vi "Cascade front panel.vi"() -> ()   [LabVIEW 2016]
uses:
  sdi_12/SDI-12/Sonde Vertical Graph.ctl
  controls/Vertical Chart.ctl
  sdi_12/Groundwater header.ctl
  controls/MCC DAQ Setup.ctl
  controls/Aux Sensor.ctl
  KPRO_2016 subvis/Control 2.ctl
  KPRO_2016 subvis/Graph Controls 2.ctl
  KPRO_2016 subvis/Ik control.ctl
  controls/MCC DAQ Readings.ctl
  controls/Kpro pressure measurement cluster.ctl
  controls/Kpro hydraulic measurement cluster.ctl
  activeXtest/activeXtest 2015 Folder/sonde cluster from excel.ctl
  sdi_12/Sonde Value Percent Tol.ctl
  activeXtest/activeXtest 2015 Folder/sample data row cluster.ctl
  activeXtest/activeXtest 2015 Folder/sonde cluster.ctl
  KPRO_2016 subvis/Sensor Physical Measurements.ctl
  KPRO_2016 subvis/SS Control 7.ctl
  controls/Action Control 1.ctl
  <extravilib>/ChannelInstances/One Element Stream-t'Action Control 1.ctl'/Instantiate.vi
  <extravilib>/ChannelInstances/One Element Stream-t'Action Control 1.ctl'/Endpoint.vi
  KPRO_lv2015/Kpro Globals.vi
  <vilib>/Utility/file.llb/Write Delimited Spreadsheet (string).vi
  C/Program Files (x86)/National Instruments/LabVIEW 2016/user.lib/_OpenG.lib/file/file.llb/Strip Path - Traditional__ogtk.vi
  C/Program Files (x86)/National Instruments/LabVIEW 2016/user.lib/_OpenG.lib/file/file.llb/Build Path - Traditional__ogtk.vi
  <vilib>/Utility/file.llb/Write Delimited Spreadsheet (DBL).vi
  C/Program Files (x86)/National Instruments/LabVIEW 2016/user.lib/_OpenG.lib/file/file.llb/Strip Path Extension - Path__ogtk.vi
  C/Program Files (x86)/National Instruments/LabVIEW 2016/user.lib/_OpenG.lib/file/file.llb/Convert File Extension (String)__ogtk.vi
  <vilib>/ULx/Create Channel.llb/ULx Create Channel (AI-Voltage-Basic).vi
  KPRO_lv2015/ad interface/Global_SIM_switch.vi
  C:/Program Files (x86)/National Instruments/LabVIEW 2016/vi.lib/ULx/ULx_LV.dll
  <vilib>/Utility/NIReport.llb/NI_report.lvclass
  <vilib>/Utility/config.llb/NI_LVConfig.lvlib
  <extravilib>/ChannelInstances/One Element Stream-t'Action Control 1.ctl'.lvlib
panel:
  out "output cluster":T1 caption="Cluster" {"Salinity" format="%_3g"; "Temp" format="%_2g"; "ORP" format="%_4g"; "pH" format="%_4g"; "Dissolved\nOxygen" format="%_3g"; "Specific\nConductance" format="%_4g"; "Cumulative\nVolume" format="%#_4g"}
  out "Serial Number/MISC":string
  in  "Depth mode":bool caption="Use \nIncrement"
  in  "Sample Sheet Data Row Cluster 2":T2={"Head\nPressure"=0.0, "Depth"=0.0, "comment string"="", "Sonde Data Cluster"={"Cumulative\nVolume"=100.0, "Specific\nConductance"=2.0, "Dissolved\nOxygen"=3.0, "pH"=4.0, "ORP"=5.0, "Temp"=26.0, "Salinity"=7.0}} {"Sonde Data Cluster"."Salinity" format="%_3g"; "Sonde Data Cluster"."Temp" format="%_2g"; "Sonde Data Cluster"."ORP" format="%_4g"; "Sonde Data Cluster"."pH" format="%_4g"; "Sonde Data Cluster"."Dissolved\nOxygen" format="%_4g"; "Sonde Data Cluster"."Specific\nConductance" format="%_4g"; "Sonde Data Cluster"."Cumulative\nVolume" format="%#_4g"; "Depth" format="%#.3g"; "Head\nPressure" format="%#.4g"}
  out "subarray":string[][](array[string])
  out "Initialization":i32
  in  "Increment Depth":bool
  in  "Finish Tests":bool
  in  "Start KPRO":bool
  in  "Record Continuous Samples":bool
  out "Current Time (s)":dbl
  in  "stop":bool
  in  "Write Data to Spreadsheet":bool
  in  "Sample Not Collected":bool
  in  "Record Single Sample":bool
  in  "Tab Control":T3(tab)
  out "KPRO Output File Path":path=path "C:/KPRO_2010/Output_files/Static Ik.txt"
  out "Output File Path":path=path "C:/KPRO_2010/Output_files/Static Ik.txt"
  in  "Slopes File Path":path=path "D:/Cascade/Data/Output Files/slopes.csv"
  out "12V Voltage Monitor":dbl format="%_3f"
  out "Found Quanta Sonde Com Port":refnum<visa-resource-name>
  in  "Temporary Data Files Directory":path=path "D:/Cascade/Data/Output Files"
  in  "Data File Directory":path=path "D:/Cascade/Data/Excel Reports"
  out "Quanta Sonde found?":bool
  in  "template file path":path=path "D:/Cascade/templates/Groundwater Profiling Log_empty_labview_template.xlsx"
  in  "Config File Path":path=path "D:/Cascade/Data/config files/DAQ Setup Config.ini"
  in  "Read Configuration File?":bool
  out "H-4191 Adapter found":bool
  in  "Save Configuration File?":bool
  out "Sonde Communication Error Out":errorcluster
  in  "Search for Comm Ports?":bool=TRUE
  in  "USB Serial Port Manual Entry":refnum<visa-resource-name>="COM13"
  in  "Static IK path":path=path "D:/Cascade/Data/Output Files/Static Ik.csv"
  out "Down hole Pressure Transducer CSV data  path 2":path
  out "appended path":path
  in  "Sonde Parameters \nTolerance Limits":T4 {"Salinity %" format="%_2f%%"; "Temp %" format="%_2f%%"; "ORP %" format="%_2f%%"; "pH %" format="%_2f%%"; "DO %" format="%_2f%%"; "SC %" format="%_2f%%"}
  in  "Sonde Parameters \nInitial Values":T5 {"Salinity Initial" format="%_2f"; "Temp Initial" format="%_2f"; "ORP  Initial" format="%_2f"; "pH Initial" format="%_2f"; "DO Initial" format="%_2f"; "SC Initial" format="%_2f"}
  in  "Header path":path=path "D:/Cascade/templates/Fields for Excel sheets.xlsx"
  out "Sensor  Real \nMeasurements":T6 {"9V Monitor" format="%#.3g"; "Aux 3" format="%#.3g"; "Aux 2" format="%#.3g"; "Aux 1" format="%#.3g"; "String Pot" format="%#.3g"; "Top String Pot" format="%#_4g"; "Downhole Pressure" format="%#_4g"; "Flow" format="%#_4g"; "Uphole Pressure" format="%#_4g"}
  in  "MCC USB-DAQ Setup":T7={"Device Name in InstaCal"="Dev0", "Omega Pressure Sensor"={"DAQ Channel"=2.0, "Output Voltage Range"=1, "Enabled"=TRUE, "Description"="Uphole Pressure"}, "McMillian 102 Flowmeter"={"DAQ Channel"=11.0, "Output Voltage Range"=0, "Enabled"=TRUE, "Description"="Flow"}, "DHT Pressure Sensor"={"DAQ Channel"=3.0, "Output Voltage Range"=1, "Enabled"=TRUE, "Description"="Downhole Pressure"}, "Top String Pot"={"DAQ Channel"=0.0, "Output Voltage Range"=0, "Enabled"=TRUE, "Description"="Top String Pot"}, "String Pot Signal"={"DAQ Channel"=1.0, "Output Voltage Range"=0, "Enabled"=TRUE, "Description"="String Pot"}, "Aux Sensor 1"={"DAQ Channel"=5.0, "Output Voltage Range"=1, "Enabled"=TRUE, "Description"="Aux 1"}, "Aux Sensor 2"={"DAQ Channel"=6.0, "Output Voltage Range"=1, "Enabled"=TRUE, "Description"="Aux 2"}, "Aux Sensor 3"={"DAQ Channel"=7.0, "Output Voltage Range"=1, "Enabled"=TRUE, "Description"="Aux 3"}, "Voltage Monitor"={"DAQ Channel"=8.0, "Output Voltage Range"=0, "Enabled"=TRUE, "Description"="9V Monitor"}} {"Voltage Monitor"."Output Voltage Range" items=["+/-10 V Range", "+/-5 V Range", "+/-2.5V Range", "+/-1.25 V Range", "+/-0.625 V Range", "+/-0.3125 V Range", "+/-0.1562V Range", "+/-0.078125 V Range"]; "Aux Sensor 3"."Output Voltage Range" items=["+/-10 V Range", "+/-5 V Range", "+/-2.5V Range", "+/-1.25 V Range", "+/-0.625 V Range", "+/-0.3125 V Range", "+/-0.1562V Range", "+/-0.078125 V Range"]; "Aux Sensor 2"."Output Voltage Range" items=["+/-10 V Range", "+/-5 V Range", "+/-2.5V Range", "+/-1.25 V Range", "+/-0.625 V Range", "+/-0.3125 V Range", "+/-0.1562V Range", "+/-0.078125 V Range"]; "Aux Sensor 1"."Output Voltage Range" items=["+/-10 V Range", "+/-5 V Range", "+/-2.5V Range", "+/-1.25 V Range", "+/-0.625 V Range", "+/-0.3125 V Range", "+/-0.1562V Range", "+/-0.078125 V Range"]; "String Pot Signal"."Output Voltage Range" items=["+/-10 V Range", "+/-5 V Range", "+/-2.5V Range", "+/-1.25 V Range", "+/-0.625 V Range", "+/-0.3125 V Range", "+/-0.1562V Range", "+/-0.078125 V Range"]; "Top String Pot"."Output Voltage Range" items=["+/-10 V Range", "+/-5 V Range", "+/-2.5V Range", "+/-1.25 V Range", "+/-0.625 V Range", "+/-0.3125 V Range", "+/-0.1562V Range", "+/-0.078125 V Range"]; "DHT Pressure Sensor"."Output Voltage Range" items=["+/-10 V Range", "+/-5 V Range", "+/-2.5V Range", "+/-1.25 V Range", "+/-0.625 V Range", "+/-0.3125 V Range", "+/-0.1562V Range", "+/-0.078125 V Range"]; "McMillian 102 Flowmeter"."Output Voltage Range" items=["+/-10 V Range", "+/-5 V Range", "+/-2.5V Range", "+/-1.25 V Range", "+/-0.625 V Range", "+/-0.3125 V Range", "+/-0.1562V Range", "+/-0.078125 V Range"]; "Omega Pressure Sensor"."Output Voltage Range" items=["+/-10 V Range", "+/-5 V Range", "+/-2.5V Range", "+/-1.25 V Range", "+/-0.625 V Range", "+/-0.3125 V Range", "+/-0.1562V Range", "+/-0.078125 V Range"]}
  out "Rate":dbl=1000.0 caption="Sample Rate (Hz)"
  out "Number \nof Channels":u16
  in  "Channel \nData Rate S/s":dbl=3720.0 format="%#_13g"
  out "Descriptions":string[](array[string])
  out "Raw Voltages":dbl[](array[numeric])
  out "9V Voltage Monitor":dbl format="%#_3g"
  in  "Record DAQ Raw Voltages":bool
  out "Sensor Voltage Cluster":T9 {"9V Monitor" format="%#.3g"; "Aux 3" format="%#_3g"; "Aux 2" format="%#.3g"; "Aux 1" format="%#.3g"; "String Pot" format="%#.3g"; "Top String Pot" format="%#_3g"; "Downhole Pressure" format="%#.3g"; "Flow" format="%#_3g"; "Uphole Pressure" format="%-#1.3g"}
  in  "Clear Groundwater Header Values":bool
  in  "Groundwater Header":T10
  out "Worksheet Names":string[](array[string])
  in  "Current Sheet":i32=1
  out "row max value":i32
  out "last occupied cell's name":string
  out "Current Sample Sheet":string="Sample 1"
  in  "Excel report file path":path=path "D:/Cascade/Data/Excel Reports/Groundwater Profiling Log_ara1.xlsx"
  out "Data Setup Indicator":string
  in  "Start Initialization":bool
  in  "Input Variables and Slopes":T11={"Total Volume"=0.0, "String Pot Slope"=1.6619999408721924, "Flow Slope"=39.040000915527344, "Up Hole Pressure Slope"=48.27000045776367, "Depth to Water Table"=-0.0, "Atmospheric Pressure"=32.22022530555725, "Reservoir Pressure"=-0.004827000045779073, "Height of Sample Box"=0.0, "DH Pressure Trans Slope"=42.0, "DH Pressure Offset"=0.0, "Up Hole  Pressure Offset"=0.0, "Aux 1 Slope"=1.0, "Aux 2 Slope"=1.0, "Aux 3 Slope"=1.0} {"Aux 3 Slope" format="%.2f"; "Aux 2 Slope" format="%.2f"; "Aux 1 Slope" format="%.2f"; "Up Hole  Pressure Offset" format="%.2f"; "DH Pressure Offset" format="%.2f"; "DH Pressure Trans Slope" format="%.2f"; "Height of Sample Box" format="%.2f"; "Reservoir Pressure" format="%.2f"; "Atmospheric Pressure" format="%.2f"; "Depth to Water Table" format="%.2f"; "Up Hole Pressure Slope" format="%.2f"; "Flow Slope" format="%.2f"; "String Pot Slope" format="%.2f"; "Total Volume" format="%.2f"}
  out "Pressure Offset":dbl
  in  "Update Sonde":bool
  out "Sonde Data Array":T12[](array[typedef]) {"Salinity"."%" format="%_2f%%"; "Salinity"."Value" format="%_4g"; "Temperature"."%" format="%_2f%%"; "Temperature"."Value" format="%_4g"; "ORP"."%" format="%_2f%%"; "ORP"."Value" format="%_4g"; "pH"."%" format="%_2f%%"; "pH"."Value" format="%_4g"; "Dissolved Oxygen"."%" format="%_2f%%"; "Dissolved Oxygen"."Value" format="%_4g"; "Sp. Conductance"."%" format="%_2f%%"; "Sp. Conductance"."Value" format="%_4g"; "Cumulative\nVolume" format="%#_4g"}
  out "Table Label":string="Data from Sample Sheet %d from Excel File"
  out "Sonde Data Display":T14
  out "Temperature":cluster{"Y":dbl[], "Y":dbl[]}[](graph)
  in  "Record Reason":bool
  in  "Select Reasons to Record Data":u16(ring) items=["Per Client Request", "Timed Out", "Sample stopped flowing", "Equipment Issue"]
  out "Sonde Recording Failure Path":path
  out "Sonde IK Behavior Path":path
  out "Recording Reason Sonde array":string[][](array[string])
  out "IK Reason array":string[][](array[string])
  out "SC  Reference\nCalibrate Response":bool
  out "DO  Reference\nCalibrate Response":bool
  in  "Salinity \nReference":dbl
  out "Salinity  Reference\nCalibrate Response":bool
  out "ORP  Reference\nCalibrate Response":bool
  in  "SC \nReference":dbl
  in  "DO \nReference":dbl
  in  "ORP Reference":dbl
  in  "pH Reference":dbl
  in  "pH Zero":dbl
  in  "Record  SC Calibration":bool
  in  "Record DO Calibration":bool
  in  "Record Salinity Calibration":bool
  in  "Record ORP Calibration":bool
  in  "Record pH Calibration Reference":bool
  in  "Record pH Calibration Zero":bool
  out "pH Zero \nCalibrate Response":bool
  out "pH  Reference\nCalibrate Response":bool
  out "KPRO Finish\nIndicator":bool
  in  "Input Depths \nand Parameters Cluster":T16={"Flow"=0.21081600494384767, "Zeroed \nPressure"=74.74207969932556, "Ik"=0.003788962123473114, "Current Depth"=-100.6, "Feet of Stainless"=40, "Start Depth"=0.0, "Abs Start Depth"=0.0} {"Abs Start Depth" format="%.2f"; "Start Depth" format="%.2f"; "Current Depth" format="%.2f"; "Ik" format="%.2f"; "Zeroed \nPressure" format="%.2f"; "Flow" format="%.2f"}
  out "Zero Pressure\nIndicator":bool
  in  "Zero\nPressure":bool caption="Zero Pressure"
  in  "enable_IKMGS_file":bool
  in  "enable_slug_file":bool
  in  "enable_kpro_file":bool=TRUE
  in  "Simulate AD6B":bool
  out "KPRO Test\nIndicator":bool
  in  "Record DTW File":bool
  in  "Zero In-Line Pressure\n(F = leave as is)":bool=TRUE
  out "Current Session":sgl[][](array[numeric]) format="%.2f"
  in  "KPRO test report header":string[](array[string])=["Time(msecs)", "Uncorrected Depth", "Corrected Depth", "Drive_Rate", "Flow", "Feet_of Stainless", "Up Hole Pressure", "IK", "Corrected Pressure", "Atm Pressure", "Depth to water", "Height of box", "Res_Pressure", "Secs_since_1_JAN_1904", "Depth jumps more than 1_foot", "Down hole Pressure"]
  in  "Depth Cluster":T17
  out "Cumulative_data_from_file":sgl[][](array[numeric]) format="%.2f"
  in  "KPRO test report header 2":string[](array[string])=["Time(msecs)", "Uncorrected Depth", "Corrected Depth", "Drive_Rate", "Flow", "Feet_of Stainless", "Up Hole Pressure", "IK", "Corrected Pressure", "Atm Pressure", "Depth to water", "Height of box", "Res_Pressure", "Secs_since_1_JAN_1904", "Depth jumps more than 1_foot", "Down hole Pressure"]
  out "Cumulative_data_ready":bool
  out "Depth Rate\nft/min":dbl format="%#.2g"
  out "Ik":dbl=0.003788962123473114 caption="Real Time - Depth vs. lk" format="%.2f"
  out "Uphole Pressure":dbl format="%.2f"
  in  "New Depth":dbl
  in  "Update Depth":bool
  in  "Select Entry for IK Log File":u16(ring) items=["IK Increase", "IK stayed the Same", "IK decreased"]
  out "Large Depth IK Graph Cluster":T18={[0.003788962123473114, 0.0037174584307500765, 0.0037174584307500765, 0.0037174584307500765, 0.0037174584307500765, 0.003788962123473114], [-100.1, -100.2, -100.3, -100.4, -100.5, -100.6]}
  in  "Culmulative Graph Cluster":T19={"Cumulative - Depth vs. Ik"={[], []}, "Real Time - Depth vs. lk "={[0.003788962123473114, 0.0037174584307500765, 0.0037174584307500765, 0.0037174584307500765, 0.0037174584307500765, 0.003788962123473114], [-100.1, -100.2, -100.3, -100.4, -100.5, -100.6]}, "Cumulative - Depth vs. Drive Rate"={[], []}, "Real Time - Depth vs. Drive Rate"={[0.02036245163917736, 0.125, 0.16666666666666674, 0.16666666666666663, 0.16666666666666663, 0.16666666666666663], [-100.1, -100.2, -100.3, -100.4, -100.5, -100.6]}}
  out "Down hole Pressure":dbl format="%.2f"
  in  "Record IK Reason":bool
  in  "Corrected Pressure Cluster":T20
  out "Flow":dbl format="%#.2g"
  out "Current Depth":sgl=-100.6 format="%.2f"
  out "Current \nDepth (m)":sgl=-30.661383 format="%.2f"
  in  "Read String Pot":bool
  out "Large Depth IK Graph":dbl(graph)
  out "DAQ Error":errorcluster
  out "Initialization Finished":bool=TRUE
  out "Stop":bool
  out "error out":errorcluster
  in  "error in (no error)":errorcluster
  out "producer loop":i32
  out "consumer loop":i32
  out "Active Channel Array":string[](array[string])
  out "delimited string":string
  out "Voltage Range":dbl[](array[numeric])
  out "Stop 2":bool
  # "ft. water"
  # "mL/min."
  # "ft. water"
  # "ft."
  # "ft."
  # "Instructions for Sonde Calibration:\n1.  Use the Record Single Point to Record the Data prior to start of\ncalibration procedure to record the initial points to the excel worksheet.\n2.  pH Calibration is a 2 step process:  A pH standard between 6.8 and 7.2 is treated as the “zero”\nand all other values are treated as the “slope”. First calibrate “zero”, then  add a second to calibrate “slope”. \n3.  Specific Conductance:  Wait for the specific conductance readings to stabilize in the calibration solution, which may\nrequire one or two minutes."
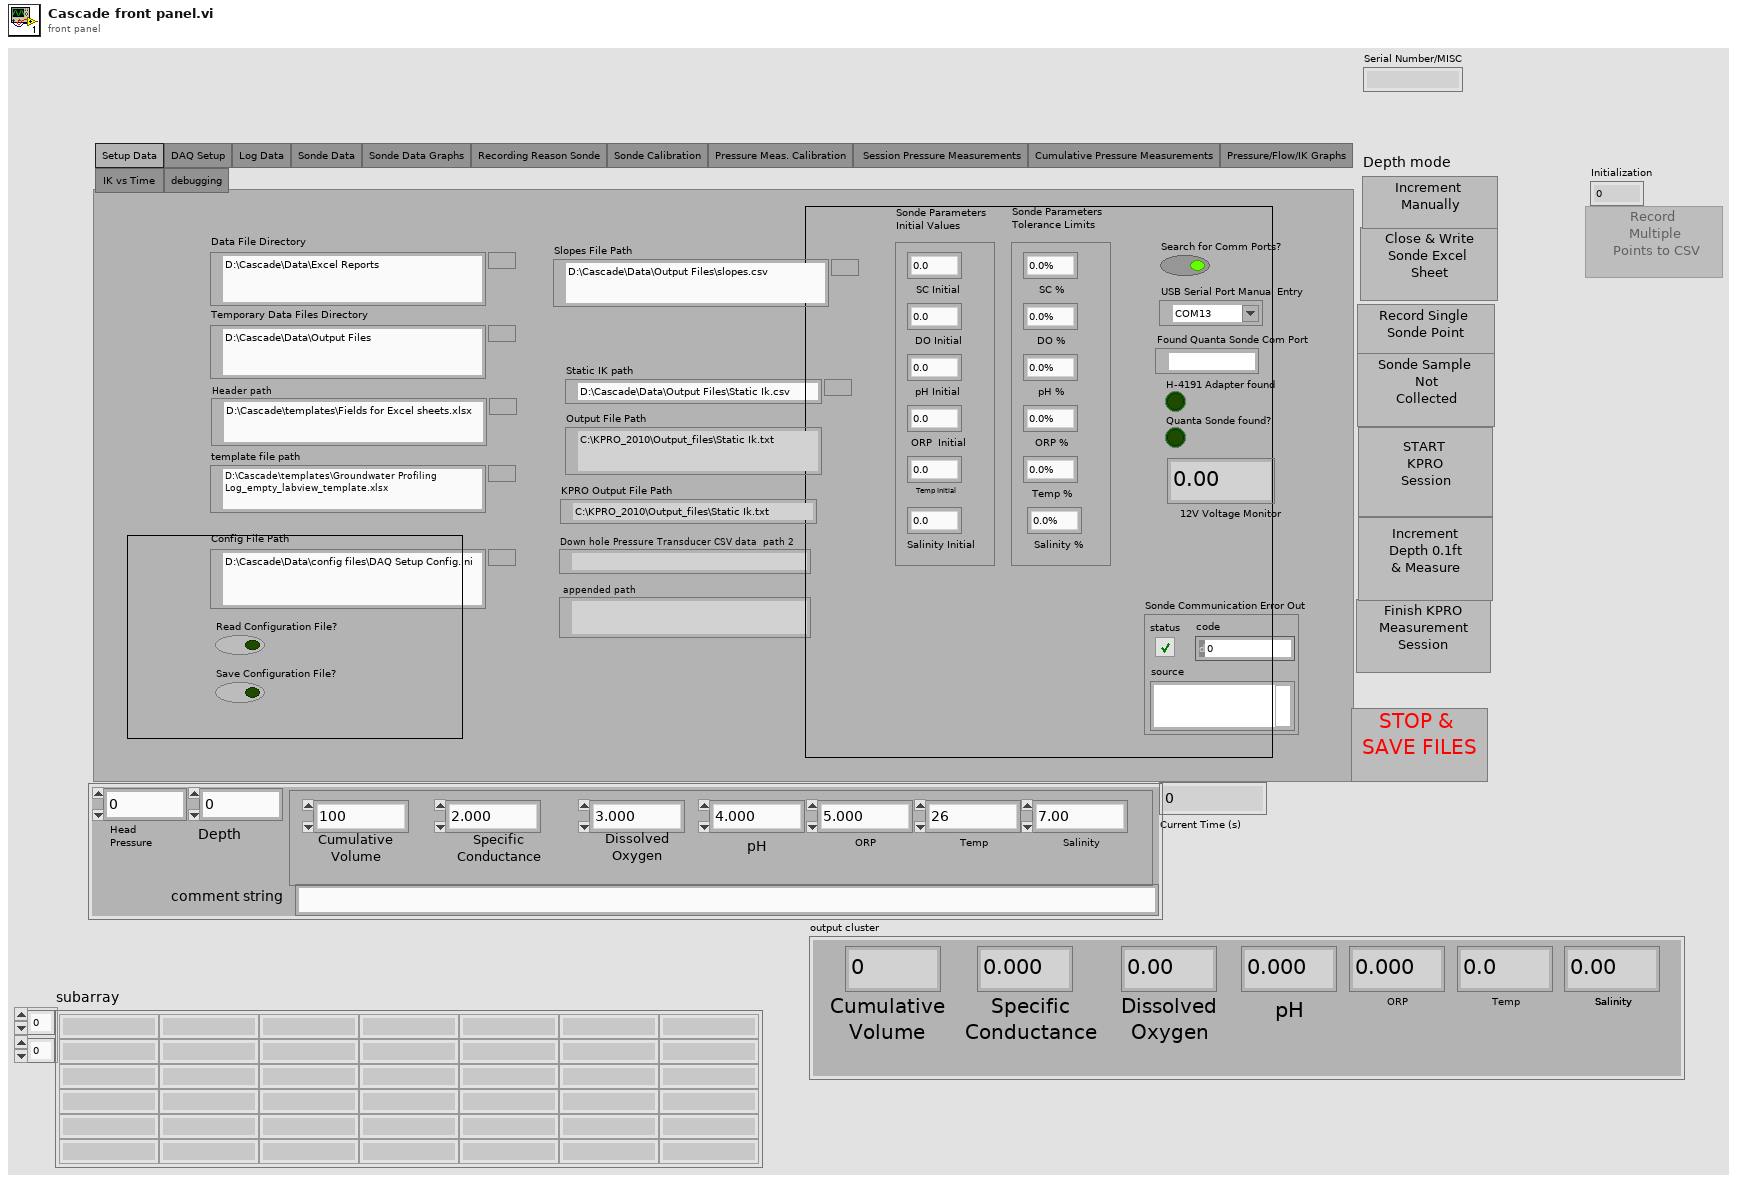
[diagram p1: front panel]
types:
  T1 = typedef "sonde cluster.ctl" = cluster{"Cumulative\nVolume":dbl, "Specific\nConductance":dbl, "Dissolved\nOxygen":dbl, "pH":dbl, "ORP":dbl, "Temp":dbl, "Salinity":dbl}
  T2 = typedef "sample data row cluster.ctl" = cluster{"Head\nPressure":dbl, "Depth":dbl, "comment string":string, "Sonde Data Cluster":T1}
  T3 = enum32{"Setup Data", "DAQ Setup", "Log Data", "Sonde Data", "Sonde Data Graphs", "Recording Reason Sonde", "Sonde Calibration", "Pressure Meas. Calibration", " Session Pressure Measurements", "Cumulative Pressure Measurements", "Pressure/Flow/IK Graphs", "IK vs Time ", "debugging"}
  T4 = cluster{"SC %":dbl, "DO %":dbl, "pH % ":dbl, "ORP % ":dbl, "Temp % ":dbl, "Salinity %":dbl}
  T5 = cluster{"SC Initial ":dbl, "DO Initial ":dbl, "pH Initial  ":dbl, "ORP  Initial":dbl, "Temp Initial":dbl, "Salinity Initial ":dbl}
  T6 = typedef "Sensor Physical Measurements.ctl" = cluster{"Uphole Pressure":dbl, "Flow":dbl, "Downhole Pressure":dbl, "Top String Pot":dbl, "String Pot":dbl, "Aux 1":dbl, "Aux 2":dbl, "Aux 3":dbl, "9V Monitor":dbl}
  T7 = typedef "MCC DAQ Setup.ctl" = cluster{"Device Name in InstaCal":string, "Omega Pressure Sensor":T8, "McMillian 102 Flowmeter":T8, "DHT Pressure Sensor":T8, "Top String Pot":T8, "String Pot Signal":T8, "Aux Sensor 1":T8, "Aux Sensor 2":T8, "Aux Sensor 3":T8, "Voltage Monitor":T8}
  T8 = typedef "Aux Sensor.ctl" = cluster{"DAQ Channel":dbl, "Output Voltage Range":u16, "Enabled":bool, "Description":string}
  T9 = typedef "MCC DAQ Readings.ctl" = cluster{"Uphole Pressure":dbl, "Flow":dbl, "Downhole Pressure":dbl, "Top String Pot":dbl, "String Pot":dbl, "Aux 1":dbl, "Aux 2":dbl, "Aux 3":dbl, "9V Monitor":dbl}
  T10 = typedef "Groundwater header.ctl" = cluster{"Location":string, "Date Finished":string, "CTS":string, "sampler":string, "Kpro box Serial ":string, "Sonde Serial":string, "Drilling Contractor":string, "Ave Depth to Water":string, "Gas/Peri Pump":string, "Atmospheric Pressure":string, "KPRO N2 Pressure":string, "Gas Drive N2 Pressure":string, "Profile ID":string}
  T11 = typedef "Control 2.ctl" = cluster{"Total Volume":dbl, "String Pot Slope":dbl, "Flow Slope":dbl, "Up Hole Pressure Slope":dbl, "Depth to Water Table":dbl, "Atmospheric Pressure":dbl, "Reservoir Pressure":dbl, "Height of Sample Box":dbl, "DH Pressure Trans Slope":dbl, "DH Pressure Offset":dbl, "Up Hole  Pressure Offset":dbl, "Aux 1 Slope":dbl, "Aux 2 Slope":dbl, "Aux 3 Slope":dbl}
  T12 = typedef "sonde cluster from excel.ctl" = cluster{"Head":dbl, "Depth":dbl, "Time":string, "Cumulative\nVolume":dbl, "Sp. Conductance":T13, "Dissolved Oxygen":T13, "pH":T13, "ORP":T13, "Temperature":T13, "Salinity":T13, "Final Tol.":bool, "Final":bool}
  T13 = typedef "Sonde Value Percent Tol.ctl" = cluster{"Value":dbl, "%":dbl, "Tol.":bool}
  T14 = typedef "Sonde Vertical Graph.ctl" = cluster{"pH":T15, "Conductance":T15, "Salinity":T15, "DO % Saturation":T15, "DO mg/L":T15, "ORP":T15}
  T15 = typedef "Vertical Chart.ctl" = cluster{"Y":dbl[], "Y":dbl[]}[]
  T16 = typedef "SS Control 7.ctl" = cluster{"Flow":dbl, "Zeroed \nPressure":dbl, "Ik":dbl, "Current Depth":sgl, "Feet of Stainless":i32, "Start Depth":sgl, "Abs Start Depth":sgl}
  T17 = typedef "Kpro hydraulic measurement cluster.ctl" = cluster{"Absolute Depth In":dbl, "Current Absolute Depth":dbl, "First Absolute Depth":dbl, "Previous Relative Depth":dbl, "Current Relative Depth":dbl, "First Relative Depth":dbl, "Last Filed Depth":dbl, "Total Volume In":dbl, "Total Volume Out":dbl, "Current Measurement Time":dbl, "Previous Measurement Time":dbl}
  T18 = typedef "Ik control.ctl" = cluster{dbl[], dbl[]}
  T19 = typedef "Graph Controls 2.ctl" = cluster{"Cumulative - Depth vs. Ik":cluster{dbl[], dbl[]}, "Real Time - Depth vs. lk ":cluster{dbl[], dbl[]}, "Cumulative - Depth vs. Drive Rate":cluster{dbl[], dbl[]}, "Real Time - Depth vs. Drive Rate":cluster{dbl[], dbl[]}}
  T20 = typedef "Kpro pressure measurement cluster.ctl" = cluster{"Up hole Corrected Pressure":dbl, "Down hole Corrected Pressure":dbl}
  T21 = enum16{"maximized", "minimized", "normal", "no change"}
  T22 = typedef "NI_LVConfig.lvlib/Config Data RefNum.ctl" = refnum<k1>
  T23 = enum8{"Enabled", "Disabled", "Disabled and Grayed Out"}
  T24 = typedef "Action Control 1.ctl" = enum16{"TimeOut", "Continuous  Sonde Data", "Init", "Exit", "Acq. Single Sonde Point", "Write Sonde Sample Sheet", "Acq. DAQ data", "Sample Not Collected", "Record Reason", "pH Calibration Zero", "pH Calibration Standard", "ORP Calibration Standard", "Salinity Calibration Standard", "DO Calibration Standard", "SC Calibration Standard", "Increment Depth Manually", "Start KPRO Measurements", "Finish KPRO Measurements", "Update Depth", "IK vs Time", "Record IK Reason"}
  T25 = typedef "One Element Stream-t'Action Control 1.ctl'.lvlib/)Channel.ctl" = refnum<queue>
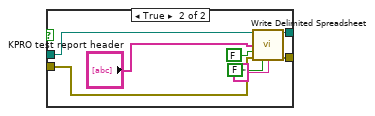
[diagram p11: hidden frame]
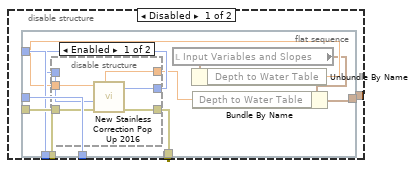
[diagram p18: hidden frame]
diagram:
  # "For calibrate command (XC) on SDI-12 address ‘a’, P is pH, C is specific conductance, S is\nsalinity or TDS, % is DO %Saturation, O is DO mg/L, R is ORP, D is depth, B is\nbarometric pressure, and t is TDS scale factor."
  n1 = flat-sequence {
    tunnel: [w20] -> w5
    tunnel: [w52] -> w7
    tunnel: w5 -> [w52]
    tunnel: [w48] -> w3
    tunnel: [w58] -> w14
    tunnel: w7 -> [w67]
    tunnel: [w67] -> w6
    tunnel: w14 -> [w93]
    tunnel: [w98] -> w12
    tunnel: [w100] -> w11
    tunnel: [w102] -> w8
    tunnel: [w95] -> w9
    tunnel: [w101] -> w10
    tunnel: [w99] -> _
    tunnel: [w94] -> w13
    tunnel: [w96] -> w2
    tunnel: [w97] -> w1
    frame #0 {
      n2 = invoke on="error out" class="Clust (strict)" method="Reinit To Default"(error in="error in (no error)") -> (error out=w18:errorcluster)  [unwired: 2 in, 2 out]
      n3 = flat-sequence {
        tunnel: [w24] -> w20
        tunnel: w18 -> [w23]
        frame #0 {
          n4 = case shown="True" "Read Configuration File?" {
            selector: "Read Configuration File?" -> [_ w31]
            tunnel: [w25 w36] -> w24
            tunnel: w23 -> [w25 w33]
            tunnel: "Config File Path" -> [_ w32]
            frame False {
            }
            frame True {
              n5 = call <vilib>:"Check if File or Folder Exists.vi"("error in (no error)"=w33, "path"=w32) -> ("error out"=w28:errorcluster, "file or folder exists?"=w29:bool, "dup path"=w27:path)  [unwired: 7 in]
              n6 = And(x=w31, y=w29) -> (x .and. y?=w30:bool)
              n7 = control-ref of="This VI"() -> (w34:refnum<vi>)
              n8 = case shown="True" w30 {
                selector: w30 -> [w37 _]
                tunnel: w27 -> [_ w42]
                tunnel: w28 -> [w38 w46]
                tunnel: [w38 w39] -> w35
                tunnel: w34 -> [_ w47]
                frame False {
                  n9 = local write "Read Configuration File?"(w37) -> ()
                }
                frame True {
                  n10 = call <vilib>:"Open Config Data.vi"("error in (no error)"=w46, "create file if necessary (T)"=FALSE, "configuration file path"=w42) -> ("error out"=w44:errorcluster, "refnum"=w45:T22)  [unwired: 6 in, 1 out]
                  n11 = call "Read Panel from INI__ogtk.vi"("error in (no error)"=w44, "VI ref"=w47, "refnum"=w45) -> ("error out"=w40:errorcluster, "refnum out"=w41:T22)  [unwired: 7 in]
                  n12 = call <vilib>:"Close Config Data.vi"("error in (no error)"=w40, "refnum"=w41) -> ("error out"=w39:errorcluster)  [unwired: 8 in, 1 out]
                }
              }
              n13 = call <vilib>:"Clear Errors.vi"("error in (no error)"=w35) -> ("error out"=w26:errorcluster)  [unwired: 5 in, 1 out]
              n14 = Merge Errors(w26) -> (w36:errorcluster)
            }
          }
        }
      }
    }
    frame #1 {
      n15 = local write "Current Sheet"(1 ("Current Sheet")) -> ()
      n16 = Get Date/Time In Seconds() -> (seconds since 1Jan1904=w48:timestamp)
      n17 = Get Date/Time In Seconds() -> (seconds since 1Jan1904=w49:timestamp)
      n18 = Subtract(x=w48, y=w49) -> (x-y=w50:dbl)
      n19 = To Double Precision Float(number=w50) -> (double precision float=→"Current Time (s)":dbl)
    }
    frame #2 {
      w54 = T23."Enabled" ("Disabled")
      w78 = T23."Disabled and Grayed Out" ("Disabled")
      n20 = local write "Initialization Finished"(FALSE ("Initialization Finished")) -> ()
      n21 = invoke on="Current Sheet" class="DigNum (strict)" method="Reinit To Default"() -> (error out=w71:errorcluster)  [unwired: 3 in, 2 out]
      n22 = invoke on="Sample Not Collected" class="Bool" method="Reinit To Default"(error in=w71) -> (error out=w75:errorcluster)  [unwired: 2 in, 2 out]
      n23 = invoke on="Record Continuous Samples" class="Bool" method="Reinit To Default"(error in=w75) -> (error out=w74:errorcluster)  [unwired: 2 in, 2 out]
      n24 = property on="Record Continuous Samples" class="Bool"("DisabledEnum"=w78) -> (error out=w79:errorcluster)  [unwired: 2 in, 1 out]
      n25 = invoke on="Write Data to Spreadsheet" class="Bool" method="Reinit To Default"(error in=w74) -> (error out=w73:errorcluster)  [unwired: 2 in, 2 out]
      n26 = call "search for Quanta Sonde devices.vi"("VISA resource name"="USB Serial Port Manual Entry", "Search for Comm Ports?"="Search for Comm Ports?", "error in (no error)"=w67) -> ("12V monitor"=→"12V Voltage Monitor":dbl, "Com Port with Quanta Sonde devices"=w84:refnum<visa-resource-name>[], "Number of Quanta Sonde devices"=w83:i32, "Serial Number/MISC"=w56:string, "Number of Quanta Sonde devices > 0?"=→"Quanta Sonde found?":bool, "H-4191 Adapter found"=→"H-4191 Adapter found":bool, "Error Out"=w64:errorcluster)  [unwired: 4 in, 2 out]
      "Sonde Communication Error Out" <- w64
      "Serial Number/MISC" <- w56
      n27 = local read "Groundwater Header"() -> (w55:T10)
      n28 = invoke on="Record Single Sample" class="Bool" method="Reinit To Default"(error in=w73) -> (error out=w72:errorcluster)  [unwired: 2 in, 2 out]
      n29 = case shown="1" w83 {
        tunnel: w84 -> [_ w91]
        tunnel: [refnum<visa-resource-name> refnum ("RS232 Port Out") w89] -> w82
        frame 0, Default {
        }
        frame 1 {
          n30 = Index Array(array=w91, index=0) -> (element=w89:refnum<visa-resource-name>)
        }
      }
      "Found Quanta Sonde Com Port" <- w82
      n31 = property on="Record Single Sample" class="Bool"(error in=w79, "DisabledEnum"=w78) -> (error out=w80:errorcluster)  [unwired: 1 in, 1 out]
      n32 = invoke on="stop" class="Bool" method="Reinit To Default"(error in=w72) -> (error out=w77:errorcluster)  [unwired: 2 in, 2 out]
      n33 = Bundle By Name(cluster=w55, "Sonde Serial"=w56) -> (w57:T10)
      n34 = invoke on="Stop" class="Bool (strict)" method="Reinit To Default"() -> (error out=w66:errorcluster)  [unwired: 3 in, 2 out]
      n35 = local write "Groundwater Header"(w57) -> ()
      n36 = property on="Write Data to Spreadsheet" class="Bool"(error in=w77, "DisabledEnum"=w78) -> (error out=w69:errorcluster)  [unwired: 1 in, 1 out]
      n37 = property on="Sample Not Collected" class="Bool"(error in=w80, "DisabledEnum"=w78) -> (error out=w76:errorcluster)  [unwired: 1 in, 1 out]
      n38 = invoke on="Stop 2" class="Bool (strict)" method="Reinit To Default"(error in=w66) -> (error out=w65:errorcluster)  [unwired: 2 in, 2 out]
      n39 = call <vilib>:"Clear Errors.vi"("error in (no error)"=w64) -> ("error out"=w63:errorcluster)  [unwired: 5 in, 1 out]
      n40 = Merge Errors(w63, w65, w69, w76) -> (w60:errorcluster)
      n41 = flat-sequence {
        tunnel: [w87] -> w59
        tunnel: w60 -> [w87]
        frame #0 {
          n42 = local write "Tab Control"(T3."Log Data" ("Tab Control")) -> ()
        }
      }
      n43 = invoke on="Current Session" class="Arr (strict)" method="Reinit To Default"() -> ()  [unwired: 3 in, 3 out]
      n44 = control-ref of="Sonde Data Display"() -> ()  [unwired: 1 out]
      n45 = property on="Clear Groundwater Header Values" class="Bool"("DisabledEnum"=w54) -> ()  [unwired: 2 in, 2 out]
      n46 = property on="Start Initialization" class="Bool"("DisabledEnum"=w54) -> ()  [unwired: 2 in, 2 out]
      n47 = invoke on="Data Setup Indicator" class="Str" method="Reinit To Default"(error in=w59) -> (error out=w58:errorcluster)  [unwired: 2 in, 2 out]
    }
    frame #3 {
      n48 = while {
        tunnel: w93 -> [w108]
        tunnel: [w105] -> w92
        tunnel: [w107] -> _
        i -> [w107]
        stop <- w110 stop-if-true
        n49 = event shown="[1] \"Start Initialization\": Value Change" {
          selector: _ -> [_ _ _]
          dyn-events: _ -> [_ _ _]
          timeout: 100 -> [_ _ _]
          tunnel: [FALSE w118 _] -> w110
          event Timeout {
            n50 = event-data() -> ()  [unwired: 1 in, 3 out]
          }
          event "Start Initialization": Value Change {
            n51 = event-data() -> ()  [unwired: 1 in, 3 out]
            n52 = case shown="True" "Start Initialization" {
              tunnel: [FALSE ("Stop") TRUE ("Stop")] -> w118
              frame False {
              }
              frame True {
                n53 = invoke on="Data Setup Indicator" class="Str" method="Reinit To Default"() -> ()  [unwired: 3 in, 3 out]
                n54 = invoke on="Start Initialization" class="Bool" method="Reinit To Default"() -> ()  [unwired: 3 in, 3 out]
              }
            }
          }
          event "Clear Groundwater Header Values": Value Change {
            n55 = event-data() -> ()  [unwired: 1 in, 6 out]
            n56 = case shown="True" "Clear Groundwater Header Values" {
              frame False {
              }
              frame True {
                n57 = invoke on="Groundwater Header" class="Clust (strict)" method="Reinit To Default"() -> (error out=w122:errorcluster)  [unwired: 3 in, 2 out]
                n58 = flat-sequence {
                  tunnel: w122 -> [_]
                  frame #0 {
                    n59 = local read "Groundwater Header"() -> (w123:T10)
                    n60 = local read "Serial Number/MISC"() -> (w124:string)
                    n61 = Bundle By Name(cluster=w123, "Sonde Serial"=w124) -> (w125:T10)
                    n62 = local write "Groundwater Header"(w125) -> ()
                  }
                }
              }
            }
          }
        }
        n63 = call "Wait (ms)__ogtk.vi"("error in (no error)"=w108, "milliseconds to wait"=u32 100) -> ("error out"=w105:errorcluster)  [unwired: 8 in, 1 out]
        n64 = Quotient & Remainder(x=w107, y=100) -> (floor(x/y)=w103:i32)  [unwired: 1 out]
        n65 = case shown="0" w103 {
          tunnel: w105 -> [w113 w115]
          frame 1, Default {
            n66 = property on="Data Setup Indicator" class="Str"(error in=w113, "Text.TextColor"=u32 0) -> ()  [unwired: 1 in, 2 out]
          }
          frame 0 {
            n67 = property on="Data Setup Indicator" class="Str"(error in=w115, "Text.TextColor"=u32 16716800) -> ()  [unwired: 1 in, 2 out]
          }
        }
        "Data Setup Indicator" <- "Hit the Start Key after Data Entry of Log Parameters and File Names." ("Data Setup Indicator")
      }
      n68 = invoke on="Sonde Data Array" class="Arr (strict)" method="Reinit To Default"() -> ()  [unwired: 3 in, 3 out]
      n69 = flat-sequence {
        tunnel: w92 -> [w146]
        tunnel: [w139] -> w102
        tunnel: [w138] -> w101
        tunnel: [w136] -> w100
        tunnel: [w135] -> w99
        tunnel: [w134] -> w98
        tunnel: [w133] -> w94
        tunnel: [w128] -> w95
        frame #0 {
          w126 = T23."Disabled and Grayed Out" ("Disabled")
          n70 = property on="Clear Groundwater Header Values" class="Bool"("DisabledEnum"=w126) -> ()  [unwired: 2 in, 2 out]
          n71 = property on="Start Initialization" class="Bool"("DisabledEnum"=w126) -> ()  [unwired: 2 in, 2 out]
          n72 = call "get sample header columns.vi"("report file path"="Header path", "error in (no error)"=w146) -> ("Column of Volume"=w128:i32, "Columns"=w138:i32[], "data"=w145:string[][], "error out"=w147:errorcluster)  [unwired: 4 in, 6 out]
          "row max value" <- w128
          n73 = call "format into Sonde Data Array.vi"("data"=w145) -> ()  [unwired: 10 in, 1 out]
          n74 = call "close excel file if open.vi"("error in (no error)"=w147, "report file path in"="Excel report file path") -> ("error out"=w140:errorcluster, "report file path out"=w132:path)  [unwired: 8 in]
          n75 = call "copy excel template.vi"("error in (no error)"=w140, "report file path in"=w132, "template file path in"="template file path") -> ("error out"=w141:errorcluster, "report file path out"=w143:path)  [unwired: 6 in, 1 out]
          n76 = call "open excel get worksheet names.vi"("window state (normal)"=T21."normal", "error in (no error)"=w141, "milliseconds to wait"=u32 5, "report file path"=w143) -> ("error out"=w129:errorcluster, "Number of Sample Sheets"=w139:i32, "NI_report out"=w130:refnum<class "NI_report.lvclass">, "Worksheet Names"=w136:string[])  [unwired: 2 in, 2 out]
          "Worksheet Names" <- w136
          n77 = flat-sequence {
            tunnel: w136 -> [w165]
            tunnel: [w163] -> w135
            tunnel: [w161] -> w134
            tunnel: [w159] -> w133
            tunnel: w130 -> [w158]
            tunnel: w129 -> [w157]
            frame #0 {
              w164 = "Sample 1" ("Worksheet Name in")
              n78 = local read "Current Sample Sheet"() -> (w150:string)
              n79 = call "find and open select worksheet.vi"("Worksheet Names"=w165, "error in (no error)"=w157, "milliseconds to wait"=u32 100, "Worksheet Name in"=w164, "NI_report in"=w158) -> ("error out"=w160:errorcluster, "Select Worksheet Index"=w163:i32, "NI_report out"=w162:refnum<class "NI_report.lvclass">)  [unwired: 4 in]
              n80 = local write "Current Sample Sheet"(w164) -> ()
              n81 = call "get sample sheet data cells.vi"("error in (no error)"=w160, "NI_report in"=w162) -> ("error out"=w153:errorcluster, "data"=w154:string[][], "NI_report out"=w161:refnum<class "NI_report.lvclass">, "left edge output cluster"=w152:cluster{"row":i32, "column":i32})  [unwired: 5 in, 1 out]
              n82 = call "find last occupied cell.vi"("data"=w154, "Active Sheet"=w150, "Header Rows to remove"=3, "sub array start"=w152, "error in (no error)"=w153) -> ("row max value"=w151:i32, "start of last occupied row"=w149:string, "error out"=w159:errorcluster)  [unwired: 4 in, 4 out]
              n83 = Array Subset(array=w154, index (col)=2 ("index")) -> (→"subarray":string[][])  [unwired: 3 in]
              n84 = local write "row max value"(w151) -> ()
              n85 = local write "last occupied cell's name"(w149) -> ()
            }
          }
        }
      }
      n86 = flat-sequence {
        tunnel: w94 -> [_]
        frame #0 {
          n87 = local write "KPRO Finish\nIndicator"(FALSE ("KPRO Finish\nIndicator")) -> ()
        }
      }
      n88 = flat-sequence {
        tunnel: [w169] -> w97
        tunnel: [w169] -> w96
        tunnel: [w174] -> _
        tunnel: w94 -> [w173]
        frame #0 {
          n89 = Unbundle By Name("Input Variables and Slopes") -> ("Depth to Water Table"=w179:dbl)
          n90 = Bundle By Name(cluster="Input Variables and Slopes", "Depth to Water Table"=w179) -> (w176:T11)
          n91 = call <vilib>:"Check if File or Folder Exists.vi"("error in (no error)"=w173, "path"="Slopes File Path") -> ("error out"=w172:errorcluster, "dup path"=w177:path)  [unwired: 7 in, 1 out]
          n92 = case shown="True" TRUE {
            tunnel: w177 -> [_ w190]
            tunnel: w176 -> [w183 w189]
            tunnel: [w183 w188] -> w175
            tunnel: w172 -> [w182 w184]
            tunnel: [w182 w184] -> w174
            frame False {
              n93 = local write "Data Setup Indicator"("Slope file not found." ("Data Setup Indicator")) -> ()
            }
            frame True {
              n94 = call "Get_SLOPE_data_from_file 2016.vi"("Slopes File Path"=w190) -> ("Last_Pressure_Slope"=w185:dbl, "Last_Flow_Slope"=w186:dbl, "Last_String_Pot_Slope"=w187:dbl)  [unwired: 7 in, 1 out]
              n95 = Bundle By Name(cluster=w189, "String Pot Slope"=w187, "Flow Slope"=w186, "Up Hole Pressure Slope"=w185) -> (w188:T11)
            }
          }
          n96 = local read "Input Depths \nand Parameters Cluster"() -> (w171:T16)
          n97 = Unbundle By Name(w171) -> ("Feet of Stainless"=w169:i32)
          n98 = Bundle By Name(cluster=w171, "Feet of Stainless"=w169) -> (w170:T16)
          n99 = local write "Input Depths \nand Parameters Cluster"(w170) -> ()
          n100 = local write "Input Variables and Slopes"(w175) -> ()
        }
      }
      n101 = invoke on="Update Sonde" class="Bool (strict)" method="Reinit To Default"() -> ()  [unwired: 3 in, 3 out]
    }
  }
  n102 = flat-sequence {
    tunnel: [w194] -> w17
    tunnel: w13 -> [w193]
    tunnel: [w192] -> w4
    frame #0 {
      w191 = Action_Control_1."Init"  # Event
      n103 = while {
        shift-right: [w202] -> w194
        shift-left: w193 -> [w202]
        shift-right: [w197] -> _
        shift-left: w191 -> [w195]
        tunnel: [w203] -> w192
        i -> [w201]
        stop <- w199 stop-if-true
        # "User Interface Producer Loop"
        n104 = First Call?() -> (First Call?: T/F=w196:bool)
        n105 = case shown="False" w196 {
          tunnel: w202 -> [w208 _]
          tunnel: [w206 FALSE ("Boolean")] -> w199
          tunnel: [w205 w392] -> w197
          tunnel: w195 -> [_ w392]
          frame False {
            w204 = Action_Control_1."TimeOut"  # Event
            n106 = event shown="[16] \"Record IK Reason\": Value Change" {
              selector: _ -> [_ _ _ _ _ _ _ _ _ _ _ _ _ _ _ _ _ _ _]
              dyn-events: _ -> [_ _ _ _ _ _ _ _ _ _ _ _ _ _ _ _ _ _ _]
              timeout: 100 -> [_ _ _ _ _ _ _ _ _ _ _ _ _ _ _ _ _ _ _]
              tunnel: [w209 w215 w221 w234 w246 w258 w270 w282 w294 w306 w319 w330 w340 w348 w356 w363 w372 w380 _] -> w205
              tunnel: [FALSE w214 w222 w235 w247 w259 w271 w283 w295 w307 w318 w329 w341 w349 w357 w364 w373 w381 _] -> w206
              tunnel: w208 -> [_ w212 w224 w237 w249 w261 w273 w285 w297 w309 _ w326 _ _ _ _ _ _ _]
              tunnel: [_ w212 w223 w236 w248 w260 w272 w284 w296 w308 _ _ _ _ _ _ _ _ _] -> _
              tunnel: w204 -> [w209 w211 w220 w233 w245 w257 w269 w281 w293 w305 w317 w324 w338 w346 w355 w362 w371 w379 _]
              event Timeout {
                n107 = event-data() -> ()  [unwired: 1 in, 3 out]
              }
              event "stop": Value Change {
                n108 = event-data() -> ()  [unwired: 1 in, 6 out]
                n109 = case shown="False" "stop" {
                  tunnel: [w216 w218] -> w215
                  tunnel: [FALSE TRUE] -> w214
                  tunnel: w211 -> [w216 _]
                  frame False {
                  }
                  frame True {
                    w218 = Action_Control_1."Exit"  # Event
                  }
                }
              }
              event "Record DAQ Raw Voltages": Value Change {
                n110 = event-data() -> ()  [unwired: 1 in, 6 out]
                n111 = case shown="False" "Record DAQ Raw Voltages" {
                  tunnel: [w226 w229] -> w221
                  tunnel: [FALSE FALSE ("Boolean")] -> w222
                  tunnel: [w227 w230] -> w223
                  tunnel: w224 -> [w227 w230]
                  tunnel: w220 -> [w226 _]
                  frame False {
                  }
                  frame True {
                    w229 = Action_Control_1."Acq. DAQ data"  # Event
                  }
                }
              }
              event "Record pH Calibration Zero": Value Change {
                n112 = event-data() -> ()  [unwired: 1 in, 6 out]
                n113 = case shown="True" "Record pH Calibration Zero" {
                  tunnel: [w238 w241] -> w234
                  tunnel: [FALSE FALSE ("Boolean")] -> w235
                  tunnel: [w239 w242] -> w236
                  tunnel: w237 -> [w239 w242]
                  tunnel: w233 -> [w238 _]
                  frame False {
                  }
                  frame True {
                    w241 = Action_Control_1."pH Calibration Zero"  # Event
                  }
                }
              }
              event "Record pH Calibration Reference": Value Change {
                n114 = event-data() -> ()  [unwired: 1 in, 6 out]
                n115 = case shown="True" "Record pH Calibration Reference" {
                  tunnel: [w250 w253] -> w246
                  tunnel: [FALSE FALSE ("Boolean")] -> w247
                  tunnel: [w251 w254] -> w248
                  tunnel: w249 -> [w251 w254]
                  tunnel: w245 -> [w250 _]
                  frame False {
                  }
                  frame True {
                    w253 = Action_Control_1."pH Calibration Standard"  # Event
                  }
                }
              }
              event "Record ORP Calibration": Value Change {
                n116 = event-data() -> ()  [unwired: 1 in, 6 out]
                n117 = case shown="True" "Record ORP Calibration" {
                  tunnel: [w262 w265] -> w258
                  tunnel: [FALSE FALSE ("Boolean")] -> w259
                  tunnel: [w263 w266] -> w260
                  tunnel: w261 -> [w263 w266]
                  tunnel: w257 -> [w262 _]
                  frame False {
                  }
                  frame True {
                    w265 = Action_Control_1."ORP Calibration Standard"  # Event
                  }
                }
              }
              event "Record Salinity Calibration": Value Change {
                n118 = event-data() -> ()  [unwired: 1 in, 6 out]
                n119 = case shown="True" "Record Salinity Calibration" {
                  tunnel: [w274 w277] -> w270
                  tunnel: [FALSE FALSE ("Boolean")] -> w271
                  tunnel: [w275 w278] -> w272
                  tunnel: w273 -> [w275 w278]
                  tunnel: w269 -> [w274 _]
                  frame False {
                  }
                  frame True {
                    w277 = Action_Control_1."Salinity Calibration Standard"  # Event
                  }
                }
              }
              event "Record DO Calibration": Value Change {
                n120 = event-data() -> ()  [unwired: 1 in, 6 out]
                n121 = case shown="True" "Record DO Calibration" {
                  tunnel: [w286 w289] -> w282
                  tunnel: [FALSE FALSE ("Boolean")] -> w283
                  tunnel: [w287 w290] -> w284
                  tunnel: w285 -> [w287 w290]
                  tunnel: w281 -> [w286 _]
                  frame False {
                  }
                  frame True {
                    w289 = Action_Control_1."DO Calibration Standard"  # Event
                  }
                }
              }
              event "Record  SC Calibration": Value Change {
                n122 = event-data() -> ()  [unwired: 1 in, 6 out]
                n123 = case shown="True" "Record  SC Calibration" {
                  tunnel: [w298 w301] -> w294
                  tunnel: [FALSE FALSE ("Boolean")] -> w295
                  tunnel: [w299 w302] -> w296
                  tunnel: w297 -> [w299 w302]
                  tunnel: w293 -> [w298 _]
                  frame False {
                  }
                  frame True {
                    w301 = Action_Control_1."SC Calibration Standard"  # Event
                  }
                }
              }
              event "Increment Depth": Value Change {
                n124 = event-data() -> ()  [unwired: 1 in, 6 out]
                n125 = case shown="True" "Increment Depth" {
                  tunnel: [w310 w313] -> w306
                  tunnel: [FALSE FALSE ("Boolean")] -> w307
                  tunnel: [w311 w314] -> w308
                  tunnel: w309 -> [w311 w314]
                  tunnel: w305 -> [w310 _]
                  frame False {
                  }
                  frame True {
                    w313 = Action_Control_1."Increment Depth Manually"  # Event
                  }
                }
              }
              event "Record Single Sample": Value Change {
                n126 = event-data() -> ()  [unwired: 1 in, 6 out]
                n127 = case shown="False" "Record Single Sample" {
                  tunnel: [w320 w322] -> w319
                  tunnel: [FALSE FALSE] -> w318
                  tunnel: w317 -> [w320 _]
                  frame False {
                  }
                  frame True {
                    w322 = Action_Control_1."Acq. Single Sonde Point"  # Event
                  }
                }
              }
              event "Write Data to Spreadsheet": Value Change {
                n128 = event-data() -> ("OldVal"=w328:bool, "NewVal"=w331:bool)  [unwired: 1 in, 4 out]
                n129 = Not(x=w328) -> (.not. x?=w327:bool)
                n130 = And(x=w327, y=w331) -> (x .and. y?=w325:bool)
                n131 = case shown="True" w325 {
                  tunnel: [w332 w335] -> w330
                  tunnel: [FALSE FALSE ("Boolean")] -> w329
                  tunnel: [w333 w336] -> _
                  tunnel: w326 -> [w333 w336]
                  tunnel: w324 -> [w332 _]
                  frame False {
                  }
                  frame True {
                    w335 = Action_Control_1."Write Sonde Sample Sheet"  # Event
                  }
                }
              }
              event "Sample Not Collected": Value Change {
                n132 = event-data() -> ("NewVal"=w339:bool)  [unwired: 1 in, 5 out]
                n133 = case shown="True" w339 {
                  tunnel: [FALSE FALSE] -> w341
                  tunnel: [w342 w344] -> w340
                  tunnel: w338 -> [_ w344]
                  frame True {
                    w342 = Action_Control_1."Sample Not Collected"  # Event
                  }
                  frame False {
                  }
                }
              }
              event "Record Reason": Value Change {
                n134 = event-data() -> ("NewVal"=w347:bool)  [unwired: 1 in, 5 out]
                n135 = case shown="True" w347 {
                  tunnel: [FALSE FALSE] -> w349
                  tunnel: [w350 w352] -> w348
                  tunnel: w346 -> [_ w352]
                  frame True {
                    w350 = Action_Control_1."Record Reason"  # Event
                  }
                  frame False {
                  }
                }
              }
              event "Start KPRO": Value Change {
                n136 = event-data() -> ()  [unwired: 1 in, 6 out]
                n137 = case shown="True" "Start KPRO" {
                  tunnel: [FALSE FALSE] -> w357
                  tunnel: [w358 w360] -> w356
                  tunnel: w355 -> [_ w360]
                  frame True {
                    w358 = Action_Control_1."Start KPRO Measurements"  # Event
                  }
                  frame False {
                  }
                }
              }
              event "Update Depth": Value Change {
                n138 = event-data() -> ()  [unwired: 1 in, 6 out]
                n139 = case shown="True" "Update Depth" {
                  tunnel: [FALSE FALSE] -> w364
                  tunnel: [w366 w368] -> w363
                  tunnel: w362 -> [_ w368]
                  frame True {
                    w366 = Action_Control_1."Update Depth"  # Event
                  }
                  frame False {
                  }
                }
              }
              event "Record IK Reason": Value Change {
                n140 = event-data() -> ()  [unwired: 1 in, 6 out]
                n141 = case shown="True" "Record IK Reason" {
                  tunnel: [FALSE FALSE] -> w373
                  tunnel: [w374 w376] -> w372
                  tunnel: w371 -> [_ w376]
                  frame True {
                    w374 = Action_Control_1."Record IK Reason"  # Event
                  }
                  frame False {
                  }
                }
              }
              event "Finish Tests": Value Change {
                n142 = event-data() -> ()  [unwired: 1 in, 6 out]
                n143 = case shown="True" "Finish Tests" {
                  tunnel: [FALSE FALSE] -> w381
                  tunnel: [w383 w385] -> w380
                  tunnel: w379 -> [_ w385]
                  frame True {
                    w383 = Action_Control_1."Finish KPRO Measurements"  # Event
                    "KPRO Finish\nIndicator" <- TRUE ("KPRO Finish\nIndicator")
                  }
                  frame False {
                  }
                }
              }
              event "Depth mode": Value Change {
                n144 = event-data() -> ()  [unwired: 1 in, 6 out]
                n145 = case shown="True" "Depth mode" {
                  tunnel: [FALSE ("Read String Pot") TRUE ("Read String Pot")] -> w387
                  frame False {
                  }
                  frame True {
                  }
                }
                n146 = local write "Read String Pot"(w387) -> ()
              }
            }
          }
          frame True {
          }
        }
        "Stop" <- w199
        n147 = local read "Stop"() -> (w200:bool)
        n148 = Or(x=w200, y=w199) -> ()  [unwired: 1 out]
        n149 = call <extravilib>:"Write With Abort.vi"("abort"=FALSE, "last element? (F)"=w199, "element"=w197) -> ("channel"=w203:T25)  [unwired: 6 in, 2 out]
        "producer loop" <- w201
      }
    }
  }
  n150 = flat-sequence {
    tunnel: [w418] -> w16
    tunnel: w13 -> [w417]
    tunnel: w12 -> [w416]
    tunnel: w11 -> [w414]
    tunnel: w10 -> [w412]
    tunnel: w9 -> [w411]
    tunnel: w8 -> [w409]
    tunnel: w6 -> [w408]
    tunnel: w4 -> [w407]
    tunnel: w3 -> [w405]
    tunnel: w2 -> [w404]
    tunnel: w1 -> [w403]
    frame #0 {
      w393 = dbl[][] []  # Cumulative Data over 1 string pot
      w397 = T5 {"SC Initial "=0.0, "DO Initial "=0.0, "pH Initial  "=0.0, "ORP  Initial"=0.0, "Temp Initial"=0.0, "Salinity Initial "=0.0}  # Sonde Parameters  Initial Values
      w398 = FALSE  # Read String Pot
      w399 = T16 {"Flow"=0.21081600494384767, "Zeroed \nPressure"=74.74207969932556, "Ik"=0.003788962123473114, "Current Depth"=-100.6, "Feet of Stainless"=40, "Start Depth"=0.0, "Abs Start Depth"=0.0}  # Input Depths  and Parameters Cluster
      w400 = T17 {"Absolute Depth In"=0.0, "Current Absolute Depth"=0.0, "First Absolute Depth"=0.0, "Previous Relative Depth"=0.0, "Current Relative Depth"=0.0, "First Relative Depth"=0.0, "Last Filed Depth"=0.0, "Total Volume In"=0.0, "Total Volume Out"=0.0, "Current Measurement Time"=0.0, "Previous Measurement Time"=0.0}  # Depth Cluster
      w401 = dbl[][] []  # Cumulative Data From File
      n151 = Get Date/Time In Seconds() -> (seconds since 1Jan1904=w396:timestamp)
      n152 = To Double Precision Float(number=w396) -> (double precision float=w395:dbl)
      n153 = while {
        tunnel: w417 -> [w472]
        tunnel: [w473] -> w418
        tunnel: w407 -> [w446]
        tunnel: w416 -> [w471]
        shift-right: [w459] -> _
        shift-left: "Current Sheet" -> [w465]
        tunnel: w414 -> [w461]
        tunnel: w412 -> [w469]
        tunnel: w411 -> [w468]
        shift-right: [w460] -> _
        shift-left: 0 ("row index") -> [w467]
        tunnel: [w466] -> _
        shift-right: [w464] -> _
        shift-left: cluster{"row":i32, "column":i32} {"row"=0, "column"=0} ("start of last occupied row") -> [w463]
        tunnel: w409 -> [w458]
        shift-right: [w452] -> _
        shift-left: dbl[] [] ("Time Array") -> [w453]
        shift-right: [w451] -> _
        shift-left: w401 -> [w450]
        tunnel: w395 -> [w449]
        tunnel: [w448] -> _
        tunnel: w408 -> [w433]
        shift-right: [w444] -> _
        shift-left: refnum<k24>[] [] -> [w432]
        tunnel: w405 -> [w442]
        shift-right: [w419] -> _
        shift-left: w404 -> [w428]
        shift-right: [w441] -> _
        shift-left: w403 -> [w441]
        shift-right: [w438] -> _
        shift-left: w398 -> [w437]
        shift-right: [w424] -> _
        shift-left: w400 -> [w436]
        shift-right: [w435] -> _
        shift-left: w399 -> [w434]
        shift-right: [w429] -> _
        shift-left: w397 -> [_]
        shift-right: [w426] -> _
        shift-left: dbl[][] [] ("Cumulative Sonde \nData Out") -> [w425]
        shift-right: [w423] -> _
        shift-left: w393 -> [w422]
        i -> [w430]
        stop <- w447 stop-if-true
        # "Consumer Data Handling Loop"
        n154 = flat-sequence {
          frame #0 {
            n155 = call "boolean debounce 2016.vi"() -> ()  [unwired: 1 in, 1 out]
          }
        }
        n156 = call <extravilib>:"Read With Abort.vi"("abort"=FALSE, "channel"=w446) -> ("last element?"=w445:bool, "element"=w455:T24)  [unwired: 5 in, 3 out]
        n157 = call "Wait (ms)__ogtk.vi"("error in (no error)"=w472, "milliseconds to wait"=u32 50) -> ("error out"=w457:errorcluster)  [unwired: 8 in, 1 out]
        n158 = feedback-in #1(w455) -> ()
        n159 = feedback #1() -> (w454:T24)  [unwired: 1 in]
        n160 = call "open select sample sheet.vi"("Number of Sample Sheets"=w458, "error in (no error)"=w457, "Worksheet Names"=w461, "Active Sample Sheet"=w465, "NI_report in"=w471) -> ("error out"=w440:errorcluster, "Current Sample Sheet"=w443:string, "NI_report out"=w470:refnum<class "NI_report.lvclass">)  [unwired: 3 in, 1 out]
        n161 = flat-sequence {
          tunnel: w443 -> [w494]
          tunnel: w442 -> [w489]
          tunnel: w440 -> [w488]
          tunnel: [w486] -> w439
          frame #0 {
            n162 = Get Date/Time In Seconds() -> (seconds since 1Jan1904=w490:timestamp)
            n163 = Subtract(x=w490, y=w489) -> (x-y=w491:dbl)
            n164 = local write "Current Time (s)"(w491) -> ()
            n165 = Scan From String(format string="Sample %d", input string=w494, error in=w488) -> (error out=w487:errorcluster, output 1=w492:i32)  [unwired: 2 in, 2 out]
            n166 = Format Into String(format string="Data from Sample Sheet %d from Excel File", error in=w487, w492) -> (resulting string=→"Table Label":string, error out=w486:errorcluster)  [unwired: 1 in]
            "Current Sample Sheet" <- w494
          }
        }
        n167 = disable-structure shown="Enabled" {
          disable-tunnel: w433 -> [w477 _]
          disable-tunnel: w432 -> [w476 w485]
          disable-tunnel: [w475 w485] -> w431
          disable-tunnel: w430 -> [w474 _]
          frame Enabled {
            n168 = case shown="1, Default" w474 {
              tunnel: w476 -> [w478 w484]
              tunnel: w477 -> [_ w483]
              tunnel: [w478 w481] -> w475
              frame 0 {
              }
              frame 1, Default {
                n169 = local read "Descriptions"() -> (w482:string[])
                n170 = call "Measure DAQ Voltages.vi"("error in (no error)"=w483, "Descriptions"=w482, "Array in"=w484) -> ("Raw Voltages"=w480:dbl[], "Array out"=w481:refnum<k24>[], "Sensor Cluster"=w479:T9)  [unwired: 6 in]
                n171 = local write "Sensor Voltage Cluster"(w479) -> ()
                n172 = local write "Raw Voltages"(w480) -> ()
              }
            }
          }
          frame Disabled {
          }
        }
        n173 = feedback #2() -> (w420:i32)  [unwired: 1 in]
        n174 = case shown="\"Start KPRO Measurements\"" w455 {
          selector: w455 -> [_ _ _ _ _ _ _ _ _ _ _ _ _ _ _ _ _ w1955 _ _ _]
          tunnel: w439 -> [w509 w661 w733 w755 w778 w926 w1118 w1135 w1174 w1222 w1257 w1335 w1438 w1542 w1646 w1750 w1853 w1961 w2040 w2418 w2435]
          tunnel: [w509 w661 w733 w755 w774 w921 w1118 w1135 w1174 w1221 w1255 w1333 w1436 w1540 w1644 w1748 w1851 w1944 w2040 w2418 w2445] -> w473
          tunnel: w445 -> [_ _ _ _ _ _ _ _ _ _ _ _ _ _ _ _ _ _ _ _ _]
          tunnel: w470 -> [w526 w647 w732 w754 w795 w946 w1117 w1134 w1173 w1216 w1269 w1353 w1456 w1560 w1664 w1768 w1871 w1962 w2047 w2417 w2436]
          tunnel: [w525 w660 w731 w753 w794 w945 w1116 w1133 w1172 w1215 w1253 w1330 w1433 w1537 w1641 w1745 w1848 w1949 w2046 w2416 w2450] -> w460
          tunnel: w469 -> [_ _ _ _ _ _ _ _ _ _ w1264 w1348 w1451 w1555 w1659 w1763 w1866 _ _ _ _]
          tunnel: w468 -> [_ _ _ _ _ _ _ _ _ _ w1263 w1347 w1450 w1554 w1658 w1762 w1865 _ _ _ _]
          tunnel: w467 -> [w525 w660 w731 w753 w794 w945 w1116 w1133 w1172 w1215 w1233 w1331 w1434 w1538 w1642 w1746 w1849 w1938 w2046 w2416 w2450]
          tunnel: [w526 w647 w732 w754 w795 w946 w1117 w1134 w1173 w1216 w1258 w1336 w1439 w1543 w1647 w1751 w1854 w1960 w2047 w2417 w2451] -> w466
          tunnel: w465 -> [w524 w659 w730 w752 w782 w930 w1115 w1132 w1171 w1214 w1231 w1344 w1447 w1551 w1655 w1759 w1862 w1957 w2045 w2415 w2449]
          tunnel: [w524 w659 w730 w752 w782 w930 w1115 w1132 w1171 w1214 w1231 w1344 w1447 w1551 w1655 w1759 w1862 w1956 w2045 w2415 w2449] -> w459
          tunnel: [w523 w658 w729 w751 w793 w944 w1114 w1131 w1170 w1213 w1254 w1332 w1435 w1539 w1643 w1747 w1850 w1952 w2044 w2414 w2448] -> w464
          tunnel: w463 -> [w523 w658 w729 w751 w793 w944 w1114 w1131 w1170 w1213 _ _ _ _ _ _ _ w1953 w2044 w2414 w2448]
          tunnel: w461 -> [_ _ _ _ _ _ _ _ _ _ _ _ _ _ _ _ _ w1959 _ _ _]
          tunnel: w458 -> [_ _ _ _ _ _ _ _ _ _ _ _ _ _ _ _ _ w1958 _ _ _]
          tunnel: w454 -> [_ _ _ _ _ _ _ _ _ _ _ _ _ _ _ _ _ w1954 _ _ _]
          tunnel: w453 -> [w508 w657 w728 w750 w792 w943 w1113 w1130 w1169 w1212 w1252 w1329 w1432 w1536 w1640 w1744 w1847 w1948 w2043 w2413 w2447]
          tunnel: [w507 w657 w728 w750 w792 w943 w1113 w1130 w1169 w1212 w1251 w1328 w1431 w1535 w1639 w1743 w1846 w1948 w2043 w2413 w2447] -> w452
          tunnel: [w502 w648 w727 w749 w780 w928 w1112 w1129 w1168 w1211 w1250 w1327 w1430 w1525 w1638 w1742 w1845 w1947 w2032 w2412 w2446] -> w451
          tunnel: w450 -> [w503 w648 w727 w749 w786 w935 w1112 w1129 w1168 w1211 w1249 w1326 w1429 w1525 w1637 w1741 w1844 w1947 w2033 w2412 w2446]
          tunnel: w449 -> [_ _ _ _ _ _ _ _ _ _ w1229 w1325 w1428 w1534 w1636 w1740 w1843 _ _ _ _]
          tunnel: w431 -> [w517 w656 w726 w748 w789 w940 w1111 w1128 w1167 w1210 w1247 w1323 w1426 w1532 w1634 w1738 w1841 w1946 _ w2410 w2440]
          tunnel: [w522 w655 w725 w747 w768 w920 w1110 w1127 w1166 w1209 w1248 w1324 w1427 w1533 w1635 w1739 w1842 w1945 w2039 _ w2441] -> w448
          tunnel: w433 -> [w522 w655 w725 w747 w769 w920 w1110 w1127 w1166 w1209 w1248 w1324 w1427 w1533 w1635 w1739 w1842 w1945 w2041 w2409 w2444]
          tunnel: [_ _ _ _ _ _ _ _ _ _ _ _ _ _ _ _ _ _ FALSE ("aborted?") FALSE ("aborted?") w2443] -> w447
          tunnel: [w513 w656 w726 w748 w789 w940 w1111 w1128 w1167 w1210 w1247 w1323 w1426 w1532 w1634 w1738 w1841 w1946 w2030 w2408 w2440] -> w444
          tunnel: [w521 w654 w724 w746 w791 w942 w1109 w1126 w1165 w1208 w1245 w1321 w1424 w1530 w1632 w1736 w1839 w1943 "Read String Pot" w2407 w2439] -> w438
          tunnel: w437 -> [w521 w654 w724 w746 w791 w942 w1109 w1126 w1165 w1208 w1245 w1321 w1424 w1530 w1632 w1736 w1839 w1943 _ w2407 w2439]
          tunnel: [w500 w649 w719 w742 w784 w932 w1108 w1125 w1164 w1207 w1244 w1320 w1423 w1529 w1631 w1735 w1838 w1942 w2036 w2406 w2438] -> w424
          tunnel: w436 -> [w501 w650 w720 w742 w760 w933 w1108 w1125 w1164 w1207 w1244 w1320 w1423 w1529 w1631 w1735 w1838 w1942 w2022 w2406 w2438]
          tunnel: [w520 w653 w723 w745 w790 w941 w1107 w1124 w1163 w1206 w1243 w1319 w1422 w1528 w1630 w1734 w1837 w1941 w2035 w2405 w2437] -> w435
          tunnel: w434 -> [w520 w653 w723 w745 w790 w941 w1107 w1124 w1163 w1206 w1243 w1319 w1422 w1528 w1630 w1734 w1837 w1941 _ w2405 w2437]
          tunnel: [w519 w652 w722 w744 w779 w927 w1106 w1123 w1162 w1205 w1227 w1318 w1421 w1527 w1629 w1733 w1836 w1940 w2026 w2404 w2432] -> w429
          tunnel: "Sonde Parameters \nInitial Values" -> [w519 w652 w722 w744 w779 w927 w1106 w1123 w1162 w1205 w1237 w1318 w1421 w1527 w1629 w1733 w1836 w1940 w2026 w2404 w2432]
          tunnel: w428 -> [w518 w651 w721 w743 w777 w925 w1105 w1122 w1161 w1204 w1236 w1317 w1420 w1526 w1628 w1732 w1835 w1939 w2025 w2403 w2431]
          tunnel: [w518 w651 w721 w743 w762 w924 w1105 w1122 w1161 w1204 w1236 w1317 w1420 w1526 w1628 w1732 w1835 w1939 w2025 w2403 w2431] -> w421
          tunnel: [w506 w646 w718 w741 w761 w918 w1104 w1121 w1160 w1203 w1228 w1316 w1419 w1524 w1627 w1731 w1834 w1937 w2023 w2402 w2430] -> w426
          tunnel: w425 -> [w505 w646 w718 w741 w761 w918 w1104 w1121 w1160 w1203 w1228 w1316 w1419 w1523 w1627 w1731 w1834 w1937 w2023 w2402 w2430]
          tunnel: [w498 w645 w717 w740 w757 w917 w1103 w1120 w1159 w1202 w1226 w1315 w1418 w1522 w1626 w1730 w1833 w1936 w2020 w2401 w2429] -> w423
          tunnel: w422 -> [w499 w645 w717 w740 w758 w916 w1103 w1120 w1159 w1202 w1226 w1315 w1418 w1522 w1626 w1730 w1833 w1936 w2020 w2401 w2429]
          tunnel: w420 -> [w497 w643 w716 w739 w756 w915 w1101 w1119 w1158 w1201 w1225 w1314 w1417 w1521 w1625 w1729 w1832 w1935 w2019 w2400 w2428]
          tunnel: [w497 w642 w716 w739 w756 w915 w1101 w1119 w1158 w1201 w1225 w1314 w1417 w1521 w1625 w1729 w1832 w1935 w2019 w2400 w2428] -> w419
          frame "TimeOut", Default {
            n175 = flat-sequence {
              tunnel: [w628] -> _
              tunnel: [w633] -> w510
              tunnel: [w641] -> _
              tunnel: [w640] -> _
              tunnel: w517 -> [w639]
              tunnel: [w638] -> _
              frame #0 {
                n176 = local read "Input Variables and Slopes"() -> (w630:T11)
                n177 = local read "Input Variables and Slopes"() -> (w635:T11)
                n178 = local read "Zero In-Line Pressure\n(F = leave as is)"() -> (w634:bool)
                n179 = Unbundle By Name(w635) -> ("DH Pressure Trans Slope"=w641:dbl, "DH Pressure Offset"=w640:dbl)
                n180 = local read "Sensor Voltage Cluster"() -> (w636:T9)
                n181 = local read "Descriptions"() -> (w637:string[])
                n182 = local read "Sensor  Real \nMeasurements"() -> (w632:T6)
                n183 = global read "Kpro Globals.vi" "Current Depth"() -> (w628:sgl)
                n184 = call "DHT Pressure 2016.vi"("Sensor Cluster"=w636, "DHT Pressure Offset"=w640, "Array in"=w639, "DHT Pressure \nSlope"=w641, "Descriptions"=w637, "Zero Pressure\n(F = leave as is)"=w634) -> ("Array out"=w638:refnum<k24>[], "DHT Pressure"=w633:dbl, "Sensor Cluster 2"=w629:T9)  [unwired: 7 in]
                n185 = local write "Sensor Voltage Cluster"(w629) -> ()
                n186 = call "convert sensor voltage to real measurements.vi"("Input Variables and Slopes"=w630, "Sensor  Real Measurements in"=w632, "Sensor Cluster"=w629) -> ("Sensor  Real Measurements out"=w631:T9)  [unwired: 8 in]
                n187 = local write "Sensor  Real \nMeasurements"(w631) -> ()
                n188 = local write "Down hole Pressure"(w633) -> ()
                n189 = Add(x=w633, y=w628) -> ()  [unwired: 1 out]
              }
            }
            n190 = case shown="True" "Update Sonde" {
              tunnel: w508 -> [w528 w535]
              tunnel: [w528 w534] -> w507
              tunnel: [w527 w533] -> w506
              tunnel: w505 -> [w527 w532]
              frame False {
              }
              frame True {
                n191 = local read "Sonde Communication Error Out"() -> (w531:errorcluster)
                n192 = local read "Current Time (s)"() -> (w529:dbl)
                n193 = flat-sequence {
                  tunnel: w531 -> [w553]
                  tunnel: [w552] -> w530
                  tunnel: w535 -> [w551]
                  tunnel: [w550] -> w534
                  tunnel: [w549] -> w533
                  tunnel: w532 -> [w548]
                  tunnel: [w538] -> _
                  tunnel: [w547] -> _
                  tunnel: w529 -> [w546]
                  frame #0 {
                    n194 = local read "Sample Sheet Data Row Cluster 2"() -> (w539:T2)
                    n195 = control-ref of="Found Quanta Sonde Com Port"() -> (w545:refnum<vi>)
                    n196 = control-ref of="Current Time (s)"() -> (w541:refnum<vi>)
                    n197 = control-ref of="Sonde Data Display"() -> (w544:refnum<vi>)
                    n198 = control-ref of="Sonde Data Display"() -> (w543:refnum<vi>)
                    n199 = control-ref of="Temperature"() -> (w542:refnum<vi>)
                    n200 = Unbundle By Name(w539) -> ("Sonde Data Cluster.Cumulative\nVolume"=w536:dbl)
                    n201 = call "Sonde Single Measurement Subvi.vi"("VISAResourceName in"=w545, "Time Array"=w551, "Cumulative Sonde Data"=w548, "Previous time"=w546, "Sonde Data Display"=w544, "Sonde Graph in"=w543, "Temp Graph 3"=w542, "error in (no error)"=w553, "Row Cluster Input"=w539, "reference 5"=w541) -> ("seconds since 1Jan1904"=w547:timestamp, "Cumulative Sonde \nData Out"=w549:dbl[][], "Sample Sheet Data Row Cluster 2"=w538:T2, "output cluster"=w540:T1, "time array out"=w550:dbl[], "error out"=w552:errorcluster)
                    n202 = Bundle By Name(cluster=w538, "Sonde Data Cluster.Cumulative\nVolume"=w536) -> (w537:T2)
                    n203 = local write "Sample Sheet Data Row Cluster 2"(w537) -> ()
                    n204 = local write "output cluster"(w540) -> ()
                  }
                }
                n205 = local write "Sonde Communication Error Out"(w530) -> ()
              }
            }
            n206 = flat-sequence {
              tunnel: w517 -> [w622]
              tunnel: [w618] -> w516
              tunnel: [w617] -> w515
              frame #0 {
                n207 = local read "Input Variables and Slopes"() -> (w625:T11)
                n208 = Unbundle By Name(w625) -> ("Up Hole Pressure Slope"=w624:dbl, "Up Hole  Pressure Offset"=w621:dbl)
                n209 = local write "Input Variables and Slopes"(w625) -> ()
                n210 = local read "Sensor Voltage Cluster"() -> (w626:T9)
                n211 = local read "Descriptions"() -> (w618:string[])
                n212 = local read "Corrected Pressure Cluster"() -> (w620:T20)
                n213 = call "up hole Pressure 2016.vi"("Sensor Cluster"=w626, "Pressure Offset"=w621, "Array in"=w622, "Pressure \nSlope"=w624, "Descriptions"=w618, "Zero Pressure\n(F = leave as is)"=TRUE) -> ("Array out"=w617:refnum<k24>[], "Uphole Pressure"=w616:dbl, "Sensor Cluster 2"=w623:T9)  [unwired: 7 in]
                n214 = local write "Uphole Pressure"(w616) -> ()
                n215 = Bundle By Name(cluster=w620, "Up hole Corrected Pressure"=w616) -> (w619:T20)
                n216 = local write "Sensor Voltage Cluster"(w623) -> ()
                n217 = local write "Corrected Pressure Cluster"(w619) -> ()
              }
            }
            n218 = flat-sequence {
              tunnel: w516 -> [w609]
              tunnel: w515 -> [w612]
              tunnel: [w608] -> w512
              tunnel: [w609] -> w514
              tunnel: [w605] -> w511
              tunnel: [w607] -> w513
              frame #0 {
                w613 = 0.0  # Offset
                n219 = local read "Input Variables and Slopes"() -> (w611:T11)
                n220 = local read "Input Depths \nand Parameters Cluster"() -> (w604:T16)
                n221 = Unbundle By Name(w611) -> ("Flow Slope"=w610:dbl)
                n222 = local read "Input Depths \nand Parameters Cluster"() -> (w615:T16)
                n223 = Unbundle By Name(w604) -> ("Feet of Stainless"=w603:i32)
                n224 = call "Flow 2016.vi"("Descriptions"=w609, "Array in"=w612, "Flow Slope"=w610, "Offset"=w613) -> ("Sensor Cluster"=w608:T9, "Flow (ml/min)"=w605:dbl, "Array out"=w607:refnum<k24>[])  [unwired: 4 in]
                n225 = local write "Sensor Voltage Cluster"(w608) -> ()
                n226 = call "pressure and IK2 2016.vi"("Ft. of SS"=w603, "flow"=w605) -> ("IK"=→"Large Depth IK Graph":dbl)  [unwired: 1 in, 1 out]
                n227 = Bundle By Name(cluster=w615, "Flow"=w605) -> (w614:T16)
                n228 = local write "Input Depths \nand Parameters Cluster"(w614) -> ()
              }
            }
            n229 = flat-sequence {
              tunnel: w514 -> [w591]
              tunnel: w503 -> [w564]
              tunnel: w512 -> [w590]
              tunnel: w501 -> [w569]
              tunnel: [w589] -> w500
              tunnel: w511 -> [w588]
              tunnel: w513 -> [w579]
              tunnel: [w578] -> _
              tunnel: [w556] -> w502
              tunnel: [w570] -> _
              tunnel: w510 -> [w561]
              tunnel: w509 -> [w558]
              tunnel: w499 -> [w557]
              tunnel: [w554] -> w498
              frame #0 {
                # "Timeout"
                n230 = Unbundle By Name(w569) -> ("Current Relative Depth"=w568:dbl)
                n231 = local read "Input Depths \nand Parameters Cluster"() -> (w583:T16)
                n232 = local read "Culmulative Graph Cluster"() -> (w577:T19)
                n233 = local read "Depth mode"() -> (w566:bool)
                n234 = local read "Input Variables and Slopes"() -> (w587:T11)
                n235 = local read "KPRO Finish\nIndicator"() -> (w563:bool)
                n236 = local read "KPRO Output File Path"() -> (w570:path)
                n237 = Unbundle By Name(w583) -> ("Feet of Stainless"=w585:i32, "Zeroed \nPressure"=w584:dbl)
                n238 = Unbundle By Name(w587) -> ("String Pot Slope"=w586:dbl)
                n239 = call "Kpro Read String Pot 2016.vi"("Read String Pot"=w566, "Feet of\nStainless to be\nUsed (Count) in"=w585, "Session Array in"=w557, "Flow"=w588, "Manual Depth In"=w568, "Finished In"=w563, "Depth Cluster in"=w569, "error in (no error)"=w558, "String Pot \nSlope in"=w586, "Sensor Cluster In in"=w590, "Descriptions"=w591, "Pressure in"=w584, "Array in"=w579, "Downhole Pressure Sensor"=w561) -> ("Sensor Cluster 2"=w580:T9, "IK"=w560:dbl, "Array out"=w578:refnum<k24>[], "Generate Array Calc IK"=w565:bool, "Feet of\nStainless to be\nUsed (Count) out"=w581:i32, "Depth Cluster out"=w589:T17, "Single String Pot Session Array out"=w554:dbl[][])  [unwired: 5 in, 2 out]
                n240 = local write "Ik"(w560) -> ()
                n241 = local write "Sensor Voltage Cluster"(w580) -> ()
                n242 = Unbundle By Name(w589) -> ("Current Absolute Depth"=w567:dbl)
                n243 = And(x=w565, y=w566) -> ()  [unwired: 1 out]
                n244 = Bundle By Name(cluster=w583, "Feet of Stainless"=w581) -> (w582:T16)
                n245 = local write "Input Depths \nand Parameters Cluster"(w582) -> ()
                n246 = flat-sequence {
                  tunnel: w567 -> [w597]
                  frame #0 {
                    n247 = global write "Kpro Globals.vi" "Current Depth"(w597) -> ()
                    n248 = local write "Current Depth"(w597) -> ()
                    n249 = Divide(x=w597, y=3.281) -> (x/y=w598:dbl)
                    n250 = local read "Sample Sheet Data Row Cluster 2"() -> (w601:T2)
                    n251 = local read "Corrected Pressure Cluster"() -> (w599:T20)
                    n252 = Unbundle By Name(w599) -> ("Up hole Corrected Pressure"=w596:dbl)
                    "Uphole Pressure" <- w596
                    n253 = Bundle By Name(cluster=w601, "Depth"=w597, "Head\nPressure"=w596) -> (w600:T2)
                    n254 = local write "Sample Sheet Data Row Cluster 2"(w600) -> ()
                    n255 = local write "Current \nDepth (m)"(w598) -> ()
                  }
                }
                n256 = case shown="True" FALSE {
                  tunnel: w564 -> [w592 w595]
                  tunnel: w554 -> [_ w593]
                  tunnel: [w592 w594] -> w556
                  frame False {
                  }
                  frame True {
                    n257 = Build Array (concatenate)(w595, w593) -> (w594:dbl[][])
                  }
                }
                n258 = call "Array to Plot 2016.vi"("Input Cumulative Array"=w556, "Input Real Time Array"=w554) -> ("Cumulative - Depth vs.Drive Rate"=w573:cluster{dbl[], dbl[]}, "Cumulative - Depth vs. Ik"=w575:cluster{dbl[], dbl[]}, "Real Time - Depth vs. Drive Rate"=w574:cluster{dbl[], dbl[]}, "Real Time - Depth vs. Ik"=w562:cluster{dbl[], dbl[]}, "Depth Rate"=w559:dbl)  [unwired: 2 in, 1 out]
                n259 = Bundle By Name(cluster=w577, "Cumulative - Depth vs. Ik"=w575, "Real Time - Depth vs. lk"=w562, "Cumulative - Depth vs. Drive Rate"=w574, "Real Time - Depth vs. Drive Rate"=w573) -> (w576:T19)
                n260 = local write "Large Depth IK Graph Cluster"(w562) -> ()
                n261 = local write "Culmulative Graph Cluster"(w576) -> ()
                n262 = local write "Depth Rate\nft/min"(w559) -> ()
                n263 = local write "Current Session"(w554) -> ()
                n264 = local read "Input Depths \nand Parameters Cluster"() -> (w572:T16)
                n265 = local write "Cumulative_data_from_file"(w556) -> ()
                n266 = Unbundle By Name(w572) -> ("Flow"=→"Flow":dbl)
              }
            }
          }
          frame "Finish KPRO Measurements" {
            n267 = flat-sequence {
              tunnel: w650 -> [w705]
              tunnel: [w704] -> w644
              tunnel: [w701] -> w649
              tunnel: w648 -> [w699]
              tunnel: w645 -> [w693]
              tunnel: w643 -> [w692]
              tunnel: [w691] -> w642
              frame #0 {
                n268 = local read "Input Depths \nand Parameters Cluster"() -> (w703:T16)
                n269 = Unbundle By Name(w703) -> ()  [unwired: 1 out]
                n270 = Build Array (concatenate)(w699, w693) -> (w694:dbl[][])
                n271 = local read "KPRO Output File Path"() -> (w697:path)
                n272 = case shown="False" TRUE {
                  tunnel: w697 -> [w706 w715]
                  tunnel: errorcluster {"status"=FALSE, "code"=0, "source"=""} ("error constant") -> [w707 w712]
                  tunnel: [w707 w711] -> _
                  tunnel: [w706 w708] -> w696
                  frame False {
                  }
                  frame True {
                    n273 = call-poly <vilib>:"Write Delimited Spreadsheet.vi"("file path (dialog if empty)"=w715, "1D data"="KPRO test report header", "append to file? (new file:F)"=FALSE, "error in (no error)"=w712, "transpose? (no:F)"=FALSE, "delimiter (\\t)"="," ("delimiter (\\t)")) -> ("new file path (Not A Path if cancelled)"=w708:path, "error out"=w711:errorcluster)  [unwired: 8 in]
                  }
                }
                n274 = call "Finished Collection Write File.vi"("Cluster in"=w705, "Corrected Array in"=w694, "Feet of\nStainless to be\nUsed (Count) in"=w692, "Output KPRO"=w696) -> ("Corrected Array out"=w704:dbl[][], "Depth to \nbe Used \n(Feet)"=w700:sgl, "Feet of\nStainless to be\nUsed (Count) out"=w691:i32)  [unwired: 5 in]
                n275 = Bundle By Name(cluster=w705, "Absolute Depth In"=w700) -> (w701:T17)
                n276 = Bundle By Name(cluster=w703, "Feet of Stainless"=w691) -> (w702:T16)
                n277 = local write "Input Depths \nand Parameters Cluster"(w702) -> ()
              }
            }
            n278 = flat-sequence {
              tunnel: w644 -> [w689]
              frame #0 {
                n279 = control-ref of="KPRO Output File Path"() -> (w687:refnum<vi>)
                n280 = call "write KPRO file.vi"("Corrected Array in"=w689, "Generate Array Calc IK"=TRUE, "Path in"=w687) -> ("paths ok"=w686:bool, "appended path"=w685:path)  [unwired: 7 in]
                n281 = case shown="True" w686 {
                  tunnel: w685 -> [_ w690]
                  frame False {
                  }
                  frame True {
                    n282 = local write "KPRO Output File Path"(w690) -> ()
                  }
                }
              }
            }
            n283 = disable-structure shown="Disabled" {
              disable-tunnel: w647 -> [w665 _]
              disable-tunnel: w644 -> [_ _]
              frame Disabled {
                n284 = disable-structure shown="Disabled" {
                  disable-tunnel: w665 -> [w670 _]
                  disable-tunnel: [w669 _] -> w664
                  disable-tunnel: [w668 _] -> w663
                  disable-tunnel: [w667 _] -> w662
                  frame Disabled {
                    n285 = call "open select sample sheet.vi"("Active Sample Sheet"=0, "NI_report in"=w670) -> ("error out"=w669:errorcluster, "Current Sample Sheet"=w668:string, "NI_report out"=w667:refnum<class "NI_report.lvclass">)  [unwired: 6 in, 1 out]
                  }
                  frame Enabled {
                  }
                }
                n286 = flat-sequence {
                  tunnel: [w683] -> _
                  tunnel: [w682] -> _
                  tunnel: w664 -> [w681]
                  tunnel: [w671] -> _
                  tunnel: [w674] -> _
                  tunnel: w663 -> [w672]
                  tunnel: w662 -> [w671]
                  frame #0 {
                    n287 = call "get sample sheet data cells.vi"("error in (no error)"=w681, "NI_report in"=w671) -> ("error out"=w684:errorcluster, "data"=w679:string[][], "NI_report out"=w683:refnum<class "NI_report.lvclass">, "left edge output cluster"=w677:cluster{"row":i32, "column":i32})  [unwired: 5 in, 1 out]
                    n288 = Array Subset(array=w679, index (col)=2 ("index")) -> ()  [unwired: 3 in, 1 out]
                    n289 = call "find last occupied cell.vi"("Active Sheet"=w672, "Header Rows to remove"=3, "sub array start"=w677, "error in (no error)"=w684) -> ("row max value"=w676:i32, 13:"start of last occupied row"=w682:cluster{"row":i32, "column":i32}, 14:"start of last occupied row"=w675:string, "error out"=w674:errorcluster)  [unwired: 5 in, 3 out]
                    n290 = local write "row max value"(w676) -> ()
                    n291 = local write "last occupied cell's name"(w675) -> ()
                    n292 = local write "Sonde Data Array"(T12[] [{"Head"=0.0, "Depth"=0.0, "Time"="19:00", "Cumulative\nVolume"=0.0, "Sp. Conductance"={"Value"=0.506, "%"=0.0, "Tol."=TRUE}, "Dissolved Oxygen"={"Value"=35.14, "%"=0.0, "Tol."=TRUE}, "pH"={"Value"=4.81, "%"=0.0, "Tol."=TRUE}, "ORP"={"Value"=390.0, "%"=0.0, "Tol."=TRUE}, "Temperature"={"Value"=23.86, "%"=0.0, "Tol."=TRUE}, "Salinity"={"Value"=0.24, "%"=0.0, "Tol."=TRUE}, "Final Tol."=TRUE, "Final"=FALSE}, {"Head"=0.0, "Depth"=0.0, "Time"="19:00", "Cumulative\nVolume"=0.0, "Sp. Conductance"={"Value"=0.506, "%"=0.0, "Tol."=TRUE}, "Dissolved Oxygen"={"Value"=35.12, "%"=0.0, "Tol."=TRUE}, "pH"={"Value"=4.81, "%"=0.0, "Tol."=TRUE}, "ORP"={"Value"=390.0, "%"=0.0, "Tol."=TRUE}, "Temperature"={"Value"=23.89, "%"=0.0, "Tol."=TRUE}, "Salinity"={"Value"=0.24, "%"=0.0, "Tol."=TRUE}, "Final Tol."=TRUE, "Final"=FALSE}, {"Head"=0.0, "Depth"=0.0, "Time"="19:00", "Cumulative\nVolume"=0.0, "Sp. Conductance"={"Value"=0.506, "%"=0.0, "Tol."=TRUE}, "Dissolved Oxygen"={"Value"=35.14, "%"=0.0, "Tol."=TRUE}, "pH"={"Value"=4.81, "%"=0.0, "Tol."=TRUE}, "ORP"={"Value"=390.0, "%"=0.0, "Tol."=TRUE}, "Temperature"={"Value"=23.86, "%"=0.0, "Tol."=TRUE}, "Salinity"={"Value"=0.24, "%"=0.0, "Tol."=TRUE}, "Final Tol."=TRUE, "Final"=FALSE}, {"Head"=0.0, "Depth"=0.0, "Time"="", "Cumulative\nVolume"=0.0, "Sp. Conductance"={"Value"=0.0, "%"=0.0, "Tol."=FALSE}, "Dissolved Oxygen"={"Value"=0.0, "%"=0.0, "Tol."=FALSE}, "pH"={"Value"=0.0, "%"=0.0, "Tol."=FALSE}, "ORP"={"Value"=0.0, "%"=0.0, "Tol."=FALSE}, "Temperature"={"Value"=0.0, "%"=0.0, "Tol."=FALSE}, "Salinity"={"Value"=0.0, "%"=0.0, "Tol."=FALSE}, "Final Tol."=FALSE, "Final"=FALSE}, {"Head"=0.0, "Depth"=0.0, "Time"="", "Cumulative\nVolume"=0.0, "Sp. Conductance"={"Value"=0.0, "%"=0.0, "Tol."=FALSE}, "Dissolved Oxygen"={"Value"=0.0, "%"=0.0, "Tol."=FALSE}, "pH"={"Value"=0.0, "%"=0.0, "Tol."=FALSE}, "ORP"={"Value"=0.0, "%"=0.0, "Tol."=FALSE}, "Temperature"={"Value"=0.0, "%"=0.0, "Tol."=FALSE}, "Salinity"={"Value"=0.0, "%"=0.0, "Tol."=FALSE}, "Final Tol."=FALSE, "Final"=FALSE}, {"Head"=0.0, "Depth"=0.0, "Time"="", "Cumulative\nVolume"=0.0, "Sp. Conductance"={"Value"=0.0, "%"=0.0, "Tol."=FALSE}, "Dissolved Oxygen"={"Value"=0.0, "%"=0.0, "Tol."=FALSE}, "pH"={"Value"=0.0, "%"=0.0, "Tol."=FALSE}, "ORP"={"Value"=0.0, "%"=0.0, "Tol."=FALSE}, "Temperature"={"Value"=0.0, "%"=0.0, "Tol."=FALSE}, "Salinity"={"Value"=0.0, "%"=0.0, "Tol."=FALSE}, "Final Tol."=FALSE, "Final"=FALSE}, {"Head"=0.0, "Depth"=0.0, "Time"="", "Cumulative\nVolume"=0.0, "Sp. Conductance"={"Value"=0.0, "%"=0.0, "Tol."=FALSE}, "Dissolved Oxygen"={"Value"=0.0, "%"=0.0, "Tol."=FALSE}, "pH"={"Value"=0.0, "%"=0.0, "Tol."=FALSE}, "ORP"={"Value"=0.0, "%"=0.0, "Tol."=FALSE}, "Temperature"={"Value"=0.0, "%"=0.0, "Tol."=FALSE}, "Salinity"={"Value"=0.0, "%"=0.0, "Tol."=FALSE}, "Final Tol."=FALSE, "Final"=FALSE}, {"Head"=0.0, "Depth"=0.0, "Time"="", "Cumulative\nVolume"=0.0, "Sp. Conductance"={"Value"=0.0, "%"=0.0, "Tol."=FALSE}, "Dissolved Oxygen"={"Value"=0.0, "%"=0.0, "Tol."=FALSE}, "pH"={"Value"=0.0, "%"=0.0, "Tol."=FALSE}, "ORP"={"Value"=0.0, "%"=0.0, "Tol."=FALSE}, "Temperature"={"Value"=0.0, "%"=0.0, "Tol."=FALSE}, "Salinity"={"Value"=0.0, "%"=0.0, "Tol."=FALSE}, "Final Tol."=FALSE, "Final"=FALSE}, {"Head"=0.0, "Depth"=0.0, "Time"="", "Cumulative\nVolume"=0.0, "Sp. Conductance"={"Value"=0.0, "%"=0.0, "Tol."=FALSE}, "Dissolved Oxygen"={"Value"=0.0, "%"=0.0, "Tol."=FALSE}, "pH"={"Value"=0.0, "%"=0.0, "Tol."=FALSE}, "ORP"={"Value"=0.0, "%"=0.0, "Tol."=FALSE}, "Temperature"={"Value"=0.0, "%"=0.0, "Tol."=FALSE}, "Salinity"={"Value"=0.0, "%"=0.0, "Tol."=FALSE}, "Final Tol."=FALSE, "Final"=FALSE}] ("Sonde Data Array")) -> ()
                  }
                }
              }
              frame Enabled {
              }
            }
          }
          frame "Update Depth" {
            n293 = flat-sequence {
              tunnel: w720 -> [w738]
              tunnel: [w737] -> w719
              frame #0 {
                n294 = local read "Sensor  Real \nMeasurements"() -> (w736:T6)
                n295 = Unbundle By Name(w736) -> ("String Pot"=w735:dbl)
                n296 = Bundle By Name(cluster=w738, "Absolute Depth In"="New Depth", "Current Absolute Depth"="New Depth", "Previous Relative Depth"=w735, "Current Relative Depth"=w735) -> (w737:T17)
                n297 = local write "Current Depth"("New Depth") -> ()
              }
            }
          }
          frame "IK vs Time" {
          }
          frame "Start KPRO Measurements" {
            n298 = flat-sequence {
              tunnel: w778 -> [w805]
              tunnel: w777 -> [w804]
              tunnel: [w803] -> w776
              tunnel: [w802] -> w775
              tunnel: [w799] -> w762
              frame #0 {
                n299 = local read "Input Variables and Slopes"() -> (w797:T11)
                n300 = Unbundle By Name(w797) -> ("Depth to Water Table"=w798:dbl)
                n301 = local read "Input Depths \nand Parameters Cluster"() -> (w801:T16)
                n302 = disable-structure shown="Enabled" {
                  disable-tunnel: w798 -> [w812 w813]
                  disable-tunnel: [w811 w813] -> w796
                  disable-tunnel: w805 -> [w810 w815]
                  disable-tunnel: [w809 w815] -> w802
                  disable-tunnel: w804 -> [w808 w814]
                  disable-tunnel: [w807 w814] -> w799
                  frame Enabled {
                    n303 = call <vilib>:"Clear Errors.vi"("error in (no error)"=w810) -> ("error out"=w806:errorcluster)  [unwired: 5 in, 1 out]
                    n304 = call "New Stainless Correction Pop Up 2016.vi"("error in (no error)"=w806, "New Feet\n of Stainless\n(Count)"=w808, "Depth to \nWater Table\nInput"=w812) -> ("error in (no error) 2"=w809:errorcluster, "Feet of\nStainless to be\nUsed (Count)"=w807:i32, "Depth to \nWater Table\nOutput"=w811:dbl)  [unwired: 6 in]
                  }
                  frame Disabled {
                  }
                }
                n305 = Bundle By Name(cluster=w797, "Depth to Water Table"=w796) -> (w803:T11)
                n306 = Bundle By Name(cluster=w801, "Feet of Stainless"=w799) -> (w800:T16)
                n307 = local write "Input Depths \nand Parameters Cluster"(w800) -> ()
              }
            }
            n308 = flat-sequence {
              tunnel: w789 -> [w843]
              tunnel: [w842] -> w788
              tunnel: w776 -> [w841]
              tunnel: w775 -> [w840]
              tunnel: [w839] -> w774
              tunnel: [w829] -> w773
              frame #0 {
                n309 = control-ref of="Input Variables and Slopes"() -> (w835:refnum<vi>)
                n310 = control-ref of="Sensor Voltage Cluster"() -> (w833:refnum<vi>)
                n311 = control-ref of="Zero In-Line Pressure\n(F = leave as is)"() -> (w832:refnum<vi>)
                n312 = control-ref of="Output File Path"() -> (w836:refnum<vi>)
                n313 = control-ref of="Descriptions"() -> (w834:refnum<vi>)
                n314 = call "measure down hole pressure and save to csv file.vi"("Path in"=w836, "reference 3"=w834, "reference in"=w835, "reference 4"=w833, "reference 5"=w832, "Record DTW File"="Record DTW File", "error in (no error)"=w840, "Array in"=w843, "Input Variables and Slopes"=w841) -> ("DTW path 2"=→"Down hole Pressure Transducer CSV data  path 2":path, "Array out"=w842:refnum<k24>[], "In-Line Pressure"=w829:dbl, "error out"=w839:errorcluster)  [unwired: 3 in]
                "Down hole Pressure" <- w829
                n315 = local read "Corrected Pressure Cluster"() -> (w831:T20)
                n316 = Bundle By Name(cluster=w831, "Down hole Corrected Pressure"=w829) -> (w830:T20)
                n317 = invoke on="Update Sonde" class="Bool (strict)" method="Reinit To Default"() -> ()  [unwired: 3 in, 3 out]
                n318 = local write "Corrected Pressure Cluster"(w830) -> ()
                n319 = property on="Large Depth IK Graph" class="WFChart (strict)"("History Data"=dbl[] []) -> ()  [unwired: 2 in, 2 out]
              }
            }
            n320 = flat-sequence {
              tunnel: w788 -> [w909]
              tunnel: [w905] -> w772
              tunnel: [w904] -> w771
              frame #0 {
                n321 = local read "Input Variables and Slopes"() -> (w912:T11)
                n322 = Unbundle By Name(w912) -> ("Up Hole Pressure Slope"=w911:dbl, "Up Hole  Pressure Offset"=w908:dbl)
                n323 = local write "Input Variables and Slopes"(w912) -> ()
                n324 = local read "Sensor Voltage Cluster"() -> (w913:T9)
                n325 = local read "Descriptions"() -> (w905:string[])
                n326 = local read "Corrected Pressure Cluster"() -> (w907:T20)
                n327 = call "up hole Pressure 2016.vi"("Sensor Cluster"=w913, "Pressure Offset"=w908, "Array in"=w909, "Pressure \nSlope"=w911, "Descriptions"=w905, "Zero Pressure\n(F = leave as is)"=TRUE) -> ("Array out"=w904:refnum<k24>[], "Uphole Pressure"=w903:dbl, "Sensor Cluster 2"=w910:T9)  [unwired: 7 in]
                n328 = Bundle By Name(cluster=w907, "Up hole Corrected Pressure"=w903) -> (w906:T20)
                n329 = local write "Sensor Voltage Cluster"(w910) -> ()
                n330 = local write "Corrected Pressure Cluster"(w906) -> ()
                n331 = local write "Uphole Pressure"(w903) -> ()
              }
            }
            n332 = local read "Input Variables and Slopes"() -> (w767:T11)
            n333 = Unbundle By Name(w767) -> ("String Pot Slope"=w766:dbl)
            n334 = call "depth read from string pot 2016.vi"("Descriptions"=w772, "error in (no error)"=w769, "String Pot \nSlope"=w766, "Array in"=w771) -> ("Array out"=w770:refnum<k24>[], "Depth"=w764:dbl, "error out"=w768:errorcluster)  [unwired: 12 in, 1 out]
            n335 = flat-sequence {
              tunnel: w764 -> [w817]
              tunnel: [w816] -> w763
              frame #0 {
                w818 = 15  # Filter Size
                # "Functional Global in \nBoxcar Integrator\nInitialize filter array to \ncurrent string pot value"
                n336 = call "Boxcar filter2016.vi"("Initialize"=TRUE, "Filter Size"=w818, "Filter Input"=w817) -> ("Filter Output"=w816:dbl)
              }
            }
            n337 = flat-sequence {
              tunnel: [w820] -> w765
              frame #0 {
                n338 = Tick Count (ms)() -> (millisecond timer value=w822:u32)
                n339 = Divide(x=w822, y=u32 1000) -> (x/y=w820:dbl)
              }
            }
            n340 = flat-sequence {
              tunnel: [w826] -> w759
              tunnel: w763 -> [w827]
              tunnel: w765 -> [w825]
              tunnel: w760 -> [w824]
              frame #0 {
                n341 = local read "Current Depth"() -> (w823:sgl)
                n342 = Bundle By Name(cluster=w824, "Previous Relative Depth"=w827, "Current Relative Depth"=w827, "First Relative Depth"=w827, "Current Measurement Time"=w825, "Previous Measurement Time"=w825, "Absolute Depth In"=w823, "Current Absolute Depth"=w823, "First Absolute Depth"=w823) -> (w826:T17)
              }
            }
            n343 = flat-sequence {
              tunnel: w772 -> [w896]
              tunnel: w770 -> [w899]
              tunnel: [w894] -> w785
              tunnel: [w896] -> w787
              tunnel: [w895] -> w783
              tunnel: [w893] -> w781
              frame #0 {
                w900 = 0.0  # Offset
                n344 = local read "Input Variables and Slopes"() -> (w898:T11)
                n345 = Unbundle By Name(w898) -> ("Flow Slope"=w897:dbl)
                n346 = local read "Input Depths \nand Parameters Cluster"() -> (w902:T16)
                n347 = call "Flow 2016.vi"("Descriptions"=w896, "Array in"=w899, "Flow Slope"=w897, "Offset"=w900) -> ("Sensor Cluster"=w894:T9, "Flow (ml/min)"=w895:dbl, "Array out"=w893:refnum<k24>[])  [unwired: 4 in]
                n348 = local write "Sensor Voltage Cluster"(w894) -> ()
                n349 = Bundle By Name(cluster=w902, "Flow"=w895) -> (w901:T16)
                n350 = local write "Input Depths \nand Parameters Cluster"(w901) -> ()
              }
            }
            n351 = flat-sequence {
              tunnel: w787 -> [w880]
              tunnel: w786 -> [w853]
              tunnel: w785 -> [w879]
              tunnel: w759 -> [w878]
              tunnel: [w877] -> w784
              tunnel: w783 -> [w876]
              tunnel: w781 -> [w868]
              tunnel: [w867] -> _
              tunnel: [w844] -> w780
              tunnel: w773 -> [w859]
              tunnel: w758 -> [w848]
              tunnel: [w845] -> w757
              frame #0 {
                n352 = local read "Culmulative Graph Cluster"() -> (w866:T19)
                n353 = local read "Input Depths \nand Parameters Cluster"() -> (w872:T16)
                n354 = local read "Input Variables and Slopes"() -> (w875:T11)
                n355 = local read "KPRO Finish\nIndicator"() -> (w860:bool)
                n356 = local read "Depth mode"() -> (w854:bool)
                n357 = Unbundle By Name(w872) -> ("Feet of Stainless"=w861:i32, "Zeroed \nPressure"=w873:dbl)
                n358 = Unbundle By Name(w875) -> ("String Pot Slope"=w874:dbl)
                n359 = call "Kpro Read String Pot 2016.vi"("Read String Pot"=w854, "Feet of\nStainless to be\nUsed (Count) in"=w861, "Session Array in"=dbl[][] [], "Flow"=w876, "Finished In"=w860, "Depth Cluster in"=w878, "String Pot \nSlope in"=w874, "Sensor Cluster In in"=w879, "Descriptions"=w880, "Pressure in"=w873, "Array in"=w868, "Downhole Pressure Sensor"=w859) -> ("Sensor Cluster 2"=w869:T9, "Array out"=w867:refnum<k24>[], "Generate Array Calc IK"=w846:bool, "Feet of\nStainless to be\nUsed (Count) out"=w870:i32, "Depth Cluster out"=w877:T17, "Single String Pot Session Array out"=w845:dbl[][])  [unwired: 7 in, 3 out]
                n360 = local write "Current Session"(w845) -> ()
                n361 = Build Array (concatenate)(w853, w848) -> (w849:dbl[][])
                n362 = local write "Sensor Voltage Cluster"(w869) -> ()
                n363 = Unbundle By Name(w877) -> ("Current Absolute Depth"=w852:dbl)
                n364 = Bundle By Name(cluster=w872, "Feet of Stainless"=w870) -> (w871:T16)
                n365 = local write "Input Depths \nand Parameters Cluster"(w871) -> ()
                n366 = flat-sequence {
                  tunnel: w852 -> [w886]
                  frame #0 {
                    n367 = global write "Kpro Globals.vi" "Current Depth"(w886) -> ()
                    n368 = local write "Current Depth"(w886) -> ()
                    n369 = Divide(x=w886, y=3.281) -> (x/y=w887:dbl)
                    n370 = local read "Sample Sheet Data Row Cluster 2"() -> (w891:T2)
                    n371 = local read "Corrected Pressure Cluster"() -> (w889:T20)
                    n372 = Unbundle By Name(w889) -> ("Up hole Corrected Pressure"=w888:dbl)
                    n373 = Bundle By Name(cluster=w891, "Depth"=w886, "Head\nPressure"=w888) -> (w890:T2)
                    n374 = local write "Sample Sheet Data Row Cluster 2"(w890) -> ()
                    n375 = local write "Current \nDepth (m)"(w887) -> ()
                  }
                }
                n376 = case shown="True" FALSE {
                  tunnel: w845 -> [_ w885]
                  tunnel: [w882 w884] -> w844
                  tunnel: w849 -> [w882 w883]
                  frame False {
                  }
                  frame True {
                    n377 = Build Array (concatenate)(w883, w885) -> (w884:dbl[][])
                  }
                }
                n378 = call "Array to Plot 2016.vi"("Input Cumulative Array"=w844, "Input Real Time Array"=w845) -> ("Cumulative - Depth vs.Drive Rate"=w862:cluster{dbl[], dbl[]}, "Cumulative - Depth vs. Ik"=w864:cluster{dbl[], dbl[]}, "Real Time - Depth vs. Drive Rate"=w863:cluster{dbl[], dbl[]}, "Real Time - Depth vs. Ik"=w855:cluster{dbl[], dbl[]}, "Depth Rate"=w851:dbl)  [unwired: 2 in, 1 out]
                n379 = Bundle By Name(cluster=w866, "Cumulative - Depth vs. Ik"=w864, "Real Time - Depth vs. lk"=w855, "Cumulative - Depth vs. Drive Rate"=w863, "Real Time - Depth vs. Drive Rate"=w862) -> (w865:T19)
                n380 = local write "Culmulative Graph Cluster"(w865) -> ()
                n381 = local write "Large Depth IK Graph Cluster"(w855) -> ()
                n382 = local write "Depth Rate\nft/min"(w851) -> ()
                n383 = local write "Cumulative_data_from_file"(w844) -> ()
                n384 = control-ref of="KPRO Output File Path"() -> (w858:refnum<vi>)
                n385 = call "write KPRO file.vi"("Corrected Array in"=w844, "Generate Array Calc IK"=w846, "Path in"=w858) -> ("paths ok"=w856:bool, "appended path"=w857:path)  [unwired: 7 in]
                n386 = case shown="True" w856 {
                  tunnel: w857 -> [_ w881]
                  frame False {
                  }
                  frame True {
                    "appended path" <- w881
                  }
                }
              }
            }
          }
          frame "Increment Depth Manually" {
            n387 = disable-structure shown="Enabled" {
              disable-tunnel: w926 -> [w951 w969]
              disable-tunnel: w925 -> [w950 _]
              disable-tunnel: [w949 _] -> w924
              disable-tunnel: [w948 w970] -> w923
              disable-tunnel: [w947 w969] -> w922
              frame Disabled {
                n388 = flat-sequence {
                  tunnel: w951 -> [w959]
                  tunnel: [w958] -> w947
                  tunnel: w950 -> [w957]
                  tunnel: [w956] -> w949
                  tunnel: [w952] -> w948
                  frame #0 {
                    n389 = local read "Input Variables and Slopes"() -> (w954:T11)
                    n390 = Unbundle By Name(w954) -> ("Depth to Water Table"=w955:dbl)
                    n391 = disable-structure shown="Enabled" {
                      disable-tunnel: w955 -> [w965 w966]
                      disable-tunnel: [w964 w966] -> w953
                      disable-tunnel: w959 -> [w963 w968]
                      disable-tunnel: [w962 w968] -> w958
                      disable-tunnel: w957 -> [w961 w967]
                      disable-tunnel: [w960 w967] -> w956
                      frame Enabled {
                        n392 = call "New Stainless Correction Pop Up 2016.vi"("error in (no error)"=w963, "New Feet\n of Stainless\n(Count)"=w961, "Depth to \nWater Table\nInput"=w965) -> ("error in (no error) 2"=w962:errorcluster, "Feet of\nStainless to be\nUsed (Count)"=w960:i32, "Depth to \nWater Table\nOutput"=w964:dbl)  [unwired: 6 in]
                      }
                      frame Disabled {
                      }
                    }
                    n393 = Bundle By Name(cluster=w954, "Depth to Water Table"=w953) -> (w952:T11)
                  }
                }
              }
              frame Enabled {
                n394 = local read "Input Variables and Slopes"() -> (w970:T11)
              }
            }
            n395 = flat-sequence {
              tunnel: w940 -> [w1065]
              tunnel: [w1064] -> w939
              tunnel: w923 -> [w1063]
              tunnel: w922 -> [w1062]
              tunnel: [w1061] -> w921
              tunnel: [w1057] -> w919
              frame #0 {
                n396 = flat-sequence {
                  tunnel: [w1082] -> w1070
                  tunnel: [w1071] -> w1069
                  tunnel: [w1081] -> w1068
                  tunnel: [w1080] -> w1067
                  tunnel: [w1079] -> w1066
                  tunnel: w1065 -> [w1078]
                  tunnel: [w1077] -> w1064
                  tunnel: w1063 -> [w1073]
                  tunnel: [w1071] -> w1057
                  frame #0 {
                    n397 = local read "Zero In-Line Pressure\n(F = leave as is)"() -> (w1072:bool)
                    n398 = Unbundle By Name(w1073) -> ("DH Pressure Trans Slope"=w1080:dbl, "DH Pressure Offset"=w1079:dbl)
                    n399 = local read "Sensor Voltage Cluster"() -> (w1075:T9)
                    n400 = local write "Input Variables and Slopes"(w1073) -> ()
                    n401 = local read "Descriptions"() -> (w1076:string[])
                    n402 = global read "Kpro Globals.vi" "Current Depth"() -> (w1082:sgl)
                    n403 = call "DHT Pressure 2016.vi"("Sensor Cluster"=w1075, "DHT Pressure Offset"=w1079, "Array in"=w1078, "DHT Pressure \nSlope"=w1080, "Descriptions"=w1076, "Zero Pressure\n(F = leave as is)"=w1072) -> ("Array out"=w1077:refnum<k24>[], "DHT Pressure"=w1081:dbl, "Sensor Cluster 2"=w1074:T9)  [unwired: 7 in]
                    n404 = local write "Sensor Voltage Cluster"(w1074) -> ()
                    n405 = Add(x=w1081, y=w1082) -> (x+y=w1071:dbl)
                    n406 = local write "Down hole Pressure"(w1071) -> ()
                  }
                }
                n407 = local read "Record DTW File"() -> (w1060:bool)
                n408 = case shown="True" w1060 {
                  selector: w1060 -> [w1084 _]
                  tunnel: [w1084 FALSE ("Boolean")] -> _
                  tunnel: w1069 -> [_ w1096]
                  tunnel: w1070 -> [_ w1097]
                  tunnel: w1066 -> [_ w1094]
                  tunnel: w1068 -> [_ w1095]
                  tunnel: w1067 -> [_ w1093]
                  tunnel: w1062 -> [w1083 w1088]
                  tunnel: [w1083 w1087] -> w1061
                  frame False {
                  }
                  frame True {
                    n409 = Build Array(w1097, w1096, w1095, w1094, w1093) -> (w1100:dbl[])
                    n410 = local read "Output File Path"() -> (w1092:path)
                    n411 = call-poly "Strip Path__ogtk.vi"("path"=w1092) -> ("stripped path"=w1091:path)  [unwired: 1 out]
                    n412 = call-poly "Strip Path__ogtk.vi"("path"=path "DTW.csv") -> ("name"=w1089:string)  [unwired: 1 out]
                    n413 = call-poly "Build Path__ogtk.vi"("name or relative path"=w1089, "base path"=w1091) -> ("appended path"=w1085:path)
                    n414 = local write "Down hole Pressure Transducer CSV data  path 2"(w1085) -> ()
                    n415 = call-poly <vilib>:"Write Delimited Spreadsheet.vi"("file path (dialog if empty)"=w1085, "1D data"=w1100, "append to file? (new file:F)"=TRUE, "error in (no error)"=w1088, "delimiter (\\t)"="," ("delimiter (\\t)")) -> ("error out"=w1087:errorcluster)  [unwired: 9 in, 1 out]
                  }
                }
                n416 = local read "Corrected Pressure Cluster"() -> (w1058:T20)
                n417 = Bundle By Name(cluster=w1058, "Down hole Corrected Pressure"=w1057) -> (w1059:T20)
                n418 = local write "Corrected Pressure Cluster"(w1059) -> ()
              }
            }
            n419 = flat-sequence {
              tunnel: w939 -> [w1051]
              tunnel: [w1047] -> w938
              tunnel: [w1046] -> w937
              frame #0 {
                n420 = local read "Input Variables and Slopes"() -> (w1054:T11)
                n421 = Unbundle By Name(w1054) -> ("Up Hole Pressure Slope"=w1053:dbl, "Up Hole  Pressure Offset"=w1050:dbl)
                n422 = local write "Input Variables and Slopes"(w1054) -> ()
                n423 = local read "Sensor Voltage Cluster"() -> (w1055:T9)
                n424 = local read "Descriptions"() -> (w1047:string[])
                n425 = local read "Corrected Pressure Cluster"() -> (w1049:T20)
                n426 = call "up hole Pressure 2016.vi"("Sensor Cluster"=w1055, "Pressure Offset"=w1050, "Array in"=w1051, "Pressure \nSlope"=w1053, "Descriptions"=w1047, "Zero Pressure\n(F = leave as is)"=TRUE) -> ("Array out"=w1046:refnum<k24>[], "Uphole Pressure"=w1045:dbl, "Sensor Cluster 2"=w1052:T9)  [unwired: 7 in]
                n427 = Bundle By Name(cluster=w1049, "Up hole Corrected Pressure"=w1045) -> (w1048:T20)
                n428 = local write "Sensor Voltage Cluster"(w1052) -> ()
                n429 = local write "Corrected Pressure Cluster"(w1048) -> ()
                n430 = local write "Uphole Pressure"(w1045) -> ()
              }
            }
            n431 = flat-sequence {
              tunnel: w938 -> [w1038]
              tunnel: w937 -> [w1041]
              tunnel: [w1036] -> w934
              tunnel: [w1038] -> w936
              tunnel: [w1037] -> w931
              tunnel: [w1035] -> w929
              frame #0 {
                w1042 = 0.0  # Offset
                n432 = local read "Input Variables and Slopes"() -> (w1040:T11)
                n433 = Unbundle By Name(w1040) -> ("Flow Slope"=w1039:dbl)
                n434 = local read "Input Depths \nand Parameters Cluster"() -> (w1044:T16)
                n435 = call "Flow 2016.vi"("Descriptions"=w1038, "Array in"=w1041, "Flow Slope"=w1039, "Offset"=w1042) -> ("Sensor Cluster"=w1036:T9, "Flow (ml/min)"=w1037:dbl, "Array out"=w1035:refnum<k24>[])  [unwired: 4 in]
                n436 = local write "Sensor Voltage Cluster"(w1036) -> ()
                n437 = Bundle By Name(cluster=w1044, "Flow"=w1037) -> (w1043:T16)
                n438 = local write "Input Depths \nand Parameters Cluster"(w1043) -> ()
              }
            }
            n439 = flat-sequence {
              tunnel: w936 -> [w1018]
              tunnel: w935 -> [w982]
              tunnel: w934 -> [w1017]
              tunnel: w933 -> [w995]
              tunnel: [w1016] -> w932
              tunnel: w931 -> [w1015]
              tunnel: w929 -> [w1006]
              tunnel: [w1005] -> _
              tunnel: [w972] -> w928
              tunnel: w920 -> [w999]
              tunnel: w919 -> [w991]
              tunnel: [w971] -> w917
              tunnel: w916 -> [w980]
              frame #0 {
                n440 = Unbundle By Name(w995) -> ("Current Relative Depth"=w992:dbl)
                n441 = local read "Input Depths \nand Parameters Cluster"() -> (w994:T16)
                n442 = Unbundle By Name(w994) -> ("Start Depth"=w993:sgl)
                n443 = global read "Kpro Globals.vi" "increment_amount"() -> (w997:dbl)
                n444 = local read "Culmulative Graph Cluster"() -> (w1004:T19)
                n445 = local read "Input Depths \nand Parameters Cluster"() -> (w1010:T16)
                n446 = Equal?(x=w992, y=w993) -> (x = y?=w988:bool)
                n447 = And(x=w988, y=TRUE) -> (x .and. y?=w989:bool)
                n448 = First Call?() -> ()  [unwired: 1 out]
                n449 = local read "Input Variables and Slopes"() -> (w1014:T11)
                n450 = local read "KPRO Finish\nIndicator"() -> (w996:bool)
                n451 = local read "Depth mode"() -> (w979:bool)
                n452 = case shown="False" w989 {
                  tunnel: w992 -> [w1022 w1023]
                  tunnel: [w1021 w1023] -> w998
                  tunnel: w997 -> [w1020 _]
                  frame False {
                    n453 = Add(x=w1020, y=w1022) -> (x+y=w1021:dbl)
                  }
                  frame True {
                  }
                }
                n454 = Unbundle By Name(w1010) -> ("Feet of Stainless"=w1012:i32, "Zeroed \nPressure"=w1011:dbl)
                n455 = Unbundle By Name(w1014) -> ("String Pot Slope"=w1013:dbl)
                n456 = call "Kpro Read String Pot 2016.vi"("Read String Pot"=w979, "Feet of\nStainless to be\nUsed (Count) in"=w1012, "Session Array in"=w980, "Flow"=w1015, "Manual Depth In"=w998, "Finished In"=w996, "Depth Cluster in"=w995, "error in (no error)"=w999, "String Pot \nSlope in"=w1013, "Sensor Cluster In in"=w1017, "Descriptions"=w1018, "Pressure in"=w1011, "Array in"=w1006, "Downhole Pressure Sensor"=w991) -> ("Sensor Cluster 2"=w1007:T9, "IK"=w981:dbl, "Array out"=w1005:refnum<k24>[], "Generate Array Calc IK"=w978:bool, "Depth Rate"=→"Depth Rate\nft/min":dbl, "Feet of\nStainless to be\nUsed (Count) out"=w1008:i32, "Depth Cluster out"=w1016:T17, "Single String Pot Session Array out"=w971:dbl[][])  [unwired: 5 in, 1 out]
                "Ik" <- w981
                n457 = And(x=w979, y=w978) -> ()  [unwired: 1 out]
                n458 = local write "Sensor Voltage Cluster"(w1007) -> ()
                n459 = Unbundle By Name(w1016) -> ("Current Absolute Depth"=w984:dbl)
                n460 = Bundle By Name(cluster=w1010, "Feet of Stainless"=w1008) -> (w1009:T16)
                n461 = local write "Ik"(w981) -> ()
                n462 = local write "Input Depths \nand Parameters Cluster"(w1009) -> ()
                n463 = flat-sequence {
                  tunnel: w984 -> [w1028]
                  frame #0 {
                    n464 = local read "Corrected Pressure Cluster"() -> (w1031:T20)
                    n465 = global write "Kpro Globals.vi" "Current Depth"(w1028) -> ()
                    n466 = local write "Current Depth"(w1028) -> ()
                    n467 = Divide(x=w1028, y=3.281) -> (x/y=w1029:dbl)
                    n468 = local read "Sample Sheet Data Row Cluster 2"() -> (w1033:T2)
                    n469 = local write "Current \nDepth (m)"(w1029) -> ()
                    n470 = Unbundle By Name(w1031) -> ("Up hole Corrected Pressure"=w1030:dbl)
                    n471 = Bundle By Name(cluster=w1033, "Depth"=w1028, "Head\nPressure"=w1030) -> (w1032:T2)
                    n472 = local write "Sample Sheet Data Row Cluster 2"(w1032) -> ()
                  }
                }
                n473 = case shown="True" FALSE {
                  tunnel: w971 -> [_ w1025]
                  tunnel: [w1024 w1026] -> w972
                  tunnel: w982 -> [w1024 w1027]
                  frame False {
                  }
                  frame True {
                    n474 = Build Array (concatenate)(w1027, w1025) -> (w1026:dbl[][])
                  }
                }
                n475 = call "Array to Plot 2016.vi"("Input Cumulative Array"=w972, "Input Real Time Array"=w971) -> ("Cumulative - Depth vs.Drive Rate"=w1000:cluster{dbl[], dbl[]}, "Cumulative - Depth vs. Ik"=w1002:cluster{dbl[], dbl[]}, "Real Time - Depth vs. Drive Rate"=w1001:cluster{dbl[], dbl[]}, "Real Time - Depth vs. Ik"=w986:cluster{dbl[], dbl[]}, "Depth Rate"=w983:dbl)  [unwired: 2 in, 1 out]
                n476 = Bundle By Name(cluster=w1004, "Cumulative - Depth vs. Ik"=w1002, "Real Time - Depth vs. lk"=w986, "Cumulative - Depth vs. Drive Rate"=w1001, "Real Time - Depth vs. Drive Rate"=w1000) -> (w1003:T19)
                n477 = local write "Culmulative Graph Cluster"(w1003) -> ()
                n478 = local write "Large Depth IK Graph Cluster"(w986) -> ()
                n479 = local write "Depth Rate\nft/min"(w983) -> ()
                n480 = control-ref of="KPRO Output File Path"() -> (w974:refnum<vi>)
                n481 = call "write KPRO file.vi"("String"="_KPRO_session.csv", "Corrected Array in"=w971, "Generate Array Calc IK"=w978, "Path in"=w974) -> ("paths ok"=w987:bool, "appended path"=w990:path)  [unwired: 6 in]
                n482 = case shown="True" w987 {
                  tunnel: w990 -> [_ w1019]
                  frame False {
                  }
                  frame True {
                    n483 = local write "KPRO Output File Path"(w1019) -> ()
                  }
                }
                n484 = call "write KPRO file.vi"("String"="_KPRO.csv", "Corrected Array in"=w972, "Path in"=w974) -> ()  [unwired: 7 in, 2 out]
                n485 = local write "Current Session"(w971) -> ()
                n486 = local write "Cumulative_data_from_file"(w972) -> ()
              }
            }
          }
          frame "Sample Not Collected" {
            n487 = local write "Tab Control"(T3."Recording Reason Sonde" ("Tab Control")) -> ()
          }
          frame "Record Reason" {
            n488 = flat-sequence {
              frame #0 {
                n489 = local read "Sample Sheet Data Row Cluster 2"() -> (w1157:T2)
                n490 = local write "Tab Control"(T3."Recording Reason Sonde" ("Tab Control")) -> ()
                n491 = local read "KPRO Output File Path"() -> (w1153:path)
                n492 = property on="Select Reasons to Record Data" class="Ring (strict)"() -> ("Strings []"=w1144:string[])  [unwired: 2 in, 2 out]
                n493 = Get Date/Time In Seconds() -> (seconds since 1Jan1904=w1156:timestamp)
                n494 = Unbundle By Name(w1157) -> ("Head\nPressure"=w1155:dbl, "Depth"=w1154:dbl)
                n495 = call-poly "Strip Path Extension__ogtk.vi"("path"=w1153) -> ("root"=w1152:string)  [unwired: 1 out]
                n496 = local read "Recording Reason Sonde array"() -> (w1138:string[][])
                n497 = call-poly "Convert File Extension__ogtk.vi"("new ending (none)"="_Sample failure.csv", "file name"=w1152) -> ("new filename"=w1150:string)  [unwired: 1 out]
                n498 = Index Array(array=w1144, index="Select Reasons to Record Data") -> (element=w1142:string)
                n499 = Format Date/Time String(seconds (now)=w1156) -> (date/time string=w1148:string)  [unwired: 2 in]
                n500 = Format Into String(w1155) -> (resulting string=w1147:string)  [unwired: 3 in, 1 out]
                n501 = Format Into String(w1154) -> (resulting string=w1146:string)  [unwired: 3 in, 1 out]
                n502 = Format Into String("Select Reasons to Record Data") -> (resulting string=w1145:string)  [unwired: 3 in, 1 out]
                n503 = Build Array(w1148, w1147, w1146, w1145, w1142) -> (w1136:string[])
                n504 = String To Path(string=w1150) -> (path=w1151:path)
                "Sonde Recording Failure Path" <- w1151
                n505 = Build Array (concatenate)(w1138, w1136) -> (→"Recording Reason Sonde array":string[][])
                n506 = call-poly <vilib>:"Write Delimited Spreadsheet.vi"("file path (dialog if empty)"=w1151, "1D data"=w1136, "append to file? (new file:F)"=TRUE, "delimiter (\\t)"="," ("delimiter (\\t)")) -> ()  [unwired: 10 in, 2 out]
              }
            }
          }
          frame "Record IK Reason" {
            n507 = flat-sequence {
              frame #0 {
                n508 = local read "Select Entry for IK Log File"() -> (w1180:u16)
                n509 = property on="Select Entry for IK Log File" class="Ring (strict)"() -> ("Strings []"=w1179:string[])  [unwired: 2 in, 2 out]
                n510 = local read "Sample Sheet Data Row Cluster 2"() -> (w1196:T2)
                n511 = local write "Tab Control"(T3."Pressure/Flow/IK Graphs" ("Tab Control")) -> ()
                n512 = local read "KPRO Output File Path"() -> (w1192:path)
                n513 = Get Date/Time In Seconds() -> (seconds since 1Jan1904=w1195:timestamp)
                n514 = Unbundle By Name(w1196) -> ("Head\nPressure"=w1194:dbl, "Depth"=w1193:dbl)
                n515 = call-poly "Strip Path Extension__ogtk.vi"("path"=w1192) -> ("root"=w1191:string)  [unwired: 1 out]
                n516 = call-poly "Convert File Extension__ogtk.vi"("new ending (none)"="_IK Behavior.csv", "file name"=w1191) -> ("new filename"=w1189:string)  [unwired: 1 out]
                n517 = Index Array(array=w1179, index=w1180) -> (element=w1183:string)
                n518 = Format Date/Time String(seconds (now)=w1195) -> (date/time string=w1187:string)  [unwired: 2 in]
                n519 = local read "IK Reason array"() -> (w1175:string[][])
                n520 = Format Into String(w1194) -> (resulting string=w1186:string)  [unwired: 3 in, 1 out]
                n521 = Format Into String(w1193) -> (resulting string=w1185:string)  [unwired: 3 in, 1 out]
                n522 = Format Into String(w1180) -> (resulting string=w1184:string)  [unwired: 3 in, 1 out]
                n523 = Build Array(w1187, w1186, w1185, w1184, w1183) -> (w1182:string[])
                n524 = String To Path(string=w1189) -> (path=w1190:path)
                "Sonde IK Behavior Path" <- w1190
                n525 = Build Array (concatenate)(w1175, w1182) -> (→"IK Reason array":string[][])
                n526 = call-poly <vilib>:"Write Delimited Spreadsheet.vi"("file path (dialog if empty)"=w1190, "1D data"=w1182, "append to file? (new file:F)"=TRUE, "delimiter (\\t)"="," ("delimiter (\\t)")) -> ()  [unwired: 10 in, 2 out]
              }
            }
          }
          frame "Continuous  Sonde Data" {
            n527 = local read "Found Quanta Sonde Com Port"() -> (w1220:refnum<visa-resource-name>)
            n528 = control-ref of="Sonde Data Display"() -> (w1223:refnum<vi>)
            n529 = local read "Sample Sheet Data Row Cluster 2"() -> (w1200:T2)
            n530 = Unbundle By Name(w1200) -> ("Sonde Data Cluster.Cumulative\nVolume"=w1199:dbl)
            n531 = call "SDI-12 Continuous Operations.vi"("RS232 Port In"=w1220, "Sensor Address In"="0", "Sonde Data Ctl Refnum"=w1223, "Error In (No Error)"=w1222) -> ("output cluster"=w1198:T1, "Temperature"=w1218:cluster{"Y":dbl[], "Y":dbl[]}[], "Sonde Data Display"=w1217:T14, "Error Out"=w1221:errorcluster)  [unwired: 8 in, 4 out]
            n532 = Bundle By Name(cluster=w1198, "Cumulative\nVolume"=w1199) -> (w1197:T1)
            n533 = Bundle By Name(cluster=w1200, "Sonde Data Cluster"=w1197) -> (w1219:T2)
            n534 = local write "Temperature"(w1218) -> ()
            n535 = local write "Sonde Data Display"(w1217) -> ()
            n536 = local write "Sample Sheet Data Row Cluster 2"(w1219) -> ()
          }
          frame "Acq. Single Sonde Point" {
            n537 = invoke on="Record Single Sample" class="Bool" method="Reinit To Default"(error in=w1257) -> (error out=w1256:errorcluster)  [unwired: 2 in, 2 out]
            n538 = flat-sequence {
              tunnel: w1266 -> [w1313]
              tunnel: [w1306] -> _
              tunnel: w1267 -> [w1311]
              tunnel: [w1310] -> w1265
              tunnel: [w1309] -> _
              tunnel: [w1308] -> w1260
              tunnel: w1268 -> [w1306]
              frame #0 {
                n539 = Array Subset(array=w1306, index (col)=2 ("index")) -> (w1302:string[][])  [unwired: 3 in]
                n540 = local write "subarray"(w1302) -> ()
                n541 = local read "Current Sample Sheet"() -> (w1305:string)
                n542 = call "find last occupied cell.vi"("data"=w1306, "Active Sheet"=w1305, "Header Rows to remove"=3, "sub array start"=w1311, "error in (no error)"=w1313) -> ("row max value"=w1309:i32, "column max value"=w1304:i32, 13:"start of last occupied row"=w1308:cluster{"row":i32, "column":i32}, 14:"start of last occupied row"=w1303:string, "error out"=w1310:errorcluster)  [unwired: 4 in, 2 out]
                n543 = local write "last occupied cell's name"(w1303) -> ()
                n544 = local write "row max value"(w1304) -> ()
              }
            }
            n545 = call <vilib>:"Clear Errors.vi"("error in (no error)"=w1256) -> ("error out"=w1246:errorcluster)  [unwired: 5 in, 1 out]
            n546 = call "get sample sheet data cells.vi"("error in (no error)"=w1246, "NI_report in"=w1269) -> ("error out"=w1266:errorcluster, "data"=w1268:string[][], "NI_report out"=w1261:refnum<class "NI_report.lvclass">, "left edge output cluster"=w1267:cluster{"row":i32, "column":i32})  [unwired: 5 in, 1 out]
            n547 = flat-sequence {
              tunnel: w1265 -> [w1286]
              tunnel: [w1285] -> w1262
              tunnel: w1252 -> [w1284]
              tunnel: [w1283] -> w1251
              tunnel: [w1282] -> w1250
              tunnel: w1249 -> [w1281]
              tunnel: [w1272] -> w1242
              tunnel: [w1280] -> w1232
              tunnel: w1229 -> [w1279]
              frame #0 {
                n548 = control-ref of="Found Quanta Sonde Com Port"() -> (w1278:refnum<vi>)
                n549 = control-ref of="Current Time (s)"() -> (w1274:refnum<vi>)
                n550 = control-ref of="Sonde Data Display"() -> (w1277:refnum<vi>)
                n551 = control-ref of="Sonde Data Display"() -> (w1276:refnum<vi>)
                n552 = local write "Tab Control"(T3."Sonde Data" ("Tab Control")) -> ()
                n553 = control-ref of="Temperature"() -> (w1275:refnum<vi>)
                n554 = local read "Sample Sheet Data Row Cluster 2"() -> (w1271:T2)
                n555 = call "Sonde Single Measurement Subvi.vi"("VISAResourceName in"=w1278, "Time Array"=w1284, "Cumulative Sonde Data"=w1281, "Previous time"=w1279, "Sonde Data Display"=w1277, "Sonde Graph in"=w1276, "Temp Graph 3"=w1275, "error in (no error)"=w1286, "Row Cluster Input"=w1271, "reference 5"=w1274) -> ("seconds since 1Jan1904"=w1280:timestamp, "Cumulative Sonde \nData Out"=w1282:dbl[][], "Sample Sheet Data Row Cluster 2"=w1272:T2, "output cluster"=→"output cluster":T1, "time array out"=w1283:dbl[], "error out"=w1285:errorcluster)
                n556 = local write "Sample Sheet Data Row Cluster 2"(w1272) -> ()
              }
            }
            n557 = call "write out sonde row.vi"("NI_report in"=w1261, "Columns"=w1264, "Column of Volume"=w1263, "Sample Sheet Data Row Cluster"=w1242, "row index"=w1233, "error in (no error)"=w1262, "start of last occupied row"=w1260) -> ("NI_report out"=w1259:refnum<class "NI_report.lvclass">, "row index out"=w1253:i32, "error out"=w1241:errorcluster)  [unwired: 6 in]
            n558 = To Double Precision Float(number=w1232) -> ()  [unwired: 1 out]
            n559 = call "populate sonde row cluster from sonde data cluster.vi"("Initialize \nInitial Value \nCluster"=TRUE ("Initialize \nInitial Value \nCluster"), "error in (no error)"=w1241, "Sonde Parameters \nInitial Values"=w1237, "Sample Sheet Data Row Cluster"=w1242, "Sonde Parameters \nTolerance Limits"="Sonde Parameters \nTolerance Limits") -> ("error out"=w1240:errorcluster, "Cluster"=w1230:T12, "Sonde Parameters \nInitial Values Out"=w1227:T5)  [unwired: 4 in]
            n560 = local read "Sonde Data Array"() -> (w1235:T12[])
            n561 = local write "Sonde Parameters \nInitial Values"(w1227) -> ()
            n562 = Insert Into Array(array=w1235, index=w1233, new element=w1230) -> (w1234:T12[])
            n563 = local write "Sonde Data Array"(w1234) -> ()
            n564 = flat-sequence {
              tunnel: w1240 -> [w1301]
              tunnel: w1259 -> [w1300]
              tunnel: [w1299] -> w1258
              tunnel: [w1294] -> w1255
              tunnel: [w1292] -> w1254
              frame #0 {
                (unwired) 3 ("Header Rows to remove")
                n565 = call <vilib>:"Clear Errors.vi"("error in (no error)"=w1301) -> ("error out"=w1288:errorcluster)  [unwired: 5 in, 1 out]
                n566 = local read "Current Sample Sheet"() -> (w1290:string)
                n567 = call "get sample sheet data cells.vi"("error in (no error)"=w1288, "NI_report in"=w1300) -> ("error out"=w1295:errorcluster, "data"=w1296:string[][], "NI_report out"=w1299:refnum<class "NI_report.lvclass">, "left edge output cluster"=w1293:cluster{"row":i32, "column":i32})  [unwired: 5 in, 1 out]
                n568 = call "find last occupied cell.vi"("data"=w1296, "Active Sheet"=w1290, "Header Rows to remove"=3, "sub array start"=w1293, "error in (no error)"=w1295) -> ("row max value"=w1291:i32, 13:"start of last occupied row"=w1292:cluster{"row":i32, "column":i32}, 14:"start of last occupied row"=w1289:string, "error out"=w1294:errorcluster)  [unwired: 4 in, 3 out]
                n569 = Array Subset(array=w1296, index (col)=2 ("index")) -> (w1287:string[][])  [unwired: 3 in]
                n570 = local write "row max value"(w1291) -> ()
                n571 = local write "last occupied cell's name"(w1289) -> ()
                n572 = local write "subarray"(w1287) -> ()
              }
            }
          }
          frame "pH Calibration Zero" {
            n573 = invoke on="Record Single Sample" class="Bool" method="Reinit To Default"(error in=w1335) -> (error out=w1334:errorcluster)  [unwired: 2 in, 2 out]
            n574 = call <vilib>:"Clear Errors.vi"("error in (no error)"=w1334) -> ("error out"=w1322:errorcluster)  [unwired: 5 in, 1 out]
            n575 = call "get sample sheet data cells.vi"("error in (no error)"=w1322, "NI_report in"=w1353) -> ("error out"=w1350:errorcluster, "data"=w1352:string[][], "NI_report out"=w1345:refnum<class "NI_report.lvclass">, "left edge output cluster"=w1351:cluster{"row":i32, "column":i32})  [unwired: 5 in, 1 out]
            n576 = flat-sequence {
              tunnel: w1350 -> [w1416]
              tunnel: [w1409] -> _
              tunnel: w1351 -> [w1414]
              tunnel: [w1413] -> w1349
              tunnel: [w1412] -> _
              tunnel: [w1411] -> w1343
              tunnel: w1352 -> [w1409]
              frame #0 {
                n577 = Array Subset(array=w1409, index (col)=2 ("index")) -> ()  [unwired: 3 in, 1 out]
                n578 = local read "Current Sample Sheet"() -> (w1408:string)
                n579 = call "find last occupied cell.vi"("data"=w1409, "Active Sheet"=w1408, "Header Rows to remove"=3, "sub array start"=w1414, "error in (no error)"=w1416) -> ("row max value"=w1412:i32, "column max value"=w1407:i32, 13:"start of last occupied row"=w1411:cluster{"row":i32, "column":i32}, 14:"start of last occupied row"=w1406:string, "error out"=w1413:errorcluster)  [unwired: 4 in, 2 out]
                n580 = local write "last occupied cell's name"(w1406) -> ()
                n581 = local write "row max value"(w1407) -> ()
              }
            }
            n582 = local read "Found Quanta Sonde Com Port"() -> (w1339:refnum<visa-resource-name>)
            n583 = Equal?(x=w1339, y=refnum<visa-resource-name> refnum ("RS232 Port Out")) -> (x = y?=w1341:bool)
            n584 = case shown="True" w1341 {
              tunnel: w1339 -> [w1371 _]
              tunnel: [w1379 w1402] -> w1342
              tunnel: w1349 -> [w1373 w1405]
              tunnel: [w1382 w1405] -> w1346
              tunnel: w1329 -> [w1378 w1404]
              tunnel: [w1377 w1392] -> w1328
              tunnel: [w1376 w1391] -> w1327
              tunnel: w1326 -> [w1375 w1403]
              tunnel: w1325 -> [_ w1388]
              frame False {
                w1374 = "0" ("Sensor Address In")
                n585 = control-ref of="Sonde Data Display"() -> (w1383:refnum<vi>)
                n586 = local read "Sample Sheet Data Row Cluster 2"() -> (w1380:T2)
                n587 = call "Calibrate pH Sensor.vi"("Calibration Standard"="pH Zero", "Error In (No Error)"=w1373, "Sensor Address In"=w1374, "RS232 Port In"=w1371) -> ("Error Out"=w1372:errorcluster, "Sensor Calibrate Response"=→"pH Zero \nCalibrate Response":bool, "RS232 Port Out"=w1370:refnum<visa-resource-name>)  [unwired: 4 in, 1 out]
                n588 = call "SDI-12 Single Operation with output cluster.vi"("RS232 Port In"=w1370, "Sensor Address In"=w1374, "Sonde Data Ctl Refnum"=w1383, "Error In (No Error)"=w1372, "Time Array In"=w1378, "Measurement Array In"=w1375) -> ("time array out"=w1377:dbl[], "Measurement  array Out"=w1376:dbl[][], "output cluster"=w1381:T1, "Temperature"=w1385:cluster{"Y":dbl[], "Y":dbl[]}[], "Sonde Data Display"=w1384:T14, "Error Out"=w1382:errorcluster)  [unwired: 12 in, 4 out]
                n589 = local write "Temperature"(w1385) -> ()
                n590 = local write "Sonde Data Display"(w1384) -> ()
                n591 = Bundle By Name(cluster=w1380, "Sonde Data Cluster"=w1381) -> (w1379:T2)
              }
              frame True {
                n592 = Get Date/Time In Seconds() -> (seconds since 1Jan1904=w1394:timestamp)
                n593 = To Double Precision Float(number=w1394) -> (double precision float=w1393:dbl)
                n594 = local read "Sample Sheet Data Row Cluster 2"() -> (w1402:T2)
                n595 = Subtract(x=w1393, y=w1388) -> (x-y=w1386:dbl)
                n596 = local write "Current Time (s)"(w1386) -> ()
                n597 = Unbundle By Name(w1402) -> ("Sonde Data Cluster.Temp"=w1387:dbl, "Sonde Data Cluster.pH"=w1401:dbl, "Sonde Data Cluster.Specific\nConductance"=w1400:dbl, "Sonde Data Cluster.Salinity"=w1399:dbl, "Sonde Data Cluster.Dissolved\nOxygen"=w1398:dbl, "Sonde Data Cluster.ORP"=w1397:dbl)  [unwired: 1 out]
                n598 = Build Array(w1387, w1401, w1400, w1399, w1398, 0.0 ("element"), w1397) -> (w1395:dbl[])
                n599 = Build Array (concatenate)(w1403, w1395) -> (w1391:dbl[][])
                n600 = Build Array (concatenate)(w1404, w1386) -> (w1392:dbl[])
                n601 = call "format into Sonde Vertical Graph Data Input.vi"("Sonde Measurement Array"=w1391, "Time Array"=w1392) -> ("Sonde Data Display"=w1390:T14, "Temperature"=w1389:cluster{"X":dbl[], "Y":dbl[]}[])  [unwired: 8 in]
                n602 = local write "Temperature"(w1389) -> ()
                n603 = local write "Sonde Data Display"(w1390) -> ()
              }
            }
            n604 = local write "Sample Sheet Data Row Cluster 2"(w1342) -> ()
            n605 = call "write out sonde row.vi"("NI_report in"=w1345, "Columns"=w1348, "Column of Volume"=w1347, "Sample Sheet Data Row Cluster"=w1342, "row index"=w1331, "error in (no error)"=w1346, "start of last occupied row"=w1343) -> ("NI_report out"=w1337:refnum<class "NI_report.lvclass">, "row index out"=w1330:i32, "error out"=w1338:errorcluster)  [unwired: 6 in]
            n606 = flat-sequence {
              tunnel: w1338 -> [w1367]
              tunnel: w1337 -> [w1366]
              tunnel: [w1365] -> w1336
              tunnel: [w1360] -> w1333
              tunnel: [w1358] -> w1332
              frame #0 {
                (unwired) 3 ("Header Rows to remove")
                n607 = call <vilib>:"Clear Errors.vi"("error in (no error)"=w1367) -> ("error out"=w1354:errorcluster)  [unwired: 5 in, 1 out]
                n608 = local read "Current Sample Sheet"() -> (w1356:string)
                n609 = call "get sample sheet data cells.vi"("error in (no error)"=w1354, "NI_report in"=w1366) -> ("error out"=w1361:errorcluster, "data"=w1362:string[][], "NI_report out"=w1365:refnum<class "NI_report.lvclass">, "left edge output cluster"=w1359:cluster{"row":i32, "column":i32})  [unwired: 5 in, 1 out]
                n610 = call "find last occupied cell.vi"("data"=w1362, "Active Sheet"=w1356, "Header Rows to remove"=3, "sub array start"=w1359, "error in (no error)"=w1361) -> ("row max value"=w1357:i32, 13:"start of last occupied row"=w1358:cluster{"row":i32, "column":i32}, 14:"start of last occupied row"=w1355:string, "error out"=w1360:errorcluster)  [unwired: 4 in, 3 out]
                n611 = Array Subset(array=w1362, index (col)=2 ("index")) -> ()  [unwired: 3 in, 1 out]
                n612 = local write "row max value"(w1357) -> ()
                n613 = local write "last occupied cell's name"(w1355) -> ()
              }
            }
          }
          frame "pH Calibration Standard" {
            n614 = invoke on="Record Single Sample" class="Bool" method="Reinit To Default"(error in=w1438) -> (error out=w1437:errorcluster)  [unwired: 2 in, 2 out]
            n615 = call <vilib>:"Clear Errors.vi"("error in (no error)"=w1437) -> ("error out"=w1425:errorcluster)  [unwired: 5 in, 1 out]
            n616 = call "get sample sheet data cells.vi"("error in (no error)"=w1425, "NI_report in"=w1456) -> ("error out"=w1453:errorcluster, "data"=w1455:string[][], "NI_report out"=w1448:refnum<class "NI_report.lvclass">, "left edge output cluster"=w1454:cluster{"row":i32, "column":i32})  [unwired: 5 in, 1 out]
            n617 = flat-sequence {
              tunnel: w1453 -> [w1520]
              tunnel: [w1513] -> _
              tunnel: w1454 -> [w1518]
              tunnel: [w1517] -> w1452
              tunnel: [w1516] -> _
              tunnel: [w1515] -> w1446
              tunnel: w1455 -> [w1513]
              frame #0 {
                n618 = Array Subset(array=w1513, index (col)=2 ("index")) -> ()  [unwired: 3 in, 1 out]
                n619 = local read "Current Sample Sheet"() -> (w1512:string)
                n620 = call "find last occupied cell.vi"("data"=w1513, "Active Sheet"=w1512, "Header Rows to remove"=3, "sub array start"=w1518, "error in (no error)"=w1520) -> ("row max value"=w1516:i32, "column max value"=w1511:i32, 13:"start of last occupied row"=w1515:cluster{"row":i32, "column":i32}, 14:"start of last occupied row"=w1510:string, "error out"=w1517:errorcluster)  [unwired: 4 in, 2 out]
                n621 = local write "last occupied cell's name"(w1510) -> ()
                n622 = local write "row max value"(w1511) -> ()
              }
            }
            n623 = local read "Found Quanta Sonde Com Port"() -> (w1442:refnum<visa-resource-name>)
            n624 = Equal?(x=w1442, y=refnum<visa-resource-name> refnum ("RS232 Port Out")) -> (x = y?=w1444:bool)
            n625 = case shown="False" w1444 {
              tunnel: w1442 -> [w1472 _]
              tunnel: [w1482 w1506] -> w1445
              tunnel: w1452 -> [w1475 w1509]
              tunnel: [w1485 w1509] -> w1449
              tunnel: w1432 -> [w1481 w1508]
              tunnel: [w1480 w1496] -> w1431
              tunnel: [w1479 w1495] -> w1430
              tunnel: w1429 -> [w1478 w1507]
              tunnel: w1428 -> [_ w1492]
              frame False {
                n626 = control-ref of="Sonde Data Display"() -> (w1486:refnum<vi>)
                n627 = call "Calibrate pH Sensor.vi"("Calibration Standard"="pH Reference", "Error In (No Error)"=w1475, "Sensor Address In"="0", "RS232 Port In"=w1472) -> ("Error Out"=w1474:errorcluster, "Sensor Calibrate Response"=→"pH  Reference\nCalibrate Response":bool, "RS232 Port Out"=w1471:refnum<visa-resource-name>)  [unwired: 4 in, 1 out]
                n628 = local read "Sample Sheet Data Row Cluster 2"() -> (w1483:T2)
                n629 = call "SDI-12 Single Operation with output cluster.vi"("RS232 Port In"=w1471, "Sensor Address In"="0", "Sonde Data Ctl Refnum"=w1486, "Error In (No Error)"=w1474, "Time Array In"=w1481, "Measurement Array In"=w1478) -> ("time array out"=w1480:dbl[], "Measurement  array Out"=w1479:dbl[][], "output cluster"=w1484:T1, "Temperature"=w1488:cluster{"Y":dbl[], "Y":dbl[]}[], "Sonde Data Display"=w1487:T14, "Error Out"=w1485:errorcluster)  [unwired: 12 in, 4 out]
                n630 = Bundle By Name(cluster=w1483, "Sonde Data Cluster"=w1484) -> (w1482:T2)
                n631 = local write "Temperature"(w1488) -> ()
                n632 = local write "Sonde Data Display"(w1487) -> ()
              }
              frame True {
                n633 = Get Date/Time In Seconds() -> (seconds since 1Jan1904=w1498:timestamp)
                n634 = To Double Precision Float(number=w1498) -> (double precision float=w1497:dbl)
                n635 = local read "Sample Sheet Data Row Cluster 2"() -> (w1506:T2)
                n636 = Subtract(x=w1497, y=w1492) -> (x-y=w1490:dbl)
                n637 = local write "Current Time (s)"(w1490) -> ()
                n638 = Unbundle By Name(w1506) -> ("Sonde Data Cluster.Temp"=w1491:dbl, "Sonde Data Cluster.pH"=w1505:dbl, "Sonde Data Cluster.Specific\nConductance"=w1504:dbl, "Sonde Data Cluster.Salinity"=w1503:dbl, "Sonde Data Cluster.Dissolved\nOxygen"=w1502:dbl, "Sonde Data Cluster.ORP"=w1501:dbl)  [unwired: 1 out]
                n639 = Build Array(w1491, w1505, w1504, w1503, w1502, 0.0 ("element"), w1501) -> (w1499:dbl[])
                n640 = Build Array (concatenate)(w1507, w1499) -> (w1495:dbl[][])
                n641 = Build Array (concatenate)(w1508, w1490) -> (w1496:dbl[])
                n642 = call "format into Sonde Vertical Graph Data Input.vi"("Sonde Measurement Array"=w1495, "Time Array"=w1496) -> ("Sonde Data Display"=w1494:T14, "Temperature"=w1493:cluster{"X":dbl[], "Y":dbl[]}[])  [unwired: 8 in]
                n643 = local write "Temperature"(w1493) -> ()
                n644 = local write "Sonde Data Display"(w1494) -> ()
              }
            }
            n645 = local write "Sample Sheet Data Row Cluster 2"(w1445) -> ()
            n646 = call "write out sonde row.vi"("NI_report in"=w1448, "Columns"=w1451, "Column of Volume"=w1450, "Sample Sheet Data Row Cluster"=w1445, "row index"=w1434, "error in (no error)"=w1449, "start of last occupied row"=w1446) -> ("NI_report out"=w1440:refnum<class "NI_report.lvclass">, "row index out"=w1433:i32, "error out"=w1441:errorcluster)  [unwired: 6 in]
            n647 = flat-sequence {
              tunnel: w1441 -> [w1470]
              tunnel: w1440 -> [w1469]
              tunnel: [w1468] -> w1439
              tunnel: [w1463] -> w1436
              tunnel: [w1461] -> w1435
              frame #0 {
                (unwired) 3 ("Header Rows to remove")
                n648 = call <vilib>:"Clear Errors.vi"("error in (no error)"=w1470) -> ("error out"=w1457:errorcluster)  [unwired: 5 in, 1 out]
                n649 = local read "Current Sample Sheet"() -> (w1459:string)
                n650 = call "get sample sheet data cells.vi"("error in (no error)"=w1457, "NI_report in"=w1469) -> ("error out"=w1464:errorcluster, "data"=w1465:string[][], "NI_report out"=w1468:refnum<class "NI_report.lvclass">, "left edge output cluster"=w1462:cluster{"row":i32, "column":i32})  [unwired: 5 in, 1 out]
                n651 = call "find last occupied cell.vi"("data"=w1465, "Active Sheet"=w1459, "Header Rows to remove"=3, "sub array start"=w1462, "error in (no error)"=w1464) -> ("row max value"=w1460:i32, 13:"start of last occupied row"=w1461:cluster{"row":i32, "column":i32}, 14:"start of last occupied row"=w1458:string, "error out"=w1463:errorcluster)  [unwired: 4 in, 3 out]
                n652 = Array Subset(array=w1465, index (col)=2 ("index")) -> ()  [unwired: 3 in, 1 out]
                n653 = local write "row max value"(w1460) -> ()
                n654 = local write "last occupied cell's name"(w1458) -> ()
              }
            }
          }
          frame "ORP Calibration Standard" {
            n655 = invoke on="Record Single Sample" class="Bool" method="Reinit To Default"(error in=w1542) -> (error out=w1541:errorcluster)  [unwired: 2 in, 2 out]
            n656 = call <vilib>:"Clear Errors.vi"("error in (no error)"=w1541) -> ("error out"=w1531:errorcluster)  [unwired: 5 in, 1 out]
            n657 = call "get sample sheet data cells.vi"("error in (no error)"=w1531, "NI_report in"=w1560) -> ("error out"=w1557:errorcluster, "data"=w1559:string[][], "NI_report out"=w1552:refnum<class "NI_report.lvclass">, "left edge output cluster"=w1558:cluster{"row":i32, "column":i32})  [unwired: 5 in, 1 out]
            n658 = flat-sequence {
              tunnel: w1557 -> [w1624]
              tunnel: [w1617] -> _
              tunnel: w1558 -> [w1622]
              tunnel: [w1621] -> w1556
              tunnel: [w1620] -> _
              tunnel: [w1619] -> w1550
              tunnel: w1559 -> [w1617]
              frame #0 {
                n659 = Array Subset(array=w1617, index (col)=2 ("index")) -> ()  [unwired: 3 in, 1 out]
                n660 = local read "Current Sample Sheet"() -> (w1616:string)
                n661 = call "find last occupied cell.vi"("data"=w1617, "Active Sheet"=w1616, "Header Rows to remove"=3, "sub array start"=w1622, "error in (no error)"=w1624) -> ("row max value"=w1620:i32, "column max value"=w1615:i32, 13:"start of last occupied row"=w1619:cluster{"row":i32, "column":i32}, 14:"start of last occupied row"=w1614:string, "error out"=w1621:errorcluster)  [unwired: 4 in, 2 out]
                n662 = local write "last occupied cell's name"(w1614) -> ()
                n663 = local write "row max value"(w1615) -> ()
              }
            }
            n664 = local read "Found Quanta Sonde Com Port"() -> (w1546:refnum<visa-resource-name>)
            n665 = Equal?(x=w1546, y=refnum<visa-resource-name> refnum ("RS232 Port Out")) -> (x = y?=w1548:bool)
            n666 = case shown="False" w1548 {
              tunnel: w1546 -> [w1576 _]
              tunnel: [w1586 w1610] -> w1549
              tunnel: w1556 -> [w1578 w1613]
              tunnel: [w1589 w1613] -> w1553
              tunnel: w1536 -> [w1585 w1612]
              tunnel: [w1584 w1600] -> w1535
              tunnel: [w1583 w1599] -> w1524
              tunnel: w1523 -> [w1582 w1611]
              tunnel: w1534 -> [_ w1596]
              frame False {
                n667 = control-ref of="Sonde Data Display"() -> (w1590:refnum<vi>)
                n668 = call "Calibrate ORP Sensor.vi"("Calibration Standard"="ORP Reference", "Error In (No Error)"=w1578, "Sensor Address In"="0", "RS232 Port In"=w1576) -> ("Error Out"=w1577:errorcluster, "Sensor Calibrate Response"=→"ORP  Reference\nCalibrate Response":bool, "RS232 Port Out"=w1575:refnum<visa-resource-name>)  [unwired: 4 in, 1 out]
                n669 = local read "Sample Sheet Data Row Cluster 2"() -> (w1587:T2)
                n670 = call "SDI-12 Single Operation with output cluster.vi"("RS232 Port In"=w1575, "Sensor Address In"="0", "Sonde Data Ctl Refnum"=w1590, "Error In (No Error)"=w1577, "Time Array In"=w1585, "Measurement Array In"=w1582) -> ("time array out"=w1584:dbl[], "Measurement  array Out"=w1583:dbl[][], "output cluster"=w1588:T1, "Temperature"=w1592:cluster{"Y":dbl[], "Y":dbl[]}[], "Sonde Data Display"=w1591:T14, "Error Out"=w1589:errorcluster)  [unwired: 12 in, 4 out]
                n671 = Bundle By Name(cluster=w1587, "Sonde Data Cluster"=w1588) -> (w1586:T2)
                n672 = local write "Temperature"(w1592) -> ()
                n673 = local write "Sonde Data Display"(w1591) -> ()
              }
              frame True {
                n674 = Get Date/Time In Seconds() -> (seconds since 1Jan1904=w1602:timestamp)
                n675 = To Double Precision Float(number=w1602) -> (double precision float=w1601:dbl)
                n676 = local read "Sample Sheet Data Row Cluster 2"() -> (w1610:T2)
                n677 = Subtract(x=w1601, y=w1596) -> (x-y=w1594:dbl)
                n678 = local write "Current Time (s)"(w1594) -> ()
                n679 = Unbundle By Name(w1610) -> ("Sonde Data Cluster.Temp"=w1595:dbl, "Sonde Data Cluster.pH"=w1609:dbl, "Sonde Data Cluster.Specific\nConductance"=w1608:dbl, "Sonde Data Cluster.Salinity"=w1607:dbl, "Sonde Data Cluster.Dissolved\nOxygen"=w1606:dbl, "Sonde Data Cluster.ORP"=w1605:dbl)  [unwired: 1 out]
                n680 = Build Array(w1595, w1609, w1608, w1607, w1606, 0.0 ("element"), w1605) -> (w1603:dbl[])
                n681 = Build Array (concatenate)(w1611, w1603) -> (w1599:dbl[][])
                n682 = Build Array (concatenate)(w1612, w1594) -> (w1600:dbl[])
                n683 = call "format into Sonde Vertical Graph Data Input.vi"("Sonde Measurement Array"=w1599, "Time Array"=w1600) -> ("Sonde Data Display"=w1598:T14, "Temperature"=w1597:cluster{"X":dbl[], "Y":dbl[]}[])  [unwired: 8 in]
                n684 = local write "Temperature"(w1597) -> ()
                n685 = local write "Sonde Data Display"(w1598) -> ()
              }
            }
            n686 = local write "Sample Sheet Data Row Cluster 2"(w1549) -> ()
            n687 = call "write out sonde row.vi"("NI_report in"=w1552, "Columns"=w1555, "Column of Volume"=w1554, "Sample Sheet Data Row Cluster"=w1549, "row index"=w1538, "error in (no error)"=w1553, "start of last occupied row"=w1550) -> ("NI_report out"=w1544:refnum<class "NI_report.lvclass">, "row index out"=w1537:i32, "error out"=w1545:errorcluster)  [unwired: 6 in]
            n688 = flat-sequence {
              tunnel: w1545 -> [w1574]
              tunnel: w1544 -> [w1573]
              tunnel: [w1572] -> w1543
              tunnel: [w1567] -> w1540
              tunnel: [w1565] -> w1539
              frame #0 {
                (unwired) 3 ("Header Rows to remove")
                n689 = call <vilib>:"Clear Errors.vi"("error in (no error)"=w1574) -> ("error out"=w1561:errorcluster)  [unwired: 5 in, 1 out]
                n690 = local read "Current Sample Sheet"() -> (w1563:string)
                n691 = call "get sample sheet data cells.vi"("error in (no error)"=w1561, "NI_report in"=w1573) -> ("error out"=w1568:errorcluster, "data"=w1569:string[][], "NI_report out"=w1572:refnum<class "NI_report.lvclass">, "left edge output cluster"=w1566:cluster{"row":i32, "column":i32})  [unwired: 5 in, 1 out]
                n692 = call "find last occupied cell.vi"("data"=w1569, "Active Sheet"=w1563, "Header Rows to remove"=3, "sub array start"=w1566, "error in (no error)"=w1568) -> ("row max value"=w1564:i32, 13:"start of last occupied row"=w1565:cluster{"row":i32, "column":i32}, 14:"start of last occupied row"=w1562:string, "error out"=w1567:errorcluster)  [unwired: 4 in, 3 out]
                n693 = Array Subset(array=w1569, index (col)=2 ("index")) -> ()  [unwired: 3 in, 1 out]
                n694 = local write "row max value"(w1564) -> ()
                n695 = local write "last occupied cell's name"(w1562) -> ()
              }
            }
          }
          frame "Salinity Calibration Standard" {
            n696 = invoke on="Record Single Sample" class="Bool" method="Reinit To Default"(error in=w1646) -> (error out=w1645:errorcluster)  [unwired: 2 in, 2 out]
            n697 = call <vilib>:"Clear Errors.vi"("error in (no error)"=w1645) -> ("error out"=w1633:errorcluster)  [unwired: 5 in, 1 out]
            n698 = call "get sample sheet data cells.vi"("error in (no error)"=w1633, "NI_report in"=w1664) -> ("error out"=w1661:errorcluster, "data"=w1663:string[][], "NI_report out"=w1656:refnum<class "NI_report.lvclass">, "left edge output cluster"=w1662:cluster{"row":i32, "column":i32})  [unwired: 5 in, 1 out]
            n699 = flat-sequence {
              tunnel: w1661 -> [w1728]
              tunnel: [w1721] -> _
              tunnel: w1662 -> [w1726]
              tunnel: [w1725] -> w1660
              tunnel: [w1724] -> _
              tunnel: [w1723] -> w1654
              tunnel: w1663 -> [w1721]
              frame #0 {
                n700 = Array Subset(array=w1721, index (col)=2 ("index")) -> ()  [unwired: 3 in, 1 out]
                n701 = local read "Current Sample Sheet"() -> (w1720:string)
                n702 = call "find last occupied cell.vi"("data"=w1721, "Active Sheet"=w1720, "Header Rows to remove"=3, "sub array start"=w1726, "error in (no error)"=w1728) -> ("row max value"=w1724:i32, "column max value"=w1719:i32, 13:"start of last occupied row"=w1723:cluster{"row":i32, "column":i32}, 14:"start of last occupied row"=w1718:string, "error out"=w1725:errorcluster)  [unwired: 4 in, 2 out]
                n703 = local write "last occupied cell's name"(w1718) -> ()
                n704 = local write "row max value"(w1719) -> ()
              }
            }
            n705 = local read "Found Quanta Sonde Com Port"() -> (w1650:refnum<visa-resource-name>)
            n706 = Equal?(x=w1650, y=refnum<visa-resource-name> refnum ("RS232 Port Out")) -> (x = y?=w1652:bool)
            n707 = case shown="False" w1652 {
              tunnel: w1650 -> [w1683 _]
              tunnel: [w1690 w1714] -> w1653
              tunnel: w1660 -> [w1681 w1717]
              tunnel: [w1693 w1717] -> w1657
              tunnel: w1640 -> [w1689 w1716]
              tunnel: [w1688 w1704] -> w1639
              tunnel: [w1687 w1703] -> w1638
              tunnel: w1637 -> [w1686 w1715]
              tunnel: w1636 -> [_ w1700]
              frame False {
                n708 = call "Calibrate Salinity Sensor.vi"("Calibration Standard"="Salinity \nReference", "Error In (No Error)"=w1681, "Sensor Address In"="0", "RS232 Port In"=w1683) -> ("Error Out"=w1680:errorcluster, "Sensor Calibrate Response"=→"Salinity  Reference\nCalibrate Response":bool, "RS232 Port Out"=w1682:refnum<visa-resource-name>)  [unwired: 4 in, 1 out]
                n709 = control-ref of="Sonde Data Display"() -> (w1694:refnum<vi>)
                n710 = local read "Sample Sheet Data Row Cluster 2"() -> (w1691:T2)
                n711 = call "SDI-12 Single Operation with output cluster.vi"("RS232 Port In"=w1682, "Sensor Address In"="0", "Sonde Data Ctl Refnum"=w1694, "Error In (No Error)"=w1680, "Time Array In"=w1689, "Measurement Array In"=w1686) -> ("time array out"=w1688:dbl[], "Measurement  array Out"=w1687:dbl[][], "output cluster"=w1692:T1, "Temperature"=w1696:cluster{"Y":dbl[], "Y":dbl[]}[], "Sonde Data Display"=w1695:T14, "Error Out"=w1693:errorcluster)  [unwired: 12 in, 4 out]
                n712 = local write "Temperature"(w1696) -> ()
                n713 = local write "Sonde Data Display"(w1695) -> ()
                n714 = Bundle By Name(cluster=w1691, "Sonde Data Cluster"=w1692) -> (w1690:T2)
              }
              frame True {
                n715 = Get Date/Time In Seconds() -> (seconds since 1Jan1904=w1706:timestamp)
                n716 = To Double Precision Float(number=w1706) -> (double precision float=w1705:dbl)
                n717 = local read "Sample Sheet Data Row Cluster 2"() -> (w1714:T2)
                n718 = Subtract(x=w1705, y=w1700) -> (x-y=w1698:dbl)
                n719 = local write "Current Time (s)"(w1698) -> ()
                n720 = Unbundle By Name(w1714) -> ("Sonde Data Cluster.Temp"=w1699:dbl, "Sonde Data Cluster.pH"=w1713:dbl, "Sonde Data Cluster.Specific\nConductance"=w1712:dbl, "Sonde Data Cluster.Salinity"=w1711:dbl, "Sonde Data Cluster.Dissolved\nOxygen"=w1710:dbl, "Sonde Data Cluster.ORP"=w1709:dbl)  [unwired: 1 out]
                n721 = Build Array(w1699, w1713, w1712, w1711, w1710, 0.0 ("element"), w1709) -> (w1707:dbl[])
                n722 = Build Array (concatenate)(w1715, w1707) -> (w1703:dbl[][])
                n723 = Build Array (concatenate)(w1716, w1698) -> (w1704:dbl[])
                n724 = call "format into Sonde Vertical Graph Data Input.vi"("Sonde Measurement Array"=w1703, "Time Array"=w1704) -> ("Sonde Data Display"=w1702:T14, "Temperature"=w1701:cluster{"X":dbl[], "Y":dbl[]}[])  [unwired: 8 in]
                n725 = local write "Temperature"(w1701) -> ()
                n726 = local write "Sonde Data Display"(w1702) -> ()
              }
            }
            n727 = local write "Sample Sheet Data Row Cluster 2"(w1653) -> ()
            n728 = call "write out sonde row.vi"("NI_report in"=w1656, "Columns"=w1659, "Column of Volume"=w1658, "Sample Sheet Data Row Cluster"=w1653, "row index"=w1642, "error in (no error)"=w1657, "start of last occupied row"=w1654) -> ("NI_report out"=w1648:refnum<class "NI_report.lvclass">, "row index out"=w1641:i32, "error out"=w1649:errorcluster)  [unwired: 6 in]
            n729 = flat-sequence {
              tunnel: w1649 -> [w1678]
              tunnel: w1648 -> [w1677]
              tunnel: [w1676] -> w1647
              tunnel: [w1671] -> w1644
              tunnel: [w1669] -> w1643
              frame #0 {
                (unwired) 3 ("Header Rows to remove")
                n730 = call <vilib>:"Clear Errors.vi"("error in (no error)"=w1678) -> ("error out"=w1665:errorcluster)  [unwired: 5 in, 1 out]
                n731 = local read "Current Sample Sheet"() -> (w1667:string)
                n732 = call "get sample sheet data cells.vi"("error in (no error)"=w1665, "NI_report in"=w1677) -> ("error out"=w1672:errorcluster, "data"=w1673:string[][], "NI_report out"=w1676:refnum<class "NI_report.lvclass">, "left edge output cluster"=w1670:cluster{"row":i32, "column":i32})  [unwired: 5 in, 1 out]
                n733 = call "find last occupied cell.vi"("data"=w1673, "Active Sheet"=w1667, "Header Rows to remove"=3, "sub array start"=w1670, "error in (no error)"=w1672) -> ("row max value"=w1668:i32, 13:"start of last occupied row"=w1669:cluster{"row":i32, "column":i32}, 14:"start of last occupied row"=w1666:string, "error out"=w1671:errorcluster)  [unwired: 4 in, 3 out]
                n734 = Array Subset(array=w1673, index (col)=2 ("index")) -> ()  [unwired: 3 in, 1 out]
                n735 = local write "row max value"(w1668) -> ()
                n736 = local write "last occupied cell's name"(w1666) -> ()
              }
            }
          }
          frame "DO Calibration Standard" {
            n737 = invoke on="Record Single Sample" class="Bool" method="Reinit To Default"(error in=w1750) -> (error out=w1749:errorcluster)  [unwired: 2 in, 2 out]
            n738 = call <vilib>:"Clear Errors.vi"("error in (no error)"=w1749) -> ("error out"=w1737:errorcluster)  [unwired: 5 in, 1 out]
            n739 = call "get sample sheet data cells.vi"("error in (no error)"=w1737, "NI_report in"=w1768) -> ("error out"=w1765:errorcluster, "data"=w1767:string[][], "NI_report out"=w1760:refnum<class "NI_report.lvclass">, "left edge output cluster"=w1766:cluster{"row":i32, "column":i32})  [unwired: 5 in, 1 out]
            n740 = flat-sequence {
              tunnel: w1765 -> [w1831]
              tunnel: [w1824] -> _
              tunnel: w1766 -> [w1829]
              tunnel: [w1828] -> w1764
              tunnel: [w1827] -> _
              tunnel: [w1826] -> w1758
              tunnel: w1767 -> [w1824]
              frame #0 {
                n741 = Array Subset(array=w1824, index (col)=2 ("index")) -> ()  [unwired: 3 in, 1 out]
                n742 = local read "Current Sample Sheet"() -> (w1823:string)
                n743 = call "find last occupied cell.vi"("data"=w1824, "Active Sheet"=w1823, "Header Rows to remove"=3, "sub array start"=w1829, "error in (no error)"=w1831) -> ("row max value"=w1827:i32, "column max value"=w1822:i32, 13:"start of last occupied row"=w1826:cluster{"row":i32, "column":i32}, 14:"start of last occupied row"=w1821:string, "error out"=w1828:errorcluster)  [unwired: 4 in, 2 out]
                n744 = local write "last occupied cell's name"(w1821) -> ()
                n745 = local write "row max value"(w1822) -> ()
              }
            }
            n746 = local read "Found Quanta Sonde Com Port"() -> (w1754:refnum<visa-resource-name>)
            n747 = Equal?(x=w1754, y=refnum<visa-resource-name> refnum ("RS232 Port Out")) -> (x = y?=w1756:bool)
            n748 = case shown="False" w1756 {
              tunnel: w1754 -> [w1786 _]
              tunnel: [w1793 w1817] -> w1757
              tunnel: w1764 -> [w1788 w1820]
              tunnel: [w1796 w1820] -> w1761
              tunnel: w1744 -> [w1792 w1819]
              tunnel: [w1791 w1807] -> w1743
              tunnel: [w1790 w1806] -> w1742
              tunnel: w1741 -> [w1789 w1818]
              tunnel: w1740 -> [_ w1803]
              frame False {
                n749 = call "Calibrate DO Sensor.vi"("Calibration Standard"="DO \nReference", "Error In (No Error)"=w1788, "Sensor Address In"="0", "RS232 Port In"=w1786) -> ("Error Out"=w1787:errorcluster, "Sensor Calibrate Response"=→"DO  Reference\nCalibrate Response":bool, "RS232 Port Out"=w1785:refnum<visa-resource-name>)  [unwired: 4 in, 1 out]
                n750 = control-ref of="Sonde Data Display"() -> (w1797:refnum<vi>)
                n751 = local read "Sample Sheet Data Row Cluster 2"() -> (w1794:T2)
                n752 = call "SDI-12 Single Operation with output cluster.vi"("RS232 Port In"=w1785, "Sensor Address In"="0", "Sonde Data Ctl Refnum"=w1797, "Error In (No Error)"=w1787, "Time Array In"=w1792, "Measurement Array In"=w1789) -> ("time array out"=w1791:dbl[], "Measurement  array Out"=w1790:dbl[][], "output cluster"=w1795:T1, "Temperature"=w1799:cluster{"Y":dbl[], "Y":dbl[]}[], "Sonde Data Display"=w1798:T14, "Error Out"=w1796:errorcluster)  [unwired: 12 in, 4 out]
                n753 = local write "Temperature"(w1799) -> ()
                n754 = local write "Sonde Data Display"(w1798) -> ()
                n755 = Bundle By Name(cluster=w1794, "Sonde Data Cluster"=w1795) -> (w1793:T2)
              }
              frame True {
                n756 = Get Date/Time In Seconds() -> (seconds since 1Jan1904=w1809:timestamp)
                n757 = To Double Precision Float(number=w1809) -> (double precision float=w1808:dbl)
                n758 = local read "Sample Sheet Data Row Cluster 2"() -> (w1817:T2)
                n759 = Subtract(x=w1808, y=w1803) -> (x-y=w1801:dbl)
                n760 = local write "Current Time (s)"(w1801) -> ()
                n761 = Unbundle By Name(w1817) -> ("Sonde Data Cluster.Temp"=w1802:dbl, "Sonde Data Cluster.pH"=w1816:dbl, "Sonde Data Cluster.Specific\nConductance"=w1815:dbl, "Sonde Data Cluster.Salinity"=w1814:dbl, "Sonde Data Cluster.Dissolved\nOxygen"=w1813:dbl, "Sonde Data Cluster.ORP"=w1812:dbl)  [unwired: 1 out]
                n762 = Build Array(w1802, w1816, w1815, w1814, w1813, 0.0 ("element"), w1812) -> (w1810:dbl[])
                n763 = Build Array (concatenate)(w1818, w1810) -> (w1806:dbl[][])
                n764 = Build Array (concatenate)(w1819, w1801) -> (w1807:dbl[])
                n765 = call "format into Sonde Vertical Graph Data Input.vi"("Sonde Measurement Array"=w1806, "Time Array"=w1807) -> ("Sonde Data Display"=w1805:T14, "Temperature"=w1804:cluster{"X":dbl[], "Y":dbl[]}[])  [unwired: 8 in]
                n766 = local write "Temperature"(w1804) -> ()
                n767 = local write "Sonde Data Display"(w1805) -> ()
              }
            }
            n768 = local write "Sample Sheet Data Row Cluster 2"(w1757) -> ()
            n769 = call "write out sonde row.vi"("NI_report in"=w1760, "Columns"=w1763, "Column of Volume"=w1762, "Sample Sheet Data Row Cluster"=w1757, "row index"=w1746, "error in (no error)"=w1761, "start of last occupied row"=w1758) -> ("NI_report out"=w1752:refnum<class "NI_report.lvclass">, "row index out"=w1745:i32, "error out"=w1753:errorcluster)  [unwired: 6 in]
            n770 = flat-sequence {
              tunnel: w1753 -> [w1781]
              tunnel: w1752 -> [w1780]
              tunnel: [w1779] -> w1751
              tunnel: [w1775] -> w1748
              tunnel: [w1773] -> w1747
              frame #0 {
                (unwired) 3 ("Header Rows to remove")
                n771 = call <vilib>:"Clear Errors.vi"("error in (no error)"=w1781) -> ("error out"=w1769:errorcluster)  [unwired: 5 in, 1 out]
                n772 = local read "Current Sample Sheet"() -> (w1771:string)
                n773 = call "get sample sheet data cells.vi"("error in (no error)"=w1769, "NI_report in"=w1780) -> ("error out"=w1776:errorcluster, "data"=w1777:string[][], "NI_report out"=w1779:refnum<class "NI_report.lvclass">, "left edge output cluster"=w1774:cluster{"row":i32, "column":i32})  [unwired: 5 in, 1 out]
                n774 = call "find last occupied cell.vi"("data"=w1777, "Active Sheet"=w1771, "Header Rows to remove"=3, "sub array start"=w1774, "error in (no error)"=w1776) -> ("row max value"=w1772:i32, 13:"start of last occupied row"=w1773:cluster{"row":i32, "column":i32}, 14:"start of last occupied row"=w1770:string, "error out"=w1775:errorcluster)  [unwired: 4 in, 3 out]
                n775 = local write "row max value"(w1772) -> ()
                n776 = local write "last occupied cell's name"(w1770) -> ()
              }
            }
          }
          frame "SC Calibration Standard" {
            n777 = invoke on="Record Single Sample" class="Bool" method="Reinit To Default"(error in=w1853) -> (error out=w1852:errorcluster)  [unwired: 2 in, 2 out]
            n778 = call <vilib>:"Clear Errors.vi"("error in (no error)"=w1852) -> ("error out"=w1840:errorcluster)  [unwired: 5 in, 1 out]
            n779 = call "get sample sheet data cells.vi"("error in (no error)"=w1840, "NI_report in"=w1871) -> ("error out"=w1868:errorcluster, "data"=w1870:string[][], "NI_report out"=w1863:refnum<class "NI_report.lvclass">, "left edge output cluster"=w1869:cluster{"row":i32, "column":i32})  [unwired: 5 in, 1 out]
            n780 = flat-sequence {
              tunnel: w1868 -> [w1934]
              tunnel: [w1928] -> _
              tunnel: w1869 -> [w1932]
              tunnel: [w1931] -> w1867
              tunnel: [w1930] -> _
              tunnel: [w1929] -> w1861
              tunnel: w1870 -> [w1928]
              frame #0 {
                n781 = local read "Current Sample Sheet"() -> (w1927:string)
                n782 = call "find last occupied cell.vi"("data"=w1928, "Active Sheet"=w1927, "Header Rows to remove"=3, "sub array start"=w1932, "error in (no error)"=w1934) -> ("row max value"=w1930:i32, "column max value"=w1926:i32, 13:"start of last occupied row"=w1929:cluster{"row":i32, "column":i32}, 14:"start of last occupied row"=w1925:string, "error out"=w1931:errorcluster)  [unwired: 4 in, 2 out]
                n783 = local write "last occupied cell's name"(w1925) -> ()
                n784 = local write "row max value"(w1926) -> ()
              }
            }
            n785 = local read "Found Quanta Sonde Com Port"() -> (w1857:refnum<visa-resource-name>)
            n786 = Equal?(x=w1857, y=refnum<visa-resource-name> refnum ("RS232 Port Out")) -> (x = y?=w1859:bool)
            n787 = case shown="False" w1859 {
              tunnel: w1857 -> [w1891 _]
              tunnel: [w1897 w1921] -> w1860
              tunnel: w1867 -> [w1889 w1924]
              tunnel: [w1900 w1924] -> w1864
              tunnel: w1847 -> [w1896 w1923]
              tunnel: [w1895 w1911] -> w1846
              tunnel: [w1894 w1910] -> w1845
              tunnel: w1844 -> [w1893 w1922]
              tunnel: w1843 -> [_ w1907]
              frame False {
                n788 = call "Calibrate SC Sensor.vi"("Calibration Standard"="SC \nReference", "Error In (No Error)"=w1889, "Sensor Address In"="0", "RS232 Port In"=w1891) -> ("Error Out"=w1888:errorcluster, "Sensor Calibrate Response"=→"SC  Reference\nCalibrate Response":bool, "RS232 Port Out"=w1890:refnum<visa-resource-name>)  [unwired: 4 in, 1 out]
                n789 = control-ref of="Sonde Data Display"() -> (w1901:refnum<vi>)
                n790 = local read "Sample Sheet Data Row Cluster 2"() -> (w1898:T2)
                n791 = call <vilib>:"Clear Errors.vi"("error in (no error)"=w1888) -> ("error out"=w1885:errorcluster)  [unwired: 5 in, 1 out]
                n792 = call "SDI-12 Single Operation with output cluster.vi"("RS232 Port In"=w1890, "Sensor Address In"="0", "Sonde Data Ctl Refnum"=w1901, "Error In (No Error)"=w1885, "Time Array In"=w1896, "Measurement Array In"=w1893) -> ("time array out"=w1895:dbl[], "Measurement  array Out"=w1894:dbl[][], "output cluster"=w1899:T1, "Temperature"=w1903:cluster{"Y":dbl[], "Y":dbl[]}[], "Sonde Data Display"=w1902:T14, "Error Out"=w1900:errorcluster)  [unwired: 12 in, 4 out]
                n793 = local write "Temperature"(w1903) -> ()
                n794 = local write "Sonde Data Display"(w1902) -> ()
                n795 = Bundle By Name(cluster=w1898, "Sonde Data Cluster"=w1899) -> (w1897:T2)
              }
              frame True {
                n796 = Get Date/Time In Seconds() -> (seconds since 1Jan1904=w1913:timestamp)
                n797 = To Double Precision Float(number=w1913) -> (double precision float=w1912:dbl)
                n798 = local read "Sample Sheet Data Row Cluster 2"() -> (w1921:T2)
                n799 = Subtract(x=w1912, y=w1907) -> (x-y=w1905:dbl)
                n800 = local write "Current Time (s)"(w1905) -> ()
                n801 = Unbundle By Name(w1921) -> ("Sonde Data Cluster.Temp"=w1906:dbl, "Sonde Data Cluster.pH"=w1920:dbl, "Sonde Data Cluster.Specific\nConductance"=w1919:dbl, "Sonde Data Cluster.Salinity"=w1918:dbl, "Sonde Data Cluster.Dissolved\nOxygen"=w1917:dbl, "Sonde Data Cluster.ORP"=w1916:dbl)  [unwired: 1 out]
                n802 = Build Array(w1906, w1920, w1919, w1918, w1917, 0.0 ("element"), w1916) -> (w1914:dbl[])
                n803 = Build Array (concatenate)(w1922, w1914) -> (w1910:dbl[][])
                n804 = Build Array (concatenate)(w1923, w1905) -> (w1911:dbl[])
                n805 = call "format into Sonde Vertical Graph Data Input.vi"("Sonde Measurement Array"=w1910, "Time Array"=w1911) -> ("Sonde Data Display"=w1909:T14, "Temperature"=w1908:cluster{"X":dbl[], "Y":dbl[]}[])  [unwired: 8 in]
                n806 = local write "Temperature"(w1908) -> ()
                n807 = local write "Sonde Data Display"(w1909) -> ()
              }
            }
            n808 = local write "Sample Sheet Data Row Cluster 2"(w1860) -> ()
            n809 = call "write out sonde row.vi"("NI_report in"=w1863, "Columns"=w1866, "Column of Volume"=w1865, "Sample Sheet Data Row Cluster"=w1860, "row index"=w1849, "error in (no error)"=w1864, "start of last occupied row"=w1861) -> ("NI_report out"=w1855:refnum<class "NI_report.lvclass">, "row index out"=w1848:i32, "error out"=w1856:errorcluster)  [unwired: 6 in]
            n810 = flat-sequence {
              tunnel: w1856 -> [w1884]
              tunnel: w1855 -> [w1883]
              tunnel: [w1882] -> w1854
              tunnel: [w1878] -> w1851
              tunnel: [w1876] -> w1850
              frame #0 {
                (unwired) 3 ("Header Rows to remove")
                (unwired) 2 ("index")
                n811 = call <vilib>:"Clear Errors.vi"("error in (no error)"=w1884) -> ("error out"=w1872:errorcluster)  [unwired: 5 in, 1 out]
                n812 = local read "Current Sample Sheet"() -> (w1874:string)
                n813 = call "get sample sheet data cells.vi"("error in (no error)"=w1872, "NI_report in"=w1883) -> ("error out"=w1879:errorcluster, "data"=w1880:string[][], "NI_report out"=w1882:refnum<class "NI_report.lvclass">, "left edge output cluster"=w1877:cluster{"row":i32, "column":i32})  [unwired: 5 in, 1 out]
                n814 = call "find last occupied cell.vi"("data"=w1880, "Active Sheet"=w1874, "Header Rows to remove"=3, "sub array start"=w1877, "error in (no error)"=w1879) -> ("row max value"=w1875:i32, 13:"start of last occupied row"=w1876:cluster{"row":i32, "column":i32}, 14:"start of last occupied row"=w1873:string, "error out"=w1878:errorcluster)  [unwired: 4 in, 3 out]
                n815 = local write "row max value"(w1875) -> ()
                n816 = local write "last occupied cell's name"(w1873) -> ()
              }
            }
          }
          frame "Write Sonde Sample Sheet" {
            n817 = flat-sequence {
              tunnel: w1962 -> [w1979]
              tunnel: w1961 -> [w1978]
              tunnel: w1959 -> [w1975]
              tunnel: w1958 -> [w1974]
              tunnel: w1957 -> [w1973]
              tunnel: [w1972] -> w1956
              tunnel: w1955 -> [w1971]
              tunnel: w1954 -> [w1970]
              tunnel: w1953 -> [w1968]
              tunnel: [w1966] -> w1951
              tunnel: [w1965] -> w1950
              tunnel: [w1964] -> w1949
              tunnel: w1938 -> [w1963]
              frame #0 {
                n818 = Not Equal?(x=w1971, y=w1970) -> (x != y?=w1969:bool)
                n819 = invoke on="Update Sonde" class="Bool (strict)" method="Reinit To Default"() -> ()  [unwired: 3 in, 3 out]
                n820 = Decrement(x=w1963) -> (x-1=w1964:i32)
                n821 = case shown="True" w1969 {
                  tunnel: w1979 -> [w1982 w1989]
                  tunnel: w1968 -> [_ w1988]
                  tunnel: w1978 -> [w1981 w1987]
                  tunnel: [w1981 w1986] -> w1977
                  tunnel: [w1982 w1985] -> w1976
                  tunnel: w1973 -> [w1980 w1984]
                  tunnel: [w1980 w1983] -> w1972
                  frame False {
                  }
                  frame True {
                    n822 = flat-sequence {
                      tunnel: [w1998] -> w1985
                      tunnel: w1989 -> [w1997]
                      tunnel: w1988 -> [w1994]
                      tunnel: w1987 -> [w1993]
                      tunnel: [w1992] -> w1986
                      tunnel: w1984 -> [w1991]
                      tunnel: [w1990] -> w1983
                      frame #0 {
                        n823 = Increment(x=w1991) -> (x+1=w1990:i32)
                        n824 = call "write comment cell with column offset.vi"("Column Relative?"=TRUE, "comment string"="done", "error in (no error)"=w1993, "start of last occupied row"=w1994, "NI_report in"=w1997) -> ("error out"=w1992:errorcluster, "NI_report out"=w1998:refnum<class "NI_report.lvclass">)  [unwired: 5 in]
                      }
                    }
                  }
                }
                n825 = call "open select sample sheet.vi"("Number of Sample Sheets"=w1974, "error in (no error)"=w1977, "Worksheet Names"=w1975, "Active Sample Sheet"=w1972, "NI_report in"=w1976) -> ("error out"=w1966:errorcluster, "Current Sample Sheet"=w1967:string, "NI_report out"=w1965:refnum<class "NI_report.lvclass">)  [unwired: 3 in, 1 out]
                n826 = local write "Current Sample Sheet"(w1967) -> ()
              }
            }
            n827 = flat-sequence {
              tunnel: w1938 -> [w2013]
              frame #0 {
                n828 = local read "Sonde Data Array"() -> (w2016:T12[])
                n829 = Index Array(array=w2016, index=w2013) -> (element=w2018:T12)
                n830 = Bundle By Name(cluster=w2018, "Final"=TRUE) -> (w2014:T12)
                n831 = Replace Array Subset(array=w2016, new element=w2014, index=w2013) -> (w2015:T12[])
                n832 = local write "Sonde Data Array"(w2015) -> ()
              }
            }
            n833 = flat-sequence {
              tunnel: [w2011] -> w1960
              tunnel: [w2010] -> w1952
              tunnel: w1951 -> [w2009]
              tunnel: w1950 -> [w2008]
              tunnel: [w2000] -> w1944
              frame #0 {
                n834 = local read "Current Sample Sheet"() -> (w2002:string)
                n835 = call "get sample sheet data cells.vi"("error in (no error)"=w2009, "NI_report in"=w2008) -> ("error out"=w2012:errorcluster, "data"=w2006:string[][], "NI_report out"=w2011:refnum<class "NI_report.lvclass">, "left edge output cluster"=w2004:cluster{"row":i32, "column":i32})  [unwired: 5 in, 1 out]
                n836 = Array Subset(array=w2006, index (col)=2 ("index")) -> ()  [unwired: 3 in, 1 out]
                n837 = call "find last occupied cell.vi"("Active Sheet"=w2002, "Header Rows to remove"=3, "sub array start"=w2004, "error in (no error)"=w2012) -> ("row max value"=w2003:i32, 13:"start of last occupied row"=w2010:cluster{"row":i32, "column":i32}, 14:"start of last occupied row"=w2001:string, "error out"=w2000:errorcluster)  [unwired: 5 in, 3 out]
                n838 = local write "row max value"(w2003) -> ()
                n839 = local write "last occupied cell's name"(w2001) -> ()
                n840 = local write "Sonde Data Array"(T12[] [{"Head"=0.0, "Depth"=0.0, "Time"="19:00", "Cumulative\nVolume"=0.0, "Sp. Conductance"={"Value"=0.506, "%"=0.0, "Tol."=TRUE}, "Dissolved Oxygen"={"Value"=35.14, "%"=0.0, "Tol."=TRUE}, "pH"={"Value"=4.81, "%"=0.0, "Tol."=TRUE}, "ORP"={"Value"=390.0, "%"=0.0, "Tol."=TRUE}, "Temperature"={"Value"=23.86, "%"=0.0, "Tol."=TRUE}, "Salinity"={"Value"=0.24, "%"=0.0, "Tol."=TRUE}, "Final Tol."=TRUE, "Final"=FALSE}, {"Head"=0.0, "Depth"=0.0, "Time"="19:00", "Cumulative\nVolume"=0.0, "Sp. Conductance"={"Value"=0.506, "%"=0.0, "Tol."=TRUE}, "Dissolved Oxygen"={"Value"=35.12, "%"=0.0, "Tol."=TRUE}, "pH"={"Value"=4.81, "%"=0.0, "Tol."=TRUE}, "ORP"={"Value"=390.0, "%"=0.0, "Tol."=TRUE}, "Temperature"={"Value"=23.89, "%"=0.0, "Tol."=TRUE}, "Salinity"={"Value"=0.24, "%"=0.0, "Tol."=TRUE}, "Final Tol."=TRUE, "Final"=FALSE}, {"Head"=0.0, "Depth"=0.0, "Time"="19:00", "Cumulative\nVolume"=0.0, "Sp. Conductance"={"Value"=0.506, "%"=0.0, "Tol."=TRUE}, "Dissolved Oxygen"={"Value"=35.14, "%"=0.0, "Tol."=TRUE}, "pH"={"Value"=4.81, "%"=0.0, "Tol."=TRUE}, "ORP"={"Value"=390.0, "%"=0.0, "Tol."=TRUE}, "Temperature"={"Value"=23.86, "%"=0.0, "Tol."=TRUE}, "Salinity"={"Value"=0.24, "%"=0.0, "Tol."=TRUE}, "Final Tol."=TRUE, "Final"=FALSE}, {"Head"=0.0, "Depth"=0.0, "Time"="", "Cumulative\nVolume"=0.0, "Sp. Conductance"={"Value"=0.0, "%"=0.0, "Tol."=FALSE}, "Dissolved Oxygen"={"Value"=0.0, "%"=0.0, "Tol."=FALSE}, "pH"={"Value"=0.0, "%"=0.0, "Tol."=FALSE}, "ORP"={"Value"=0.0, "%"=0.0, "Tol."=FALSE}, "Temperature"={"Value"=0.0, "%"=0.0, "Tol."=FALSE}, "Salinity"={"Value"=0.0, "%"=0.0, "Tol."=FALSE}, "Final Tol."=FALSE, "Final"=FALSE}, {"Head"=0.0, "Depth"=0.0, "Time"="", "Cumulative\nVolume"=0.0, "Sp. Conductance"={"Value"=0.0, "%"=0.0, "Tol."=FALSE}, "Dissolved Oxygen"={"Value"=0.0, "%"=0.0, "Tol."=FALSE}, "pH"={"Value"=0.0, "%"=0.0, "Tol."=FALSE}, "ORP"={"Value"=0.0, "%"=0.0, "Tol."=FALSE}, "Temperature"={"Value"=0.0, "%"=0.0, "Tol."=FALSE}, "Salinity"={"Value"=0.0, "%"=0.0, "Tol."=FALSE}, "Final Tol."=FALSE, "Final"=FALSE}, {"Head"=0.0, "Depth"=0.0, "Time"="", "Cumulative\nVolume"=0.0, "Sp. Conductance"={"Value"=0.0, "%"=0.0, "Tol."=FALSE}, "Dissolved Oxygen"={"Value"=0.0, "%"=0.0, "Tol."=FALSE}, "pH"={"Value"=0.0, "%"=0.0, "Tol."=FALSE}, "ORP"={"Value"=0.0, "%"=0.0, "Tol."=FALSE}, "Temperature"={"Value"=0.0, "%"=0.0, "Tol."=FALSE}, "Salinity"={"Value"=0.0, "%"=0.0, "Tol."=FALSE}, "Final Tol."=FALSE, "Final"=FALSE}, {"Head"=0.0, "Depth"=0.0, "Time"="", "Cumulative\nVolume"=0.0, "Sp. Conductance"={"Value"=0.0, "%"=0.0, "Tol."=FALSE}, "Dissolved Oxygen"={"Value"=0.0, "%"=0.0, "Tol."=FALSE}, "pH"={"Value"=0.0, "%"=0.0, "Tol."=FALSE}, "ORP"={"Value"=0.0, "%"=0.0, "Tol."=FALSE}, "Temperature"={"Value"=0.0, "%"=0.0, "Tol."=FALSE}, "Salinity"={"Value"=0.0, "%"=0.0, "Tol."=FALSE}, "Final Tol."=FALSE, "Final"=FALSE}, {"Head"=0.0, "Depth"=0.0, "Time"="", "Cumulative\nVolume"=0.0, "Sp. Conductance"={"Value"=0.0, "%"=0.0, "Tol."=FALSE}, "Dissolved Oxygen"={"Value"=0.0, "%"=0.0, "Tol."=FALSE}, "pH"={"Value"=0.0, "%"=0.0, "Tol."=FALSE}, "ORP"={"Value"=0.0, "%"=0.0, "Tol."=FALSE}, "Temperature"={"Value"=0.0, "%"=0.0, "Tol."=FALSE}, "Salinity"={"Value"=0.0, "%"=0.0, "Tol."=FALSE}, "Final Tol."=FALSE, "Final"=FALSE}, {"Head"=0.0, "Depth"=0.0, "Time"="", "Cumulative\nVolume"=0.0, "Sp. Conductance"={"Value"=0.0, "%"=0.0, "Tol."=FALSE}, "Dissolved Oxygen"={"Value"=0.0, "%"=0.0, "Tol."=FALSE}, "pH"={"Value"=0.0, "%"=0.0, "Tol."=FALSE}, "ORP"={"Value"=0.0, "%"=0.0, "Tol."=FALSE}, "Temperature"={"Value"=0.0, "%"=0.0, "Tol."=FALSE}, "Salinity"={"Value"=0.0, "%"=0.0, "Tol."=FALSE}, "Final Tol."=FALSE, "Final"=FALSE}] ("Sonde Data Array")) -> ()
              }
            }
          }
          frame "Init" {
            n841 = flat-sequence {
              tunnel: w2041 -> [w2386]
              tunnel: [w2372] -> w2031
              tunnel: [w2371] -> w2030
              frame #0 {
                n842 = call "create DAQ strings.vi"("error in (no error)"=w2386, "MCC USB-DAQ Setup"="MCC USB-DAQ Setup") -> ("error IO"=w2379:errorcluster, "Descriptions"=w2377:string[], "delimited string"=w2380:string, "Array"=w2378:string[], "Voltage Range"=w2385:dbl[])  [unwired: 5 in]
                "delimited string" <- w2380
                "Active Channel Array" <- w2378
                "Voltage Range" <- w2385
                "Descriptions" <- w2377
                n843 = call "Physical Channels to Number of channels.vi"("error in (no error)"=w2379, "Physical Channel in"=w2380) -> ("error out"=w2381:errorcluster, "Number of Channels"=w2383:i32)  [unwired: 7 in, 1 out]
                "Number \nof Channels" <- w2383
                n844 = call "Calculate Rate from Num Channels and Max Rate.vi"("error in (no error)"=w2381, "Channel Data Rate S/s"="Channel \nData Rate S/s", "Number of Channels"=w2383) -> ("error out"=w2375:errorcluster, "Rate"=→"Rate":dbl)  [unwired: 7 in]
                n845 = for {
                  tunnel: w2378 -> [w2399] mode=indexing
                  tunnel: w2385 -> [w2398] mode=indexing
                  tunnel: [w2395] -> w2374 mode=indexing
                  shift-right: [w2396] -> w2373
                  shift-left: w2375 -> [w2394]
                  n846 = Negate(x=w2398) -> (-x=w2397:dbl)
                  n847 = call-poly <vilib>:"ULx Create Virtual Channel.vi"("maximum value"=w2398, "minimum value"=w2397, "physical channels"=w2399, "error in"=w2394) -> ("task out"=w2395:refnum<k24>, "error out"=w2396:errorcluster)  [unwired: 10 in]
                }
                n848 = call "get 9V monitor voltage.vi"("error in (no error)"=w2373, "Descriptions"=w2377, "Array"=w2378, "Array 2"=w2374) -> ("error out"=w2372:errorcluster, "9V Voltage Monitor"=→"9V Voltage Monitor":dbl)  [unwired: 6 in]
                "DAQ Error" <- w2372
                n849 = flat-sequence {
                  tunnel: [w2392] -> w2371
                  tunnel: w2374 -> [w2390]
                  tunnel: w2372 -> [w2389]
                  frame #0 {
                    n850 = local read "Descriptions"() -> (w2393:string[])
                    n851 = call "Measure DAQ Voltages.vi"("error in (no error)"=w2389, "Descriptions"=w2393, "Array in"=w2390) -> ("Raw Voltages"=w2391:dbl[], "Array out"=w2392:refnum<k24>[], "Sensor Cluster"=w2388:T9)  [unwired: 6 in]
                    n852 = local write "Sensor Voltage Cluster"(w2388) -> ()
                    n853 = local write "Raw Voltages"(w2391) -> ()
                  }
                }
              }
            }
            n854 = local write "Initialization"(-1 ("Initialization")) -> ()
            n855 = disable-structure shown="Enabled" {
              disable-tunnel: [w2051 _] -> w2034
              disable-tunnel: w2033 -> [w2056 w2319]
              disable-tunnel: [w2055 w2319] -> w2032
              disable-tunnel: w2031 -> [w2054 _]
              disable-tunnel: w2030 -> [w2052 _]
              disable-tunnel: w2022 -> [w2049 _]
              disable-tunnel: [w2048 _] -> w2021
              frame Enabled {
                n856 = local read "Descriptions"() -> (w2053:string[])
                n857 = call <vilib>:"Clear Errors.vi"("error in (no error)"=w2054) -> ("error out"=w2050:errorcluster)  [unwired: 5 in, 1 out]
                n858 = stacked-sequence {
                  seq-local: [w2057 _ _ _ _ _ _ _ _ _ _] -> [_ w2086 _ _ _ _ _ _ _ _ _]
                  seq-local: [_ w2087 _ _ _ _ _ _ _ _ _] -> [_ _ w2113 _ _ _ _ _ _ _ _]
                  seq-local: [_ _ w2112 _ _ _ _ _ _ _ _] -> [_ _ _ _ _ _ _ _ _ _ w2310]
                  tunnel: [_ _ w2117 _ _ _ _ _ _ _ _] -> _
                  tunnel: [_ _ _ _ _ _ errorcluster {"status"=FALSE, "code"=0, "source"=""} ("error out") _ _ _ _] -> _
                  tunnel: w2056 -> [_ _ _ _ _ _ _ _ _ _ w2314]
                  tunnel: [_ _ _ _ _ _ _ _ _ _ w2313] -> w2055
                  tunnel: w2050 -> [w2059 _ _ _ _ _ _ _ _ _ _]
                  tunnel: w2052 -> [_ _ w2115 w2192 w2219 w2245 _ _ _ w2284 _]
                  tunnel: w2053 -> [_ _ w2114 w2193 w2218 w2244 _ _ _ w2282 _]
                  tunnel: [_ _ _ w2194 _ _ _ _ _ _ _] -> _
                  tunnel: [_ _ _ _ _ _ _ _ _ _ w2310] -> w2051
                  tunnel: w2049 -> [_ _ w2111 _ _ _ _ _ _ _ _]
                  tunnel: [_ _ w2110 _ _ _ _ _ _ _ _] -> w2048
                  frame #0 {
                    n859 = flat-sequence {
                      tunnel: [w2064] -> w2057
                      tunnel: w2059 -> [w2065]
                      frame #0 {
                        n860 = local read "Groundwater Header"() -> (w2071:T10)
                        n861 = Unbundle By Name(w2071) -> ("Kpro box Serial"=w2061:string)
                        n862 = Scan From String(format string="%d", input string=w2061, error in=w2065, default 1=800.0 ("default value 1")) -> (error out=w2066:errorcluster, output 1=w2070:dbl)  [unwired: 1 in, 2 out]
                        n863 = Equal?(x=w2061, y="") -> (x = y?=w2062:bool)
                        n864 = case shown="True" w2062 {
                          tunnel: "KPRO Box Number\n\nEnter the number of the KPRO box you are using." ("prompt") -> [_ w2085]
                          tunnel: w2071 -> [w2075 w2084]
                          tunnel: w2070 -> [w2073 w2083]
                          tunnel: [w2073 w2082] -> w2069
                          tunnel: [w2075 w2080] -> w2067
                          tunnel: w2066 -> [w2074 w2078]
                          tunnel: [w2074 w2077] -> w2064
                          frame False {
                          }
                          frame True {
                            n865 = call "prompt_and_enter_value2.vi"("prompt_IN"=w2085, "Enter value"=w2083) -> ("Numeric"=w2082:dbl)  [unwired: 9 in]
                            n866 = call <vilib>:"Clear Errors.vi"("error in (no error)"=w2078) -> ("error out"=w2076:errorcluster)  [unwired: 5 in, 1 out]
                            n867 = Format Into String(format string="%d", error in=w2076, w2082) -> (resulting string=w2079:string, error out=w2077:errorcluster)  [unwired: 1 in]
                            n868 = Bundle By Name(cluster=w2084, "Kpro box Serial"=w2079) -> (w2080:T10)
                          }
                        }
                        n869 = global write "Kpro Globals.vi" "KPRO Box Number"(w2069) -> ()
                        n870 = local write "Groundwater Header"(w2067) -> ()
                      }
                    }
                    "Initialization" <- 0
                  }
                  frame #1 {
                    n871 = local write "Initialization"(1 ("Initialization")) -> ()
                    n872 = flat-sequence {
                      tunnel: w2086 -> [w2094]
                      tunnel: [w2093] -> w2087
                      frame #0 {
                        n873 = local read "Groundwater Header"() -> (w2095:T10)
                        n874 = Build Array("Profile ID   " ("string"), "Depth    " ("string"), "Flow " ("string"), "Ik    " ("string")) -> (w2098:string[])
                        n875 = Unbundle By Name(w2095) -> ("Profile ID"=w2091:string)
                        n876 = call-poly <vilib>:"Write Delimited Spreadsheet.vi"("file path (dialog if empty)"="Static IK path", "1D data"=w2098, "append to file? (new file:F)"=TRUE, "error in (no error)"=w2094, "delimiter (\\t)"="," ("delimiter (\\t)")) -> ("error out"=w2093:errorcluster)  [unwired: 9 in, 1 out]
                        n877 = Equal?(x=w2091, y="") -> ()  [unwired: 1 out]
                        n878 = case shown="True" TRUE {
                          tunnel: "Profile ID\n\nEnter the profile ID" ("prompt") -> [_ w2109]
                          tunnel: [w2106 w2108] -> w2096
                          tunnel: w2091 -> [w2106 w2107]
                          frame False {
                          }
                          frame True {
                            n879 = call "prompt_string.vi"("prompt_IN"=w2109, "Enter value"=w2107) -> ("String"=w2108:string)  [unwired: 9 in]
                            n880 = global write "Kpro Globals.vi" "Profile ID"(w2108) -> ()
                          }
                        }
                        n881 = Bundle By Name(cluster=w2095, "Profile ID"=w2096) -> (w2097:T10)
                        n882 = local write "Groundwater Header"(w2097) -> ()
                      }
                    }
                  }
                  frame #2 {
                    n883 = flat-sequence {
                      tunnel: [w2138] -> w2117
                      tunnel: w2113 -> [w2145]
                      tunnel: w2115 -> [w2143]
                      tunnel: w2114 -> [w2142]
                      tunnel: [w2120] -> w2112
                      tunnel: w2111 -> [w2119]
                      tunnel: [w2118] -> w2110
                      frame #0 {
                        w2136 = "_KPRO.csv"
                        n884 = local read "Input Variables and Slopes"() -> (w2149:T11)
                        n885 = call <vilib>:"Clear Errors.vi"("error in (no error)"=w2145) -> ("error out"=w2121:errorcluster)  [unwired: 5 in, 1 out]
                        n886 = local read "Temporary Data Files Directory"() -> (w2144:path)
                        n887 = Unbundle By Name(w2149) -> ("Up Hole Pressure Slope"=w2152:dbl, "String Pot Slope"=w2151:dbl, "Flow Slope"=w2150:dbl)
                        n888 = call "FILE_DIALOG 2016.vi"("flow_slope_IN"=w2150, "pressure_slope_IN"=w2152, "string_pot_slope_IN"=w2151, "Descriptions"=w2142, "error in (no error)"=w2121, "start path"=w2144, "Array in"=w2143) -> ("path"=w2131:path, "exists"=w2141:bool, "flow_slope_OUT"=w2147:dbl, "pressure_slope_OUT"=w2146:dbl, "string_pot_slope_OUT"=w2148:dbl, "error out"=w2137:errorcluster)  [unwired: 5 in, 2 out]
                        n889 = global write "Kpro Globals.vi" "Flow Slope"(w2147) -> ()
                        n890 = Bundle By Name(cluster=w2149, "String Pot Slope"=w2148, "Flow Slope"=w2147, "Up Hole Pressure Slope"=w2146) -> (w2139:T11)
                        n891 = global write "Kpro Globals.vi" "Pressure \nSlope"(w2146) -> ()
                        n892 = global write "Kpro Globals.vi" "String Pot \nSlope"(w2148) -> ()
                        n893 = Path To String(path=w2131) -> (string=w2133:string)
                        n894 = call-poly "Strip Path Extension__ogtk.vi"("path"=w2131) -> ("root"=w2132:string, "extension"=w2130:string)
                        n895 = Match Pattern(string=w2133, regular expression=w2136) -> (offset past match=w2135:i32)  [unwired: 1 in, 3 out]
                        n896 = String Length(string=w2130) -> (length=w2129:i32)
                        n897 = Equal?(x=w2135, y=-1) -> (x = y?=w2127:bool)
                        n898 = Equal To 0?(x=w2129) -> (x = 0?=w2128:bool)
                        n899 = local write "Input Variables and Slopes"(w2139) -> ()
                        n900 = Or(x=w2127, y=w2128) -> (x .or. y?=w2126:bool)
                        n901 = case shown="True" w2126 {
                          tunnel: [w2153 w2159] -> w2140
                          tunnel: w2132 -> [_ w2157]
                          tunnel: w2136 -> [_ w2158]
                          tunnel: w2131 -> [w2153 _]
                          tunnel: [w2153 w2154] -> w2122
                          frame False {
                          }
                          frame True {
                            n902 = Concatenate Strings(w2157, ".csv" ("string")) -> (w2155:string)
                            n903 = Concatenate Strings(w2157, w2158) -> (w2160:string)
                            n904 = String To Path(string=w2155) -> (path=w2154:path)
                            n905 = String To Path(string=w2160) -> (path=w2159:path)
                          }
                        }
                        "Output File Path" <- w2122
                        "KPRO Output File Path" <- w2140
                        n906 = call <vilib>:"Check if File or Folder Exists.vi"("path"=w2140) -> ("file or folder exists?"=w2123:bool, "dup path"=w2125:path)  [unwired: 8 in, 1 out]
                        n907 = And(x=w2123, y=w2141) -> (x .and. y?=w2124:bool)
                        n908 = case shown="True" w2124 {
                          selector: w2124 -> [_ w2167]
                          tunnel: w2125 -> [_ w2178]
                          tunnel: w2139 -> [w2163 w2173]
                          tunnel: [w2163 w2172] -> w2138
                          tunnel: w2137 -> [w2162 w2168]
                          tunnel: [w2162 w2168] -> w2120
                          tunnel: w2119 -> [w2161 w2166]
                          tunnel: [w2161 w2165] -> w2118
                          frame False {
                          }
                          frame True {
                            n909 = local read "Culmulative Graph Cluster"() -> (w2177:T19)
                            n910 = call "Get_KPRO_data_from_file 2016.vi"("Output File KPRO Test"=w2178) -> ("Last_height_of_box"=w2170:dbl, "Last_depth_to_water"=w2171:dbl, "Last_depth"=w2169:dbl, "Output_array"=w2164:sgl[][])  [unwired: 7 in]
                            "Cumulative_data_from_file" <- w2164
                            n911 = Bundle By Name(cluster=w2173, "Depth to Water Table"=w2171, "Height of Sample Box"=w2170) -> (w2172:T11)
                            n912 = Bundle By Name(cluster=w2166, "Absolute Depth In"=w2169, "Current Absolute Depth"=w2169) -> (w2165:T17)
                            n913 = call "Array to Plot 2016.vi"("Input Cumulative Array"=w2164) -> ("Cumulative - Depth vs.Drive Rate"=w2174:cluster{dbl[], dbl[]}, "Cumulative - Depth vs. Ik"=w2175:cluster{dbl[], dbl[]})  [unwired: 3 in, 4 out]
                            n914 = Bundle By Name(cluster=w2177, "Cumulative - Depth vs. Ik"=w2175, "Cumulative - Depth vs. Drive Rate"=w2174) -> (w2176:T19)
                            n915 = local write "Culmulative Graph Cluster"(w2176) -> ()
                            n916 = local write "Input Variables and Slopes"(w2172) -> ()
                            "Cumulative_data_ready" <- w2167
                          }
                        }
                      }
                    }
                    n917 = local write "Initialization"(2 ("Initialization")) -> ()
                  }
                  frame #3 {
                    # "Take offset and put\n into Pressure VI."
                    n918 = local read "Groundwater Header"() -> (w2184:T10)
                    n919 = local write "Initialization"(3 ("Initialization")) -> ()
                    n920 = local read "Input Variables and Slopes"() -> (w2182:T11)
                    n921 = Unbundle By Name(w2184) -> ("Atmospheric Pressure"=w2181:string)
                    n922 = case shown="True" TRUE {
                      tunnel: "ATMOSPHERIC PRESSURE READING\n\nHold Kpro effluent facing up and level with the pressure transducer.\nTurn on Kpro water, turn off when water flows with no air bubbles.\n\nPress OK when the reading equilibrates." ("message") -> [_ w2217]
                      tunnel: [w2208 w2216] -> w2199
                      tunnel: [w2207 w2209] -> w2196
                      tunnel: w2193 -> [_ w2215]
                      tunnel: w2192 -> [w2205 w2214]
                      tunnel: [w2206 w2213] -> w2191
                      tunnel: [w2202 w2211] -> w2186
                      tunnel: [w2205 w2210] -> w2185
                      tunnel: w2182 -> [w2207 w2209]
                      tunnel: w2181 -> [w2203 _]
                      frame False {
                        n923 = local read "Sensor Voltage Cluster"() -> (w2208:T9)
                        n924 = Unbundle By Name(w2207) -> ("Up Hole Pressure Slope"=w2206:dbl)
                        n925 = Scan From String(input string=w2203, default 1=35.0 ("default value 1")) -> (output 1=w2202:dbl)  [unwired: 3 in, 3 out]
                      }
                      frame True {
                        n926 = local read "Sensor Voltage Cluster"() -> (w2216:T9)
                        n927 = Unbundle By Name(w2209) -> ("Up Hole Pressure Slope"=w2213:dbl)
                        n928 = global read "Kpro Globals.vi" "Pressure Offset"() -> (w2212:dbl)
                        "Pressure Offset" <- w2212
                        n929 = call "Up Hole PRESSURE_CAL 2016.vi"("Pressure Offset"=w2212, "Descriptions"=w2215, "Array in"=w2214, "Pressure \nSlope"=w2213, "Sensor Cluster"=w2216, "Prompt_IN"=w2217) -> ("PRESSURE\nFt of water"=w2211:dbl, "Array out"=w2210:refnum<k24>[])  [unwired: 4 in]
                      }
                    }
                    n930 = Equal?(x=w2181, y="") -> ()  [unwired: 1 out]
                    n931 = local read "Corrected Pressure Cluster"() -> (w2198:T20)
                    n932 = global write "Kpro Globals.vi" "Atmospheric Pressure"(w2186) -> ()
                    n933 = Bundle By Name(cluster=w2196, "Atmospheric Pressure"=w2186) -> (w2195:T11)
                    n934 = Format Into String(w2186) -> (resulting string=w2187:string)  [unwired: 3 in, 1 out]
                    n935 = call "up hole Pressure 2016.vi"("Sensor Cluster"=w2199, "Pressure Offset"=w2186, "Array in"=w2185, "Pressure \nSlope"=w2191, "Descriptions"=w2193, "Zero Pressure\n(F = leave as is)"=TRUE) -> ("Array out"=w2194:refnum<k24>[], "Uphole Pressure"=w2179:dbl, "Sensor Cluster 2"=w2189:T9)  [unwired: 7 in]
                    n936 = Bundle By Name(cluster=w2184, "Atmospheric Pressure"=w2187) -> (w2188:T10)
                    n937 = Bundle By Name(cluster=w2198, "Up hole Corrected Pressure"=w2179) -> (w2197:T20)
                    n938 = local write "Sensor Voltage Cluster"(w2189) -> ()
                    n939 = local write "Input Variables and Slopes"(w2195) -> ()
                    n940 = local write "Groundwater Header"(w2188) -> ()
                    n941 = local write "Corrected Pressure Cluster"(w2197) -> ()
                    n942 = local write "Uphole Pressure"(w2179) -> ()
                  }
                  frame #4 {
                    n943 = disable-structure shown="Disabled" {
                      disable-tunnel: w2219 -> [w2223 _]
                      disable-tunnel: w2218 -> [w2222 _]
                      frame Disabled {
                        w2231 = 0.0  # Offset
                        (unwired) FALSE
                        # "Take offset and put\n into Pressure VI."
                        n944 = local write "Initialization"(4 ("Initialization")) -> ()
                        n945 = local read "Input Variables and Slopes"() -> (w2230:T11)
                        n946 = local read "Input Variables and Slopes"() -> (w2237:T11)
                        n947 = local read "Input Variables and Slopes"() -> (w2229:T11)
                        n948 = local read "Input Variables and Slopes"() -> (w2228:T11)
                        n949 = local read "Sensor Voltage Cluster"() -> (w2233:T9)
                        n950 = Unbundle By Name(w2230) -> ()  [unwired: 2 out]
                        n951 = Unbundle By Name(w2233) -> ()  [unwired: 1 out]
                        n952 = Unbundle By Name(w2237) -> ("Up Hole Pressure Slope"=w2224:dbl, "Flow Slope"=w2232:dbl)
                        n953 = Unbundle By Name(w2229) -> ()  [unwired: 2 out]
                        n954 = Unbundle By Name(w2228) -> ()  [unwired: 2 out]
                        n955 = call "Up Hole PRESSURE_CAL 2016.vi"("Descriptions"=w2222, "Array in"=w2223, "Pressure \nSlope"=w2224, "Sensor Cluster"=w2233, "Prompt_IN"="ZERO PRESSURE TRANSDUCER\n\nHold Kpro effluent in a grad cylinder with 800mL (1 ft) of water.\nHold grad cylinder with its bottom level with the pressure transducer.\n\nPress OK when the reading equilibrates. " ("message")) -> ("PRESSURE\nFt of water"=w2238:dbl)  [unwired: 5 in, 1 out]
                        n956 = call "Flow 2016.vi"("Descriptions"=w2222, "Array in"=w2223, "Flow Slope"=w2232, "Offset"=w2231) -> ("Flow (ml/min)"=w2225:dbl)  [unwired: 4 in, 2 out]
                        n957 = local read item#-1() -> (w2227)
                        n958 = Subtract(x=w2238, y=1.0) -> (x-y=w2241:dbl)
                        n959 = Bundle By Name(cluster=w2227, "Flow"=w2225) -> (w2226:cluster{})
                        n960 = call "up hole Pressure 2016.vi"("Sensor Cluster"=w2233, "Pressure Offset"=w2241, "Array in"=w2223, "Pressure \nSlope"=w2224, "Descriptions"=w2222, "Zero Pressure\n(F = leave as is)"=TRUE) -> ("Uphole Pressure"=w2234:dbl, "Sensor Cluster 2"=w2220:T9)  [unwired: 7 in, 1 out]
                        n961 = local write "Sensor Voltage Cluster"(w2220) -> ()
                        n962 = local write item#-1(w2226) -> ()
                        n963 = local read "Corrected Pressure Cluster"() -> (w2236:T20)
                        n964 = Bundle By Name(cluster=w2236, "Up hole Corrected Pressure"=w2234) -> (w2235:T20)
                        n965 = local write "Corrected Pressure Cluster"(w2235) -> ()
                      }
                      frame Enabled {
                      }
                    }
                  }
                  frame #5 {
                    n966 = local write "Initialization"(5 ("Initialization")) -> ()
                    n967 = flat-sequence {
                      tunnel: w2245 -> [w2254]
                      tunnel: w2244 -> [w2253]
                      frame #0 {
                        n968 = local read "Input Variables and Slopes"() -> (w2252:T11)
                        n969 = Unbundle By Name(w2252) -> ("Up Hole Pressure Slope"=w2251:dbl)
                        n970 = local read "Sensor Voltage Cluster"() -> (w2257:T9)
                        n971 = global read "Kpro Globals.vi" "Pressure Offset"() -> (w2250:dbl)
                        n972 = call "Up Hole PRESSURE_CAL 2016.vi"("Pressure Offset"=w2250, "Descriptions"=w2253, "Array in"=w2254, "Pressure \nSlope"=w2251, "Sensor Cluster"=w2257, "Prompt_IN"="CHECK RESERVOIR PRESSURE\n\nTurn on Kpro. Unplug Kpro Out quick connect from sample box.\nReservoir pressure should be 69.2 +/- 5%(65.7 - 72.7).\n\nPress OK when the reading equilibrates within range." ("message")) -> ("PRESSURE\nFt of water"=w2247:dbl)  [unwired: 4 in, 1 out]
                        n973 = local read "Groundwater Header"() -> (w2249:T10)
                        n974 = Format Into String(w2247) -> (resulting string=w2246:string)  [unwired: 3 in, 1 out]
                        n975 = global write "Kpro Globals.vi" "Reservoir Pressure"(w2247) -> ()
                        n976 = Bundle By Name(cluster=w2252, "Reservoir Pressure"=w2247) -> (w2255:T11)
                        n977 = Bundle By Name(cluster=w2249, "KPRO N2 Pressure"=w2246) -> (w2248:T10)
                        n978 = local write "Input Variables and Slopes"(w2255) -> ()
                        n979 = local write "Groundwater Header"(w2248) -> ()
                      }
                    }
                  }
                  frame #6 {
                    n980 = local write "Initialization"(6 ("Initialization")) -> ()
                    n981 = flat-sequence {
                      frame #0 {
                        n982 = local read "Input Depths \nand Parameters Cluster"() -> (w2263:T16)
                        n983 = Unbundle By Name(w2263) -> ("Start Depth"=w2260:sgl)
                        n984 = call "prompt_and_enter_value 2016.vi"("prompt_IN"="ENTER START DEPTH", "Enter value"=w2260) -> ("Numeric"=w2265:dbl)  [unwired: 9 in]
                        n985 = Absolute Value(x=w2265) -> (abs(x)=w2264:dbl)
                        n986 = Negate(x=w2264) -> (-x=w2261:dbl)
                        n987 = Bundle By Name(cluster=w2263, "Start Depth"=w2261) -> (w2262:T16)
                        n988 = local write "Input Depths \nand Parameters Cluster"(w2262) -> ()
                      }
                    }
                  }
                  frame #7 {
                    n989 = local write "Initialization"(7 ("Initialization")) -> ()
                    n990 = local read "Input Variables and Slopes"() -> (w2271:T11)
                    n991 = Unbundle By Name(w2271) -> ("Height of Sample Box"=w2269:dbl)
                    n992 = call "prompt_and_enter_value 2016.vi"("prompt_IN"="HEIGHT FROM GROUND SURFACE TO SAMPLE BOX\n\nMeasure the vertical distance between the ground surface and the pressure transducer." ("prompt"), "Enter value"=w2269) -> ("Numeric"=w2268:dbl)  [unwired: 9 in]
                    n993 = Bundle By Name(cluster=w2271, "Height of Sample Box"=w2268) -> (w2270:T11)
                    n994 = global write "Kpro Globals.vi" "height_of_box"(w2268) -> ()
                    n995 = local write "Input Variables and Slopes"(w2270) -> ()
                  }
                  frame #8 {
                    n996 = local write "Initialization"(8 ("Initialization")) -> ()
                    n997 = flat-sequence {
                      frame #0 {
                        n998 = local read "Input Variables and Slopes"() -> (w2276:T11)
                        n999 = Unbundle By Name(w2276) -> ("Depth to Water Table"=w2277:dbl)
                        n1000 = call "prompt_and_enter_value 2016.vi"("prompt_IN"="DEPTH TO WATER TABLE\n\nEnter the depth to the water table." ("prompt"), "Enter value"=w2277) -> ("Numeric"=w2279:dbl)  [unwired: 9 in]
                        n1001 = Absolute Value(x=w2279) -> (abs(x)=w2278:dbl)
                        n1002 = Negate(x=w2278) -> (-x=w2275:dbl)
                        n1003 = global write "Kpro Globals.vi" "Depth to Water Table"(w2275) -> ()
                        n1004 = Bundle By Name(cluster=w2276, "Depth to Water Table"=w2275) -> (w2274:T11)
                        n1005 = local write "Input Variables and Slopes"(w2274) -> ()
                      }
                    }
                  }
                  frame #9 {
                    n1006 = local write "Initialization"(9 ("Initialization")) -> ()
                    n1007 = local read "Input Variables and Slopes"() -> (w2285:T11)
                    n1008 = Unbundle By Name(w2285) -> ("Up Hole Pressure Slope"=w2283:dbl)
                    n1009 = stacked-sequence {
                      tunnel: [_ w2305] -> w2286
                      tunnel: w2283 -> [w2295 w2304]
                      tunnel: w2282 -> [w2290 w2303]
                      tunnel: w2284 -> [w2289 w2299]
                      tunnel: w2283 -> [_ w2302]
                      tunnel: w2282 -> [_ w2300]
                      frame #0 {
                        # "Set to raw pressure mode"
                        n1010 = local read "Sensor Voltage Cluster"() -> (w2294:T9)
                        n1011 = local read "Corrected Pressure Cluster"() -> (w2292:T20)
                        n1012 = call "up hole Pressure 2016.vi"("Sensor Cluster"=w2294, "Pressure Offset"=0.0, "Array in"=w2289, "Pressure \nSlope"=w2295, "Descriptions"=w2290, "Zero Pressure\n(F = leave as is)"=TRUE) -> ("Uphole Pressure"=w2293:dbl)  [unwired: 7 in, 2 out]
                        n1013 = Bundle By Name(cluster=w2292, "Up hole Corrected Pressure"=w2293) -> (w2291:T20)
                        n1014 = local write "Corrected Pressure Cluster"(w2291) -> ()
                      }
                      frame #1 {
                        # "adjust for 1 foot head"
                        # "Take offset and put\n into Pressure VI."
                        n1015 = local read "Sensor Voltage Cluster"() -> (w2306:T9)
                        n1016 = global read "Kpro Globals.vi" "Pressure Offset"() -> (w2301:dbl)
                        n1017 = call "Up Hole PRESSURE_CAL 2016.vi"("Pressure Offset"=w2301, "Descriptions"=w2300, "Array in"=w2299, "Pressure \nSlope"=w2302, "Sensor Cluster"=w2306, "Prompt_IN"="ZERO TO GROUND SURFACE\n\nFill a grad cylinder to 750mL.\nPlace it on the ground at the profile location.\nImmerse the Kpro effluent and turn on Kpro flow.\nTurn off after water is flowing with no bubbles\nand the water has reached 800mL (1 foot).\n\nPress OK when the reading equilibrates." ("message")) -> ("PRESSURE\nFt of water"=w2307:dbl)  [unwired: 4 in, 1 out]
                        n1018 = Decrement(x=w2307) -> (x-1=w2298:dbl)
                        n1019 = call "up hole Pressure 2016.vi"("Sensor Cluster"=w2306, "Pressure Offset"=w2298, "Array in"=w2299, "Pressure \nSlope"=w2304, "Descriptions"=w2303, "Zero Pressure\n(F = leave as is)"=TRUE) -> ("Uphole Pressure"=w2305:dbl)  [unwired: 7 in, 2 out]
                      }
                    }
                    n1020 = local read "Corrected Pressure Cluster"() -> (w2288:T20)
                    n1021 = Bundle By Name(cluster=w2288, "Up hole Corrected Pressure"=w2286) -> (w2287:T20)
                    n1022 = local write "Corrected Pressure Cluster"(w2287) -> ()
                  }
                  frame #10 {
                    n1023 = local write "Initialization"(10 ("Initialization")) -> ()
                    n1024 = local read "Cumulative_data_ready"() -> (w2315:bool)
                    n1025 = case shown="True" w2315 {
                      tunnel: w2314 -> [w2316 _]
                      tunnel: [w2316 w2317] -> w2313
                      frame False {
                      }
                      frame True {
                        n1026 = local write "Cumulative_data_ready"(FALSE ("Get_KPRO_data")) -> ()
                        n1027 = local read "Cumulative_data_from_file"() -> (w2317:sgl[][])
                      }
                    }
                    "Zero Pressure\nIndicator" <- FALSE ("Zero Pressure\nIndicator")
                  }
                }
              }
              frame Disabled {
              }
            }
            n1028 = flat-sequence {
              tunnel: w2031 -> [w2364]
              tunnel: [w2364] -> w2039
              frame #0 {
                w2365 = T23."Enabled" ("Disabled")
                n1029 = property on="Write Data to Spreadsheet" class="Bool"("DisabledEnum"=w2365) -> (error out=w2368:errorcluster)  [unwired: 2 in, 1 out]
                n1030 = property on="Record Continuous Samples" class="Bool"(error in=w2368, "DisabledEnum"=T23."Disabled and Grayed Out" ("Disabled")) -> (error out=w2367:errorcluster)  [unwired: 1 in, 1 out]
                n1031 = property on="Record Single Sample" class="Bool"(error in=w2367, "DisabledEnum"=w2365) -> (error out=w2366:errorcluster)  [unwired: 1 in, 1 out]
                n1032 = property on="Sample Not Collected" class="Bool"(error in=w2366, "DisabledEnum"=w2365) -> (error out=w2363:errorcluster)  [unwired: 1 in, 1 out]
                n1033 = invoke on="Sonde Data Array" class="Arr (strict)" method="Reinit To Default"(error in=w2363) -> ()  [unwired: 2 in, 3 out]
                "Initialization Finished" <- TRUE
              }
            }
            n1034 = flat-sequence {
              tunnel: "Read String Pot" -> [_]
              tunnel: [w2357] -> w2027
              tunnel: w2034 -> [w2341]
              tunnel: w2030 -> [w2342]
              frame #0 {
                w2347 = 0.0
                w2348 = TRUE
                # "Initialize Incrementer if using hand incrementer,\nDon't use Debug,\nPut use string pot into shift register first pass to avoid allowing\na change in which method is the source of the depth reading."
                n1035 = global write "Global_SIM_switch.vi" "enable_kpro_file"("enable_kpro_file") -> ()
                n1036 = global write "Global_SIM_switch.vi" "Simulate AD6B"("Simulate AD6B") -> ()
                n1037 = global write "Global_SIM_switch.vi" "enable_slug_file"("enable_slug_file") -> ()
                n1038 = local read "Input Variables and Slopes"() -> (w2355:T11)
                n1039 = global write "Global_SIM_switch.vi" "enable_IKMGS_file"("enable_IKMGS_file") -> ()
                n1040 = Unbundle By Name(w2355) -> ("String Pot Slope"=w2354:dbl, "Up Hole Pressure Slope"=w2350:dbl)  [unwired: 1 out]
                n1041 = local read "Sensor Voltage Cluster"() -> (w2349:T9)
                n1042 = local read "Descriptions"() -> (w2340:string[])
                n1043 = local read "Sensor Voltage Cluster"() -> (w2356:T9)
                n1044 = call "In-Line-Pressure 2016.vi"("Zero Pressure\n(F = leave as is)"=w2348, "In-Line Pressure Slope"=w2350, "Sensor Voltages Cluster"=w2349, "In-Line Pressure Offset"=w2347) -> ("Pressure"=w2351:dbl)  [unwired: 7 in]
                n1045 = call "up hole Pressure 2016.vi"("Sensor Cluster"=w2349, "Pressure Offset"=w2347, "Array in"=w2342, "Pressure \nSlope"=w2350, "Descriptions"=w2340, "Zero Pressure\n(F = leave as is)"=w2348) -> ("Array out"=w2339:refnum<k24>[], "Uphole Pressure"=w2336:dbl)  [unwired: 7 in, 1 out]
                n1046 = Bundle By Name(cluster="Corrected Pressure Cluster", "Up hole Corrected Pressure"=w2336, "Down hole Corrected Pressure"=w2351) -> (w2352:T20)
                n1047 = call "depth read from string pot 2016.vi"("Descriptions"=w2340, "error in (no error)"=w2341, "String Pot \nSlope"=w2354, "Array in"=w2339, "Sensor Cluster In"=w2356) -> ("Depth"=w2358:dbl)  [unwired: 11 in, 3 out]
                n1048 = local read "Sample Sheet Data Row Cluster 2"() -> (w2338:T2)
                n1049 = local write "Corrected Pressure Cluster"(w2352) -> ()
                n1050 = flat-sequence {
                  tunnel: w2358 -> [w2360]
                  tunnel: [w2359] -> w2357
                  frame #0 {
                    w2361 = 15  # Filter Size
                    # "Functional Global in \nBoxcar Integrator\nInitialize filter array to \ncurrent string pot value"
                    n1051 = call "Boxcar filter2016.vi"("Initialize"=TRUE, "Filter Size"=w2361, "Filter Input"=w2360) -> ("Filter Output"=w2359:dbl)
                  }
                }
                n1052 = Bundle By Name(cluster=w2338, "Head\nPressure"=w2336) -> (w2337:T2)
                n1053 = local write "Sample Sheet Data Row Cluster 2"(w2337) -> ()
              }
            }
            n1054 = flat-sequence {
              tunnel: [w2323] -> w2035
              tunnel: [w2322] -> w2028
              tunnel: w2027 -> [w2320]
              tunnel: [w2320] -> w2024
              frame #0 {
                n1055 = local read "Input Depths \nand Parameters Cluster"() -> (w2321:T16)
                n1056 = Unbundle By Name(w2321) -> ("Start Depth"=w2324:sgl)
                n1057 = Less Or Equal To 0?(x=w2324) -> (x <= 0?=w2326:bool)
                n1058 = Negate(x=w2324) -> (-x=w2325:sgl)
                n1059 = Select(t=w2324, s=w2326, f=w2325) -> (s? t:f=w2322:sgl)
                n1060 = Bundle By Name(cluster=w2321, "Abs Start Depth"=w2322, "Current Depth"=w2320) -> (w2323:T16)
                n1061 = local write "Input Depths \nand Parameters Cluster"(w2323) -> ()
              }
            }
            n1062 = flat-sequence {
              tunnel: [w2333] -> w2037
              frame #0 {
                n1063 = Tick Count (ms)() -> (millisecond timer value=w2335:u32)
                n1064 = Divide(x=w2335, y=u32 1000) -> (x/y=w2333:dbl)
              }
            }
            n1065 = flat-sequence {
              tunnel: [w2328] -> w2036
              tunnel: w2037 -> [w2331]
              tunnel: [w2330] -> _
              tunnel: w2028 -> [w2330]
              tunnel: w2024 -> [w2329]
              tunnel: w2021 -> [w2327]
              frame #0 {
                n1066 = Bundle By Name(cluster=w2327, "Absolute Depth In"=w2330, "Previous Relative Depth"=w2329, "Current Relative Depth"=w2329, "First Relative Depth"=w2329, "Current Absolute Depth"=w2330, "Last Filed Depth"=0.0, "Current Measurement Time"=w2331, "Previous Measurement Time"=w2331, "First Absolute Depth"=w2330) -> (w2328:T17)
              }
            }
          }
          frame "Acq. DAQ data" {
            n1067 = flat-sequence {
              tunnel: w2410 -> [w2427]
              tunnel: w2409 -> [w2426]
              tunnel: [w2423] -> w2408
              frame #0 {
                n1068 = local read "Descriptions"() -> (w2424:string[])
                n1069 = local read "Sensor  Real \nMeasurements"() -> (w2422:T6)
                n1070 = local read "Input Variables and Slopes"() -> (w2420:T11)
                n1071 = call "Measure DAQ Voltages.vi"("error in (no error)"=w2426, "Descriptions"=w2424, "Array in"=w2427) -> ("Raw Voltages"=→"Raw Voltages":dbl[], "Array out"=w2423:refnum<k24>[], "Sensor Cluster"=w2419:T9)  [unwired: 6 in]
                "Sensor Voltage Cluster" <- w2419
                n1072 = call "convert sensor voltage to real measurements.vi"("Input Variables and Slopes"=w2420, "Sensor  Real Measurements in"=w2422, "Sensor Cluster"=w2419) -> ("Sensor  Real Measurements out"=w2421:T9)  [unwired: 8 in]
                n1073 = local write "Sensor  Real \nMeasurements"(w2421) -> ()
              }
            }
          }
          frame "Exit" {
            n1074 = flat-sequence {
              tunnel: [w2456] -> _
              tunnel: [w2463] -> w2433
              tunnel: w2436 -> [w2458]
              tunnel: w2435 -> [w2456]
              tunnel: [w2455] -> w2434
              frame #0 {
                w2462 = "Groundwater Profile Log" ("Worksheet Name in")
                n1075 = local read "Worksheet Names"() -> (w2460:string[])
                n1076 = local write "Current Sample Sheet"(w2462) -> ()
                n1077 = call "find and open select worksheet.vi"("Worksheet Names"=w2460, "error in (no error)"=w2456, "milliseconds to wait"=u32 100, "Worksheet Name in"=w2462, "NI_report in"=w2458) -> ("error out"=w2459:errorcluster, "NI_report out"=w2457:refnum<class "NI_report.lvclass">)  [unwired: 4 in, 1 out]
                n1078 = call "groundwater log header.vi"("Worksheet Names"=w2460, "Groundwater Header"="Groundwater Header", "error in (no error)"=w2459, "NI_report in"=w2457) -> ("error out"=w2455:errorcluster, "NI_report out"=w2463:refnum<class "NI_report.lvclass">)  [unwired: 6 in]
              }
            }
            n1079 = case shown="No Error" w2444 {
              tunnel: w2440 -> [w2487 _]
              tunnel: w2444 -> [w2486 w2498]
              tunnel: [w2485 w2498] -> w2442
              frame No Error {
                n1080 = for {
                  shift-right: [w2489] -> w2485
                  shift-left: w2486 -> [w2490]
                  tunnel: w2487 -> [w2488] mode=indexing
                  n1081 = while {
                    shift-right: [w2497] -> w2492
                    shift-left: w2490 -> [w2495]
                    shift-right: [w2496] -> w2491
                    shift-left: w2488 -> [w2494]
                    stop <- w2493 stop-if-true
                    n1082 = call <vilib>:"ULx Is Task Done.vi"("task in"=w2494, "error in"=w2495) -> ("task out"=w2496:refnum<k24>, "task done?"=w2493:bool, "error out"=w2497:errorcluster)  [unwired: 11 in]
                  }
                  n1083 = call <vilib>:"ULx Clear Task.vi"("task in"=w2491, "error in"=w2492) -> ("error out"=w2489:errorcluster)  [unwired: 13 in]
                }
              }
              frame Error {
              }
            }
            n1084 = flat-sequence {
              tunnel: [w2504] -> w2451
              tunnel: [w2503] -> w2452
              tunnel: w2434 -> [w2501]
              tunnel: w2433 -> [w2500]
              frame #0 {
                n1085 = local read "Excel report file path"() -> (w2499:path)
                n1086 = call-dynamic "Save Report to File.vi"("report in"=w2500, "report file path"=w2499, "prompt to replace? (F)"=FALSE, "error in (no error)"=w2501) -> ("report out"=w2504:refnum<class "NI_report.lvclass">, "error out"=w2503:errorcluster)  [unwired: 10 in]
              }
            }
            n1087 = call "Wait (ms)__ogtk.vi"("error in (no error)"=w2452, "milliseconds to wait"=u32 5) -> ("error out"=w2453:errorcluster)  [unwired: 8 in, 1 out]
            n1088 = flat-sequence {
              tunnel: w2453 -> [w2473]
              tunnel: w2451 -> [w2471]
              tunnel: [w2469] -> w2445
              frame #0 {
                (unwired) FALSE ("Write Ini")
                n1089 = call-dynamic "Dispose Report.vi"("report in"=w2471, "save changes? (F)"=FALSE, "error in (no error)"=w2473) -> ("error out"=w2468:errorcluster)  [unwired: 12 in]
                n1090 = case shown="False" "Save Configuration File?" {
                  tunnel: [errorcluster {"status"=FALSE, "code"=0, "source"=""} ("error IO") w2482] -> w2470
                  frame False {
                  }
                  frame True {
                    n1091 = local read "Config File Path"() -> (w2481:path)
                    n1092 = call <vilib>:"Open Config Data.vi"("create file if necessary (T)"=TRUE ("Read Ini"), "configuration file path"=w2481) -> ("error out"=w2479:errorcluster, "refnum"=w2476:T22)  [unwired: 7 in, 1 out]
                    n1093 = control-ref of="This VI"() -> (w2475:refnum<vi>)
                    n1094 = call "Write Panel to INI__ogtk.vi"("error in (no error)"=w2479, "VI ref"=w2475, "refnum"=w2476) -> ("error out"=w2478:errorcluster, "refnum out"=w2477:T22)  [unwired: 7 in]
                    n1095 = call <vilib>:"Clear Errors.vi"("error in (no error)"=w2478) -> ("error out"=w2484:errorcluster)  [unwired: 5 in, 1 out]
                    n1096 = call <vilib>:"Close Config Data.vi"("error in (no error)"=w2484, "refnum"=w2477) -> ("error out"=w2483:errorcluster)  [unwired: 8 in, 1 out]
                    n1097 = Merge Errors(w2483, w2478) -> (w2482:errorcluster)
                  }
                }
                n1098 = Merge Errors(w2470, w2468) -> (w2469:errorcluster)
              }
            }
            n1099 = flat-sequence {
              tunnel: [TRUE ("aborted?")] -> w2443
              tunnel: [w2465] -> w2441
              tunnel: w2442 -> [w2465]
              frame #0 {
              }
            }
          }
        }
        n1100 = feedback-in #2(w421) -> ()
        n1101 = local write "Depth Cluster"(w424) -> ()
        "consumer loop" <- w430
      }
    }
  }
  n1102 = invoke on="IK Reason array" class="Arr (strict)" method="Reinit To Default"() -> ()  [unwired: 3 in, 3 out]
  n1103 = invoke on="Recording Reason Sonde array" class="Arr (strict)" method="Reinit To Default"() -> ()  [unwired: 3 in, 3 out]
  n1104 = Merge Errors(w17, w16) -> (→"error out":errorcluster)
